vi "Beampointing_Multi_TRA.vi"() -> ()   [LabVIEW 2013]
uses:
  GUI_Template/GUI_master/tcp_new_data_event.ctl
  GUI_Template/GUI_master/tcp new data cluster.ctl
  Ctrs/beam detection.ctl
  GUI_Beampointing_single_TRA/Ctrs/move.ctl
  <vilib>/Utility/file.llb/Read From Spreadsheet File (string).vi
  <userlib>/_OpenG.lib/array/array.llb/Filter 1D Array with Scalar (String)__ogtk.vi
  <vilib>/Utility/file.llb/Write To Spreadsheet File (string).vi
  <vilib>/Analysis/NI_AALBase.lvlib
panel:
  out "size(s) 3":i32[](array[numeric])
  out "size(s) 2":i32[](array[numeric])
  out "size(s)":i32[](array[numeric])
  out "Numeric 2":i32
  out "x-y*floor(x/y)":dbl
  out "config path":string
  out "motor refs 7":refnum<vi>[](array[refnum])
  out "Moving Y":string
  out "Moving X":string
  out "particles":T1(array[cluster])
  out "motor refs 6":refnum<vi>[](array[refnum])
  out "millisecond timer value":u32
  out "motor refs 5":refnum<vi>[](array[refnum])
  out "appended path":path
  out "motor refs 4":refnum<vi>[](array[refnum])
  in  "active Axis ref 3":cluster{"Ref X":refnum<vi>, "Ref Y":refnum<vi>}
  out "motor refs 3":refnum<vi>[](array[refnum])
  in  "active man refs":cluster{"Ref X":refnum<vi>, "Ref Y":refnum<vi>}
  out "motor refs 2":refnum<vi>[](array[refnum])
  in  "Numeric":dbl
  out "Current State":string
  in  "output cluster 2":T5 {"detection para"."smal para"."Measurement Parameter" items=["Center of Mass X", "Center of Mass Y", "First Pixel X", "First Pixel Y", "Bounding Rect Left", "Bounding Rect Top", "Bounding Rect Right", "Bounding Rect Bottom", "Max Feret Diameter Start X", "Max Feret Diameter Start Y", "Max Feret Diameter End X", "Max Feret Diameter End Y", "Max Horiz. Segment Length Left", "Max Horiz. Segment Length Right", "Max Horiz. Segment Length Row", "-", "Bounding Rect Width", "Bounding Rect Height", "Bounding Rect Diagonal", "Perimeter", "Convex Hull Perimeter", "Holes' Perimeter", "Max Feret Diameter", "Equivalent Ellipse Major Axis", "Equivalent Ellipse Minor Axis", "Equivalent Ellipse Minor Axis (Feret)", "Equivalent Rect Long Side", "Equivalent Rect Short Side", "Equivalent Rect Diagonal", "Equivalent Rect Short Side (Feret)", "Average Horiz. Segment Length", "Average Vert. Segment Length", "Hydraulic Radius", "Waddel Disk Diameter", "-", "Area", "Holes' Area", "Particle & Holes' Area", "Convex Hull Area", "Image Area", "-", "Number of Holes", "Number of Horiz. Segments", "Number of Vert. Segments", "-", "Orientation", "Max Feret Diameter Orientation", "-", "% Area/Image Area", "% Area/(Particle & Holes' Area)", "Ratio of Equivalent Ellipse Axes", "Ratio of Equivalent Rect Sides", "-", "Elongation Factor", "Compactness Factor", "Heywood Circularity Factor", "Type Factor", "-", "Sum X", "Sum Y", "Sum XX", "Sum XY", "Sum YY", "Sum XXX", "Sum XXY", "Sum XYY", "Sum YYY", "-", "Moment of Inertia XX", "Moment of Inertia XY", "Moment of Inertia YY", "Moment of Inertia XXX", "Moment of Inertia XXY", "Moment of Inertia XYY", "Moment of Inertia YYY", "Norm. Moment of Inertia XX", "Norm. Moment of Inertia XY", "Norm. Moment of Inertia YY", "Norm. Moment of Inertia XXX", "Norm. Moment of Inertia XXY", "Norm. Moment of Inertia XYY", "Norm. Moment of Inertia YYY", "Hu Moment 1", "Hu Moment 2", "Hu Moment 3", "Hu Moment 4", "Hu Moment 5", "Hu Moment 6", "Hu Moment 7"]; "detection para"."smal para"."Range Lower Value" format="%.2f"; "detection para"."smal para"."Range Upper Value" format="%.2f"; "detection para"."detection method" items=["clustering", "entropy", "metric", "moments", "inter-class variance"]; "detection para"."Filter" items=["No Filter", "Median Filter", "Low Pass Filter"]}
  out "CCDs":string[](array[string])
  in  "GUIdevice 12":string
  in  "GUIdevice 11":string
  in  "GUIdevice 10":string
  in  "GUIdevice 9":string
  out "error out 2":errorcluster
  in  "active cams":string[](array[string])
  in  "Motor Y":dbl[][](array[numeric])
  in  "Motor X":dbl[][](array[numeric])
  out "Names":string[](array[string])
  in  "Offset X stats":dbl[][](array[numeric])
  in  "Offset Y stats":dbl[][](array[numeric])
  out "Box":T6(array[cluster])
  in  "Tab Control 2":enum32{"Config ", "Main", "History"}(tab)=enum."Main"
  in  "associated motors":T7 {"Motor CCD 12" items=["M20", "SIM", "M22", ""]; "Motor CCD 11" items=["M20", "SIM", "M22", ""]; "Motor CCD 10" items=["M20", "SIM", "M22", ""]; "Motor CCD 9" items=["M20", "SIM", "M22", ""]; "Motor CCD 8" items=["M20", "SIM", "M22", ""]; "Motor CCD 7" items=["M20", "SIM", "M22", ""]; "Motor CCD 6" items=["M20", "SIM", "M22", ""]; "Motor CCD 5" items=["M20", "SIM", "M22", ""]; "Motor CCD 4" items=["M20", "SIM", "M22", ""]; "Motor CCD 3" items=["M20", "SIM", "M22", ""]; "Motor CCD 2" items=["M20", "SIM", "M22", ""]; "Motor CCD 1" items=["M20", "SIM", "M22", ""]}
  out "Cameras":T8
  out "Status":cluster{i32, i32, "Centroid X":dbl[][]}(graph)
  in  "Exposure:12":dbl=0.095 min=0.0001 max=1.0 format="%#_6f"
  in  "Triggerdelay::12":dbl=0.003 min=0.0 max=0.09 format="%#_6f"
  in  "Exposure::11":dbl=0.095 min=0.0001 max=1.0 format="%#_6f"
  in  "Triggerdelay::11":dbl=0.003 min=0.0 max=0.09 format="%#_6f"
  in  "Exposure::10":dbl=0.095 min=0.0001 max=1.0 format="%#_6f"
  in  "Triggerdelay::10":dbl=0.003 min=0.0 max=0.09 format="%#_6f"
  in  "Exposure::9":dbl=0.095 min=0.0001 max=1.0 format="%#_6f"
  in  "Triggerdelay::9":dbl=0.003 min=0.0 max=0.09 format="%#_6f"
  in  "Trigger::9":bool
  in  "Trigger::10":bool caption="Trigger:10"
  in  "Trigger::11":bool
  in  "Trigger::12":bool
  in  "Target.Y::9":dbl=45.0 caption="T9y" min=0.0 max=2000.0 format="%#_6f"
  in  "Target.X::9":dbl=47.0 caption="Tx9" min=0.0 max=2000.0 format="%#_6f"
  in  "Target.Y::10":dbl=45.0 caption="T10y" min=0.0 max=2000.0 format="%#_6f"
  in  "Target.X::10":dbl=47.0 caption="T10x" min=0.0 max=2000.0 format="%#_6f"
  in  "Target.Y::11":dbl=45.0 caption="T11y" min=0.0 max=2000.0 format="%#_6f"
  in  "Target.X::11":dbl=47.0 caption="T11x" min=0.0 max=2000.0 format="%#_6f"
  in  "Target.Y::12":dbl=45.0 caption="T12y" min=0.0 max=2000.0 format="%#_6f"
  in  "Target.X::12":dbl=47.0 caption="T12x" min=0.0 max=2000.0 format="%#_6f"
  in  "Exposure::8":dbl=0.095 min=0.0001 max=1.0 format="%#_6f"
  in  "Triggerdelay::8":dbl=0.003 min=0.0 max=0.09 format="%#_6f"
  in  "Trigger::8":bool
  in  "Target.Y::8":dbl=45.0 caption="T8y" min=0.0 max=2000.0 format="%#_6f"
  in  "Target.X::8":dbl=47.0 caption="T8x" min=0.0 max=2000.0 format="%#_6f"
  in  "Target.Y::7":dbl=45.0 caption="T7x" min=0.0 max=2000.0 format="%#_6f"
  in  "Target.X::7":dbl=47.0 caption="T7y" min=0.0 max=2000.0 format="%#_6f"
  in  "Target.Y::6":dbl=45.0 caption="T6y" min=0.0 max=5000.0 format="%#_6f"
  in  "Target.X::6":dbl=47.0 caption="T6x" min=0.0 max=5000.0 format="%#_6f"
  in  "Target.Y::5":dbl=45.0 caption="T5y" min=0.0 max=5000.0 format="%#_6f"
  in  "Target.X::5":dbl=47.0 caption="T5x" min=0.0 max=5000.0 format="%#_6f"
  in  "Target.Y::4":dbl=45.0 caption="T4y" min=0.0 max=5000.0 format="%#_6f"
  in  "Target.X::4":dbl=47.0 caption="T4x" min=0.0 max=5000.0 format="%#_6f"
  in  "Target.Y::3":dbl=163.0 caption="T3y" min=0.0 max=5000.0 format="%#_6f"
  in  "Target.X::3":dbl=152.0 caption="T3x" min=0.0 max=5000.0 format="%#_6f"
  in  "Target.Y::2":dbl=74.0 caption="T2y" min=0.0 max=5000.0 format="%#_6f"
  in  "Target.X::2":dbl=75.0 caption="T2x" min=0.0 max=5000.0 format="%#_6f"
  in  "Target.Y::1":dbl=61.0 caption="T1y" min=0.0 max=5000.0 format="%#_6f"
  in  "Target.X::1":dbl=77.0 caption="T1x" min=0.0 max=5000.0 format="%#_6f"
  in  "Exposure::7":dbl=0.095 min=0.0001 max=1.0 format="%#_6f"
  in  "Triggerdelay::7":dbl=0.003 min=0.0 max=0.09 format="%#_6f"
  in  "Trigger::7":bool
  in  "Exposure::6":dbl=0.095 min=0.0001 max=1.0 format="%#_6f"
  in  "Triggerdelay::6":dbl=0.003 min=0.0 max=0.09 format="%#_6f"
  in  "Trigger::6":bool
  in  "Exposure::5":dbl=0.095 min=0.0001 max=1.0 format="%#_6f"
  in  "Triggerdelay::5":dbl=0.003 min=0.0 max=0.09 format="%#_6f"
  in  "Trigger::5":bool
  in  "Exposure::4":dbl=0.095 min=0.0001 max=1.0 format="%#_6f"
  in  "Triggerdelay::4":dbl=0.003 min=0.0 max=0.09 format="%#_6f"
  in  "Trigger::4":bool
  in  "Exposure::3":dbl=0.095 min=0.0001 max=1.0 format="%#_6f"
  in  "Triggerdelay::3":dbl=0.003 min=0.0 max=0.09 format="%#_6f"
  in  "Trigger::3":bool
  in  "Exposure::2":dbl=0.095 min=0.0001 max=1.0 format="%#_6f"
  in  "Triggerdelay::2":dbl=0.003 min=0.0 max=0.09 format="%#_6f"
  in  "Trigger::2":bool
  out "image::1":T9(plugin-control) caption="RegenCam"
  out "image::2":T9(plugin-control) caption="BoosterCam"
  out "image::3":T9(plugin-control) caption="PreampCam"
  out "image::4":T9(plugin-control) caption="Amp1Cam"
  out "image::5":T9(plugin-control) caption="Amp2Cam"
  out "image::6":T9(plugin-control) caption="Amp3Cam"
  out "image::7":T9(plugin-control)
  out "image::8":T9(plugin-control)
  in  "Exposure::1":dbl=0.095 min=0.0001 max=1.0 format="%#_6f"
  in  "Triggerdelay::1":dbl=0.003 min=0.0 max=0.09 format="%#_6f"
  in  "Trigger::1":bool
  in  "UDP error message":string
  out "required Y":bool[](array[boolean])
  out "required X":bool[](array[boolean])
  out "detected":bool[](array[boolean])
  out "name array":string[](array[string])
  out "image::9":T9(plugin-control)
  out "image::10":T9(plugin-control)
  out "image::11":T9(plugin-control)
  out "image::12":T9(plugin-control)
  out "speedmode X":bool[](array[boolean])
  out "speedmode Y":bool[](array[boolean])
  out "CCD 9":cluster{timestamp[], dbl[]}[](graph)
  out "CCD 10":cluster{timestamp[], dbl[]}[](graph)
  out "CCD 11":cluster{timestamp[], dbl[]}[](graph)
  out "CCD 12":cluster{timestamp[], dbl[]}[](graph)
  out "CCD 5":cluster{timestamp[], dbl[]}[](graph)
  out "CCD 6":cluster{timestamp[], dbl[]}[](graph)
  out "CCD 7":cluster{timestamp[], dbl[]}[](graph)
  out "CCD 8":cluster{timestamp[], dbl[]}[](graph)
  out "CCD 2":cluster{timestamp[], dbl[]}[](graph)
  out "CCD 1":cluster{timestamp[], dbl[]}[](graph)
  out "CCD 3":cluster{timestamp[], dbl[]}[](graph)
  out "CCD 4":cluster{timestamp[], dbl[]}[](graph)
  in  "History Size":i32=500
  out "History Index":i32
  in  "Feedback Global":bool
  in  "detection para":T3[](array[typedef])=[{"Filter"=1, "Filter Para"={"X Size"=5, "Y Size"=5, "% Tolerance"=1}, "detection method"=4, "smal para"=[{"Measurement Parameter"=35, "Range Lower Value"=0.0, "Range Upper Value"=0.0, "Range"=TRUE, "Measurement Type"=FALSE}], "Remove small Objects"=TRUE, "Restrict to round Objects"=FALSE}, {"Filter"=1, "Filter Para"={"X Size"=5, "Y Size"=5, "% Tolerance"=1}, "detection method"=4, "smal para"=[{"Measurement Parameter"=35, "Range Lower Value"=0.0, "Range Upper Value"=500.0, "Range"=FALSE, "Measurement Type"=FALSE}], "Remove small Objects"=TRUE, "Restrict to round Objects"=FALSE}, {"Filter"=1, "Filter Para"={"X Size"=5, "Y Size"=5, "% Tolerance"=1}, "detection method"=4, "smal para"=[{"Measurement Parameter"=35, "Range Lower Value"=0.0, "Range Upper Value"=500.0, "Range"=TRUE, "Measurement Type"=FALSE}], "Remove small Objects"=TRUE, "Restrict to round Objects"=FALSE}, {"Filter"=1, "Filter Para"={"X Size"=5, "Y Size"=5, "% Tolerance"=1}, "detection method"=4, "smal para"=[{"Measurement Parameter"=35, "Range Lower Value"=0.0, "Range Upper Value"=500.0, "Range"=TRUE, "Measurement Type"=FALSE}], "Remove small Objects"=TRUE, "Restrict to round Objects"=FALSE}, {"Filter"=1, "Filter Para"={"X Size"=5, "Y Size"=5, "% Tolerance"=1}, "detection method"=4, "smal para"=[{"Measurement Parameter"=35, "Range Lower Value"=0.0, "Range Upper Value"=500.0, "Range"=TRUE, "Measurement Type"=FALSE}], "Remove small Objects"=TRUE, "Restrict to round Objects"=FALSE}, {"Filter"=1, "Filter Para"={"X Size"=5, "Y Size"=5, "% Tolerance"=1}, "detection method"=4, "smal para"=[{"Measurement Parameter"=35, "Range Lower Value"=0.0, "Range Upper Value"=500.0, "Range"=TRUE, "Measurement Type"=FALSE}], "Remove small Objects"=TRUE, "Restrict to round Objects"=FALSE}, {"Filter"=1, "Filter Para"={"X Size"=5, "Y Size"=5, "% Tolerance"=1}, "detection method"=4, "smal para"=[{"Measurement Parameter"=35, "Range Lower Value"=0.0, "Range Upper Value"=500.0, "Range"=TRUE, "Measurement Type"=FALSE}], "Remove small Objects"=TRUE, "Restrict to round Objects"=FALSE}, {"Filter"=1, "Filter Para"={"X Size"=5, "Y Size"=5, "% Tolerance"=1}, "detection method"=3, "smal para"=[{"Measurement Parameter"=35, "Range Lower Value"=0.0, "Range Upper Value"=0.0, "Range"=FALSE, "Measurement Type"=FALSE}], "Remove small Objects"=TRUE, "Restrict to round Objects"=FALSE}, {"Filter"=1, "Filter Para"={"X Size"=5, "Y Size"=5, "% Tolerance"=1}, "detection method"=4, "smal para"=[{"Measurement Parameter"=35, "Range Lower Value"=0.0, "Range Upper Value"=0.0, "Range"=FALSE, "Measurement Type"=FALSE}], "Remove small Objects"=TRUE, "Restrict to round Objects"=FALSE}, {"Filter"=1, "Filter Para"={"X Size"=5, "Y Size"=5, "% Tolerance"=1}, "detection method"=4, "smal para"=[{"Measurement Parameter"=35, "Range Lower Value"=0.0, "Range Upper Value"=500.0, "Range"=TRUE, "Measurement Type"=FALSE}], "Remove small Objects"=TRUE, "Restrict to round Objects"=FALSE}, {"Filter"=1, "Filter Para"={"X Size"=5, "Y Size"=5, "% Tolerance"=1}, "detection method"=4, "smal para"=[{"Measurement Parameter"=35, "Range Lower Value"=0.0, "Range Upper Value"=500.0, "Range"=TRUE, "Measurement Type"=FALSE}], "Remove small Objects"=TRUE, "Restrict to round Objects"=FALSE}, {"Filter"=1, "Filter Para"={"X Size"=5, "Y Size"=5, "% Tolerance"=1}, "detection method"=4, "smal para"=[{"Measurement Parameter"=35, "Range Lower Value"=0.0, "Range Upper Value"=500.0, "Range"=TRUE, "Measurement Type"=FALSE}], "Remove small Objects"=TRUE, "Restrict to round Objects"=FALSE}] {"smal para"."Measurement Parameter" items=["Center of Mass X", "Center of Mass Y", "First Pixel X", "First Pixel Y", "Bounding Rect Left", "Bounding Rect Top", "Bounding Rect Right", "Bounding Rect Bottom", "Max Feret Diameter Start X", "Max Feret Diameter Start Y", "Max Feret Diameter End X", "Max Feret Diameter End Y", "Max Horiz. Segment Length Left", "Max Horiz. Segment Length Right", "Max Horiz. Segment Length Row", "-", "Bounding Rect Width", "Bounding Rect Height", "Bounding Rect Diagonal", "Perimeter", "Convex Hull Perimeter", "Holes' Perimeter", "Max Feret Diameter", "Equivalent Ellipse Major Axis", "Equivalent Ellipse Minor Axis", "Equivalent Ellipse Minor Axis (Feret)", "Equivalent Rect Long Side", "Equivalent Rect Short Side", "Equivalent Rect Diagonal", "Equivalent Rect Short Side (Feret)", "Average Horiz. Segment Length", "Average Vert. Segment Length", "Hydraulic Radius", "Waddel Disk Diameter", "-", "Area", "Holes' Area", "Particle & Holes' Area", "Convex Hull Area", "Image Area", "-", "Number of Holes", "Number of Horiz. Segments", "Number of Vert. Segments", "-", "Orientation", "Max Feret Diameter Orientation", "-", "% Area/Image Area", "% Area/(Particle & Holes' Area)", "Ratio of Equivalent Ellipse Axes", "Ratio of Equivalent Rect Sides", "-", "Elongation Factor", "Compactness Factor", "Heywood Circularity Factor", "Type Factor", "-", "Sum X", "Sum Y", "Sum XX", "Sum XY", "Sum YY", "Sum XXX", "Sum XXY", "Sum XYY", "Sum YYY", "-", "Moment of Inertia XX", "Moment of Inertia XY", "Moment of Inertia YY", "Moment of Inertia XXX", "Moment of Inertia XXY", "Moment of Inertia XYY", "Moment of Inertia YYY", "Norm. Moment of Inertia XX", "Norm. Moment of Inertia XY", "Norm. Moment of Inertia YY", "Norm. Moment of Inertia XXX", "Norm. Moment of Inertia XXY", "Norm. Moment of Inertia XYY", "Norm. Moment of Inertia YYY", "Hu Moment 1", "Hu Moment 2", "Hu Moment 3", "Hu Moment 4", "Hu Moment 5", "Hu Moment 6", "Hu Moment 7"]; "smal para"."Range Lower Value" format="%.2f"; "smal para"."Range Upper Value" format="%.2f"; "detection method" items=["clustering", "entropy", "metric", "moments", "inter-class variance"]; "Filter" items=["No Filter", "Median Filter", "Low Pass Filter"]}
  in  "GUIdevice 8":string
  in  "Tab Control":T10(tab)=enum."Detection"
  in  "new tdms":bool
  in  "Save Stats":bool
  in  "Save Config":bool
  in  "Load Config":bool
  in  "update speed [ms]":i32=200
  in  "img to avg":i32=10
  in  "Reset History":bool
  in  "save path":path=path "W:/BP_DATA"
  in  "autodetect":bool
  in  "Detection Rate":dbl=0.9 min=0.001 max=1.0
  in  "Center":bool
  in  "Align":bool
  in  "Speedmode @":dbl=3.0 min=1.0 max=20.0
  in  "device ini":bool
  in  "beam detection para":T3={"Filter"=1, "Filter Para"={"X Size"=5, "Y Size"=5, "% Tolerance"=1}, "detection method"=4, "smal para"=[{"Measurement Parameter"=35, "Range Lower Value"=0.0, "Range Upper Value"=500.0, "Range"=FALSE, "Measurement Type"=FALSE}], "Remove small Objects"=TRUE, "Restrict to round Objects"=FALSE} {"smal para"."Measurement Parameter" items=["Center of Mass X", "Center of Mass Y", "First Pixel X", "First Pixel Y", "Bounding Rect Left", "Bounding Rect Top", "Bounding Rect Right", "Bounding Rect Bottom", "Max Feret Diameter Start X", "Max Feret Diameter Start Y", "Max Feret Diameter End X", "Max Feret Diameter End Y", "Max Horiz. Segment Length Left", "Max Horiz. Segment Length Right", "Max Horiz. Segment Length Row", "-", "Bounding Rect Width", "Bounding Rect Height", "Bounding Rect Diagonal", "Perimeter", "Convex Hull Perimeter", "Holes' Perimeter", "Max Feret Diameter", "Equivalent Ellipse Major Axis", "Equivalent Ellipse Minor Axis", "Equivalent Ellipse Minor Axis (Feret)", "Equivalent Rect Long Side", "Equivalent Rect Short Side", "Equivalent Rect Diagonal", "Equivalent Rect Short Side (Feret)", "Average Horiz. Segment Length", "Average Vert. Segment Length", "Hydraulic Radius", "Waddel Disk Diameter", "-", "Area", "Holes' Area", "Particle & Holes' Area", "Convex Hull Area", "Image Area", "-", "Number of Holes", "Number of Horiz. Segments", "Number of Vert. Segments", "-", "Orientation", "Max Feret Diameter Orientation", "-", "% Area/Image Area", "% Area/(Particle & Holes' Area)", "Ratio of Equivalent Ellipse Axes", "Ratio of Equivalent Rect Sides", "-", "Elongation Factor", "Compactness Factor", "Heywood Circularity Factor", "Type Factor", "-", "Sum X", "Sum Y", "Sum XX", "Sum XY", "Sum YY", "Sum XXX", "Sum XXY", "Sum XYY", "Sum YYY", "-", "Moment of Inertia XX", "Moment of Inertia XY", "Moment of Inertia YY", "Moment of Inertia XXX", "Moment of Inertia XXY", "Moment of Inertia XYY", "Moment of Inertia YYY", "Norm. Moment of Inertia XX", "Norm. Moment of Inertia XY", "Norm. Moment of Inertia YY", "Norm. Moment of Inertia XXX", "Norm. Moment of Inertia XXY", "Norm. Moment of Inertia XYY", "Norm. Moment of Inertia YYY", "Hu Moment 1", "Hu Moment 2", "Hu Moment 3", "Hu Moment 4", "Hu Moment 5", "Hu Moment 6", "Hu Moment 7"]; "smal para"."Range Lower Value" format="%.2f"; "smal para"."Range Upper Value" format="%.2f"; "detection method" items=["clustering", "entropy", "metric", "moments", "inter-class variance"]; "Filter" items=["No Filter", "Median Filter", "Low Pass Filter"]}
  in  "move config":T2={"Tolerance [%]"=0.1, "Stepsize"=0.0001, "Invert Axis"=TRUE, "Invert Direction X"=FALSE, "Invert Direction Y"=TRUE, "enable feedback"=FALSE, "Set Centriod Target"=FALSE}
  in  "Position 2":dbl=0.001 caption="Stepsize" min=0.0 max=999999.0 format="%_6f"
  in  "Position 1":dbl=0.001 caption="Stepsize" min=0.0 max=999999.0 format="%_6f"
  in  "Right":bool caption="RelativeMove.Axis 1.CCW::1"
  in  "Left":bool caption="RelativeMove.Axis 1.CW::1"
  in  "Down":bool caption="RelativeMove.Axis. 2.CCW::1"
  in  "Up":bool caption="RelativeMove.Axis 2.CW::1"
  in  "StepSize":dbl=0.001 caption="Stepsize" min=0.0 max=999999.0 format="%_1p"
  in  "active axis refs 2":T11(array[cluster])
  in  "active Axis ref":cluster{"Ref X":refnum<vi>, "Ref Y":refnum<vi>}
  in  "CCDs":u16(ring) items=["RegenCam", "BoosterCam", "PreampCam", "Amp1Cam", "Amp2Cam", "Amp3Cam", "", "", "", "", "", ""]
  out "motor refs":refnum<vi>[](array[refnum])
  in  "Position.Axis 4::99":dbl=77.0 caption="Motor Axis 1" min=0.0 max=6.0 format="%#_6f"
  in  "Position.Axis 5::99":dbl=77.0 caption="Motor Axis 1" min=0.0 max=6.0 format="%#_6f"
  in  "Position.Axis 6::99":dbl=77.0 caption="Motor Axis 1" min=0.0 max=6.0 format="%#_6f"
  in  "Position.Axis 3::99":dbl=77.0 caption="Motor Axis 1" min=0.0 max=6.0 format="%#_6f"
  in  "Position.Axis 2::99":dbl=77.0 caption="Motor Axis 1" min=0.0 max=6.0 format="%#_6f"
  in  "Position.Axis 1::99":dbl=77.0 caption="Motor Axis 1" min=0.0 max=6.0 format="%#_6f"
  in  "GUIdevice 99":string="TREX TRA1"
  in  "move properties":T2[](array[typedef])=[{"Tolerance [%]"=0.1, "Stepsize"=0.0001, "Invert Axis"=TRUE, "Invert Direction X"=FALSE, "Invert Direction Y"=TRUE, "enable feedback"=FALSE, "Set Centriod Target"=FALSE}, {"Tolerance [%]"=0.1, "Stepsize"=0.0001, "Invert Axis"=TRUE, "Invert Direction X"=FALSE, "Invert Direction Y"=TRUE, "enable feedback"=FALSE, "Set Centriod Target"=FALSE}, {"Tolerance [%]"=0.1, "Stepsize"=0.0001, "Invert Axis"=TRUE, "Invert Direction X"=FALSE, "Invert Direction Y"=TRUE, "enable feedback"=FALSE, "Set Centriod Target"=FALSE}, {"Tolerance [%]"=0.1, "Stepsize"=0.0001, "Invert Axis"=TRUE, "Invert Direction X"=FALSE, "Invert Direction Y"=TRUE, "enable feedback"=FALSE, "Set Centriod Target"=FALSE}, {"Tolerance [%]"=0.1, "Stepsize"=0.0001, "Invert Axis"=TRUE, "Invert Direction X"=FALSE, "Invert Direction Y"=TRUE, "enable feedback"=FALSE, "Set Centriod Target"=FALSE}, {"Tolerance [%]"=0.1, "Stepsize"=0.0001, "Invert Axis"=TRUE, "Invert Direction X"=FALSE, "Invert Direction Y"=TRUE, "enable feedback"=FALSE, "Set Centriod Target"=FALSE}, {"Tolerance [%]"=0.1, "Stepsize"=0.0001, "Invert Axis"=TRUE, "Invert Direction X"=FALSE, "Invert Direction Y"=TRUE, "enable feedback"=FALSE, "Set Centriod Target"=FALSE}, {"Tolerance [%]"=0.1, "Stepsize"=0.0001, "Invert Axis"=TRUE, "Invert Direction X"=FALSE, "Invert Direction Y"=TRUE, "enable feedback"=FALSE, "Set Centriod Target"=FALSE}, {"Tolerance [%]"=0.1, "Stepsize"=0.0001, "Invert Axis"=TRUE, "Invert Direction X"=FALSE, "Invert Direction Y"=TRUE, "enable feedback"=FALSE, "Set Centriod Target"=FALSE}, {"Tolerance [%]"=0.1, "Stepsize"=0.0001, "Invert Axis"=TRUE, "Invert Direction X"=FALSE, "Invert Direction Y"=TRUE, "enable feedback"=FALSE, "Set Centriod Target"=FALSE}, {"Tolerance [%]"=0.1, "Stepsize"=0.0001, "Invert Axis"=TRUE, "Invert Direction X"=FALSE, "Invert Direction Y"=TRUE, "enable feedback"=FALSE, "Set Centriod Target"=FALSE}, {"Tolerance [%]"=0.1, "Stepsize"=0.0001, "Invert Axis"=TRUE, "Invert Direction X"=FALSE, "Invert Direction Y"=TRUE, "enable feedback"=FALSE, "Set Centriod Target"=FALSE}, {"Tolerance [%]"=0.1, "Stepsize"=0.0001, "Invert Axis"=TRUE, "Invert Direction X"=FALSE, "Invert Direction Y"=TRUE, "enable feedback"=FALSE, "Set Centriod Target"=FALSE}]
  in  "Time":timestamp[][](array[timestamp])
  in  "Mean Size":dbl[][](array[numeric])
  in  "Size":dbl[][](array[numeric])
  in  "active CCDs":i32(listbox)
  in  "Offset Y":dbl[][](array[numeric])
  in  "Offset X":dbl[][](array[numeric])
  in  "Mean Centroid X":dbl[][](array[numeric])
  in  "Mean Centroid Y":dbl[][](array[numeric])
  in  "Centroid Y":dbl[][](array[numeric])
  in  "Centroid X":dbl[][](array[numeric])
  in  "GUIdevice 7":string
  in  "GUIdevice 6":string
  in  "GUIdevice 5":string
  in  "GUIdevice 4":string
  in  "GUIdevice 3":string="TargetCam10Hz_Diode"
  in  "GUIdevice 2":string="StagingM1Far"
  in  "insert tag":bool=TRUE
  in  "stop":bool
  in  "GUIdevice 1":string="StagingM1Near"
  out "tcp data event":T12
  out "error IO 2":errorcluster
  # "x [Tolerance]"
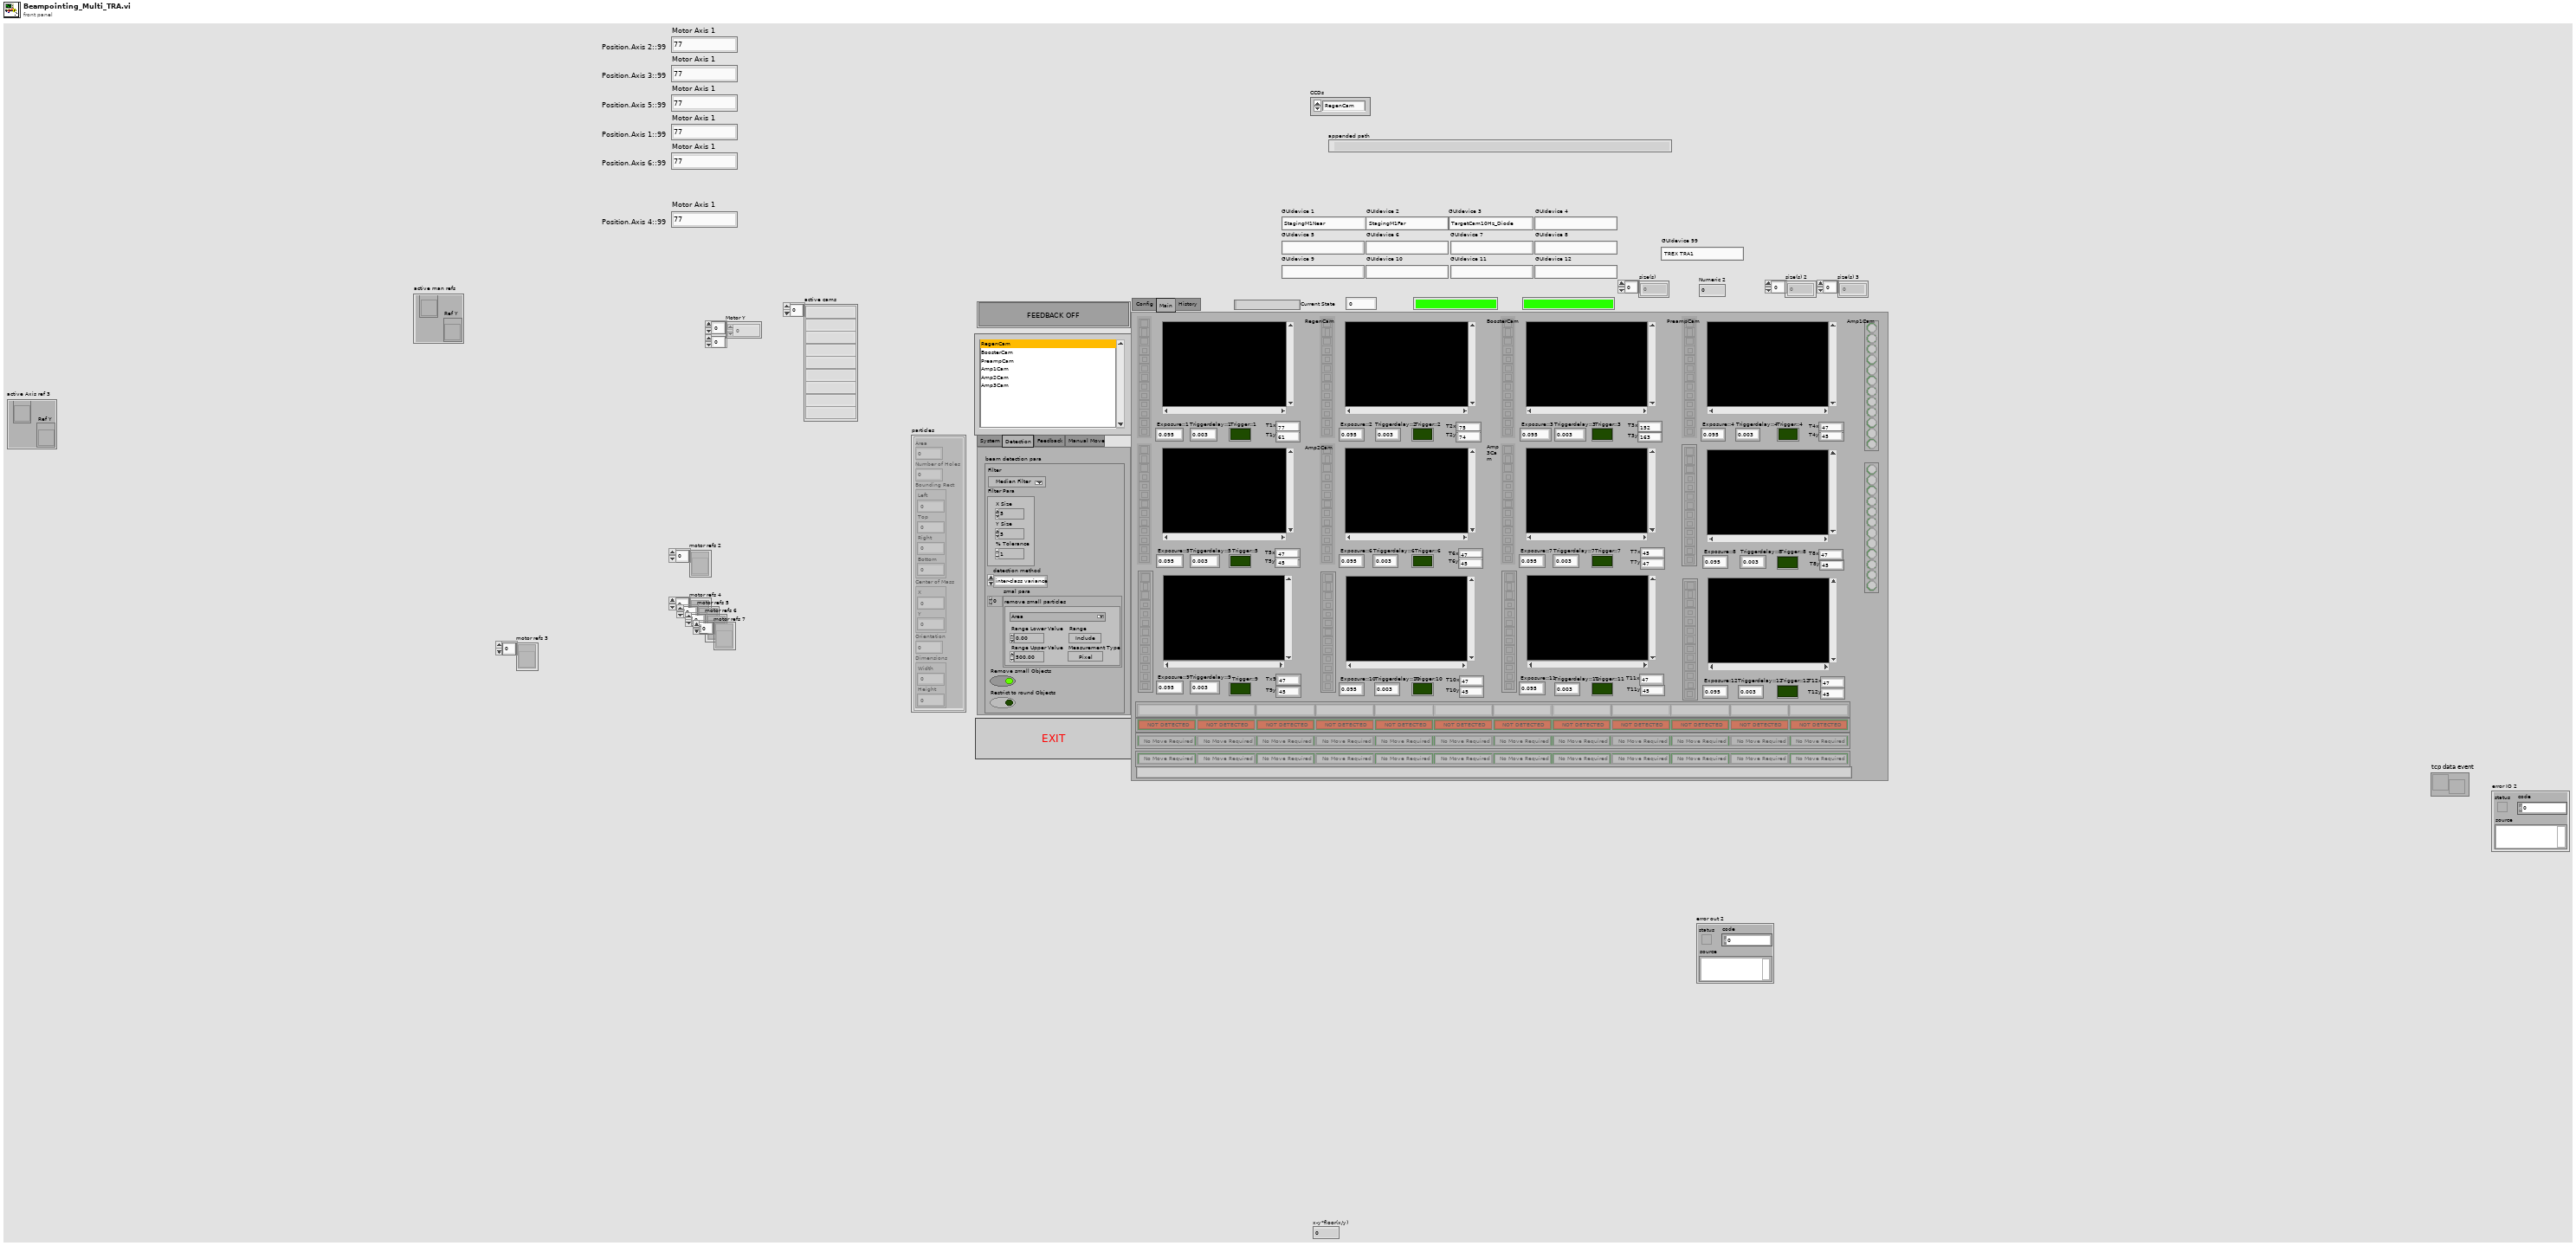
[diagram p1: front panel]
types:
  T1 = cluster{"Area":dbl, "Number of Holes":dbl, "Bounding Rect":cluster{"Left":dbl, "Top":dbl, "Right":dbl, "Bottom":dbl}, "Center of Mass":cluster{"X":dbl, "Y":dbl}, "Orientation":dbl, "Dimensions":cluster{"Width":dbl, "Height":dbl}}[]
  T2 = typedef "move.ctl" = cluster{"Tolerance [%]":dbl, "Stepsize":dbl, "Invert Axis":bool, "Invert Direction X":bool, "Invert Direction Y":bool, "enable feedback":bool, "Set Centriod Target":bool}
  T3 = typedef "beam detection.ctl" = cluster{"Filter":u16, "Filter Para":cluster{"X Size":i32, "Y Size":i32, "% Tolerance":i32}, "detection method":i32, "smal para":cluster{"Measurement Parameter":T4, "Range Lower Value":dbl, "Range Upper Value":dbl, "Range":bool, "Measurement Type":bool}[], "Remove small Objects":bool, "Restrict to round Objects":bool}
  T4 = typedef "Particle Parameters" = i32
  T5 = cluster{"CCDs":string[], "move properties":T2[], "detection para":T3[], "thresholds":cluster{"Lower value":sgl, "Upper value":sgl}[], "Value":cluster{"Motor CCD 1":u16, "Motor CCD 2":u16, "Motor CCD 3":u16, "Motor CCD 4":u16, "Motor CCD 5":u16, "Motor CCD 6":u16, "Motor CCD 7":u16, "Motor CCD 8":u16, "Motor CCD 9":u16, "Motor CCD 10":u16, "Motor CCD 11":u16, "Motor CCD 12":u16}}
  T6 = cluster{"Left":dbl, "Top":dbl, "Right":dbl, "Bottom":dbl}[]
  T7 = cluster{"Motor CCD 1":u16, "Motor CCD 2":u16, "Motor CCD 3":u16, "Motor CCD 4":u16, "Motor CCD 5":u16, "Motor CCD 6":u16, "Motor CCD 7":u16, "Motor CCD 8":u16, "Motor CCD 9":u16, "Motor CCD 10":u16, "Motor CCD 11":u16, "Motor CCD 12":u16}
  T8 = cluster{"[0]":string, "[1]":string, "[2]":string, "[3]":string, "[4]":string, "[5]":string, "[6]":string, "[7]":string, "[8]":string, "[8] 2":string, "[8] 3":string, "[8] 4":string}
  T9 = typedef "IMAQ Image.ctl" = refnum<image>
  T10 = enum32{"System", "Detection", "Feedback", "Manual Move"}
  T11 = cluster{"Ref X":refnum<vi>, "Ref Y":refnum<vi>}[]
  T12 = typedef "tcp_new_data_event.ctl" = refnum<user-event>
  T13 = typedef "tcp new data cluster.ctl" = cluster{"EventEnum":enum16{"new data", "connection status update"}, "Device name":string}
  T14 = cluster{"Left":i32, "Top":i32, "Right":i32, "Bottom":i32}
  T15 = enum32{"invalid app kind", "Development System", "Run Time System", "Student Edition", "Embedded LabVIEW", "Evaluation", "Custom"}
  T16 = enum16{"open", "open or create", "create or replace", "create", "open (read-only)"}
  T17 = enum32{"Invalid", "Standard", "Closed", "Hidden", "Minimized", "Maximized"}
  T18 = enum16{"open", "replace", "create", "open or create", "replace or create", "replace or create with confirmation"}
  T19 = enum8{"Enabled", "Disabled", "Disabled and Grayed Out"}
  T20 = typedef "Image Type" = u32
  T21 = cluster{"[0]":string, "[1]":string, "[2]":string, "[3]":string, "[4]":string, "[5]":string, "[6]":string, "[7]":string, "[8]":string, "[9]":string, "[10]":string, "[11]":string}
  T22 = cluster{"Target.X::1":refnum<vi>, "Target.Y::1":refnum<vi>}
  T23 = cluster{"Target.X::2":refnum<vi>, "Target.Y::2":refnum<vi>}
  T24 = cluster{"Target.X::3":refnum<vi>, "Target.Y::3":refnum<vi>}
  T25 = cluster{"Target.X::4":refnum<vi>, "Target.Y::4":refnum<vi>}
  T26 = cluster{"Target.X::5":refnum<vi>, "Target.Y::5":refnum<vi>}
  T27 = cluster{"Target.X::6":refnum<vi>, "Target.Y::6":refnum<vi>}
  T28 = cluster{"Target.X::7":refnum<vi>, "Target.Y::7":refnum<vi>}
  T29 = cluster{"Target.X::8":refnum<vi>, "Target.Y::8":refnum<vi>}
  T30 = cluster{"Target.X::12":refnum<vi>, "Target.Y::12":refnum<vi>}
  T31 = cluster{"Target.X::9":refnum<vi>, "Target.Y::9":refnum<vi>}
  T32 = cluster{"Target.X::10":refnum<vi>, "Target.Y::10":refnum<vi>}
  T33 = cluster{"Target.X::11":refnum<vi>, "Target.Y::11":refnum<vi>}
  T34 = cluster{"Target.X::12":refnum<vi>, "Target.Y::12":refnum<vi>}[]
  T35 = cluster{"Left":dbl, "Top":dbl, "Right":dbl, "Bottom":dbl}
  T36 = cluster{"Core":cluster{"Current VI Reference":refnum<vi>, "Close Panel on Exit?":bool}, "detection para":T3[], "thresholds":cluster{"Lower value":sgl, "Upper value":sgl}[], "Centroid X":dbl[][], "Centroid Y":dbl[][], "img to avg":i32, "Mean Centroid X":dbl[][], "Mean Centroid Y":dbl[][], "Offset X":dbl[][], "Offset Y":dbl[][], "Offset X stats ":dbl[][], "Offset Y stats ":dbl[][], "Size":dbl[][], "Mean Size":dbl[][], "Time":timestamp[][], "move properties":T2[], "active axis refs 2":cluster{"Ref X":refnum<vi>, "Ref Y":refnum<vi>}[], "active ccd":i32, "Feedback global":bool, "Motor X":dbl[][], "Motor Y":dbl[][], "active cams":string[], "Data Value Reference out":refnum<k34>, "active man refs":cluster{"Ref X":refnum<vi>, "Ref Y":refnum<vi>}, "speedmode X":bool[], "speedmode Y":bool[]}
  T37 = cluster{"Current VI Reference":refnum<vi>, "Close Panel on Exit?":bool}
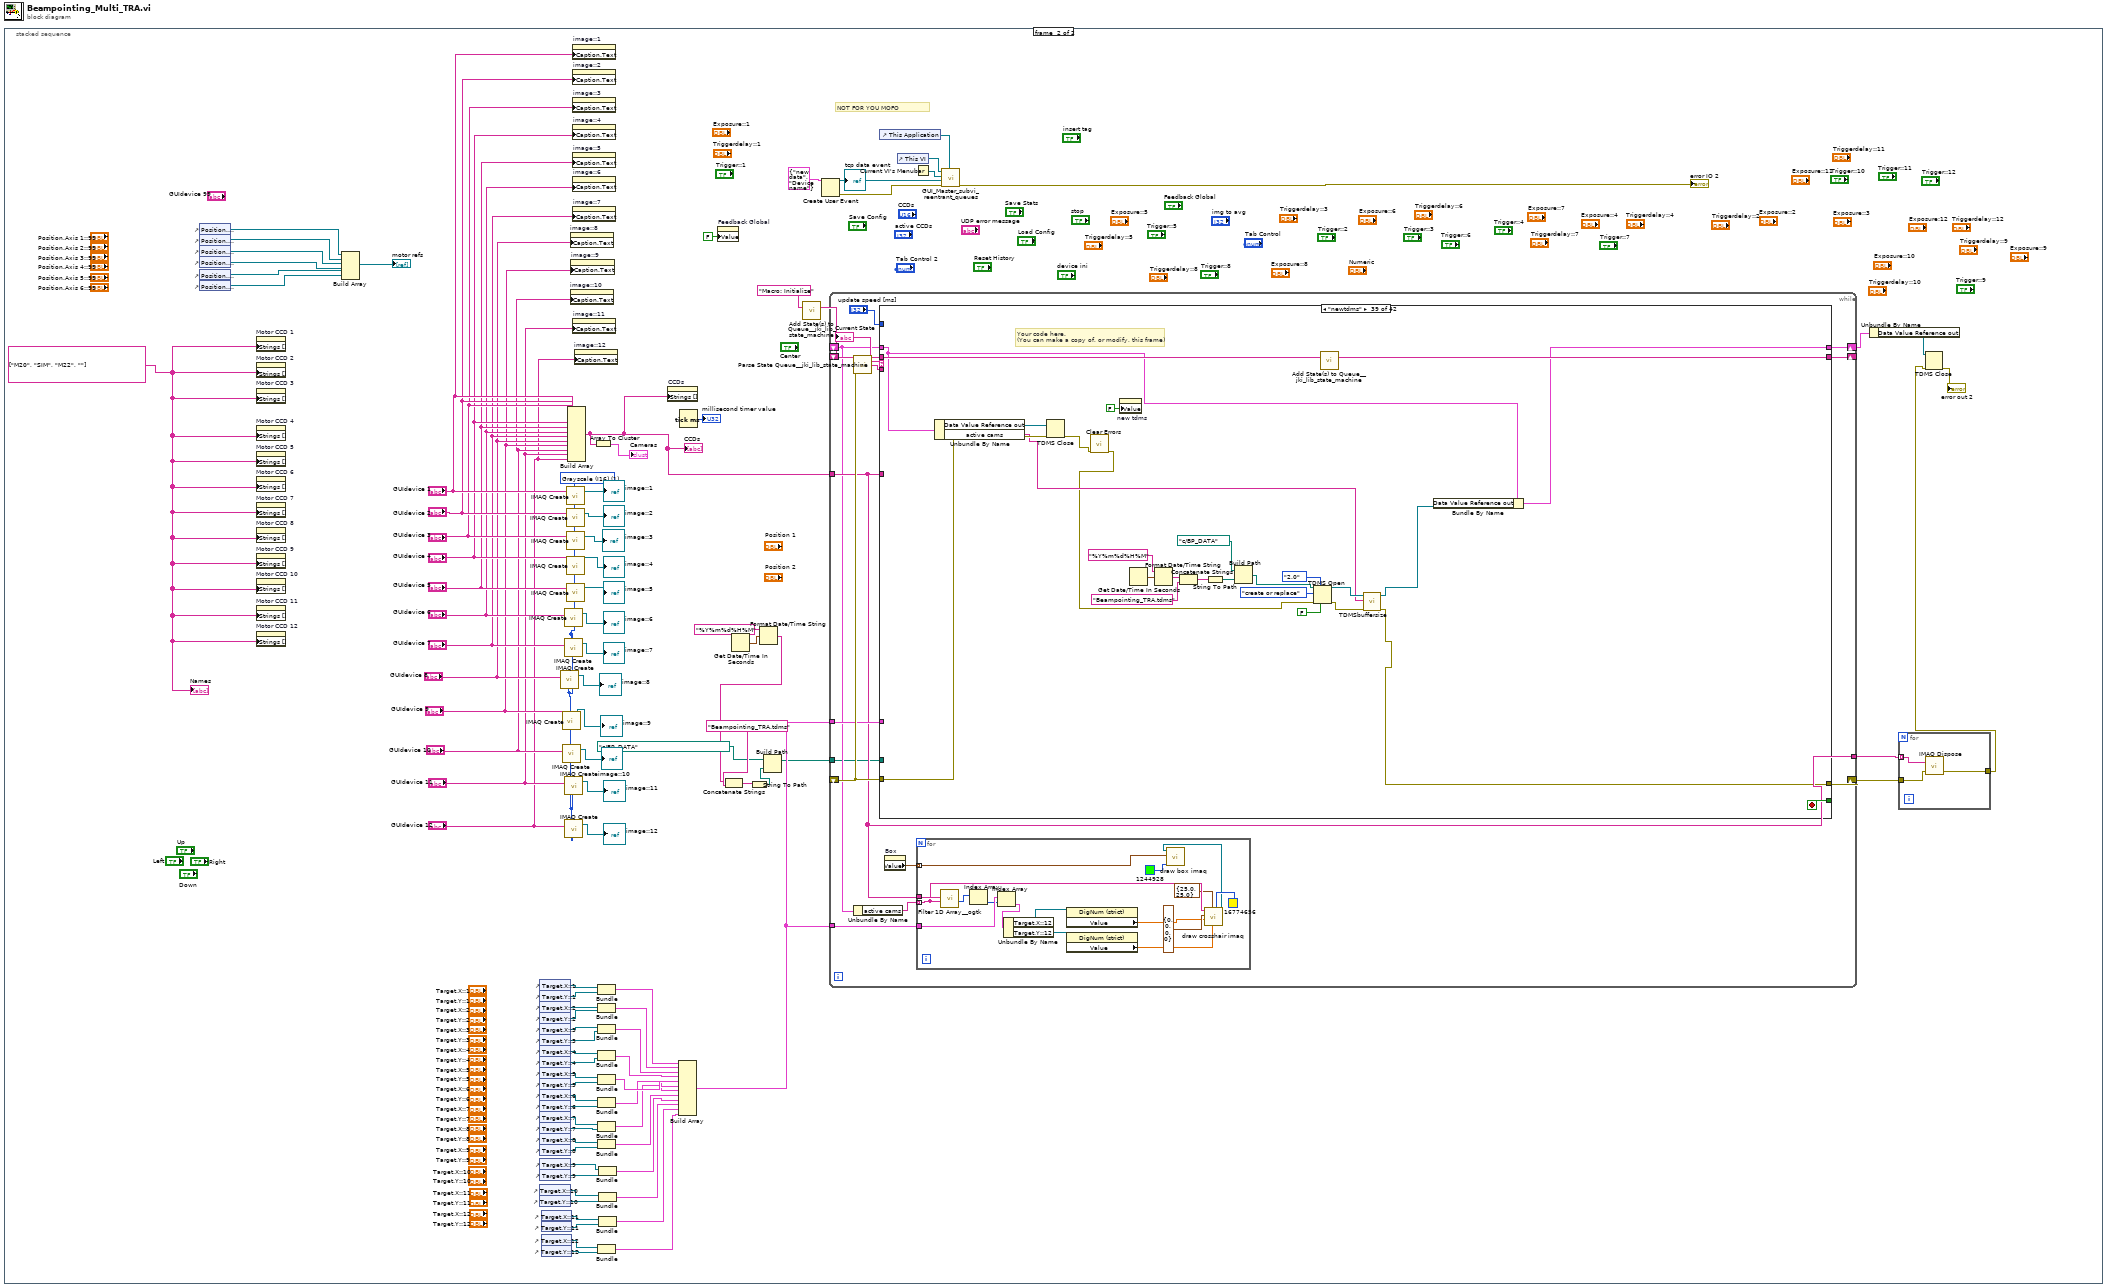
[diagram p0: block diagram]
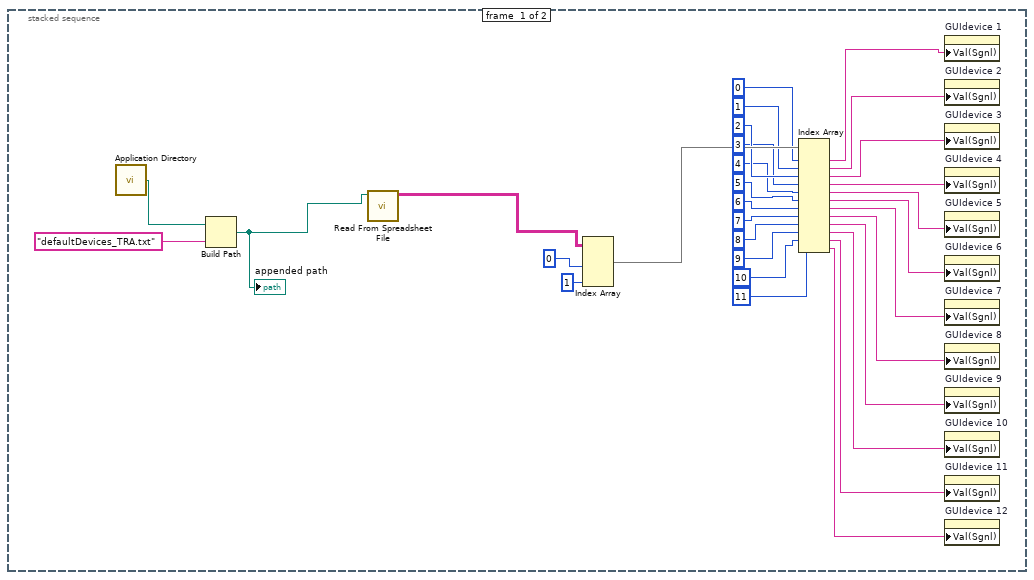
[diagram p2: hidden frame]
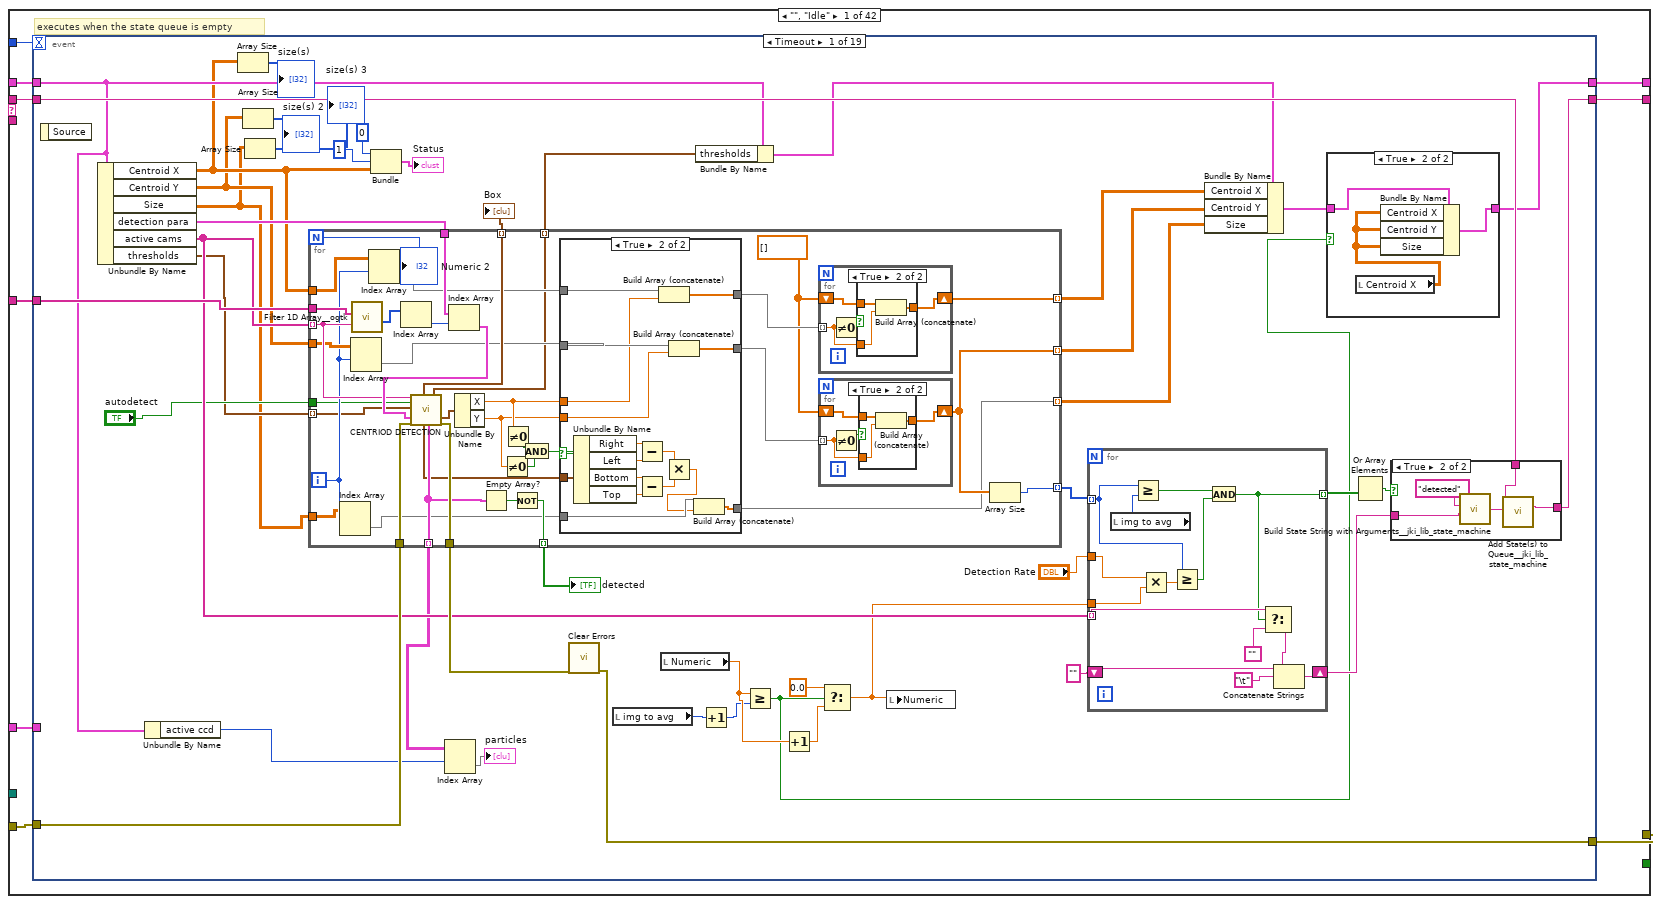
[diagram p3: hidden frame]
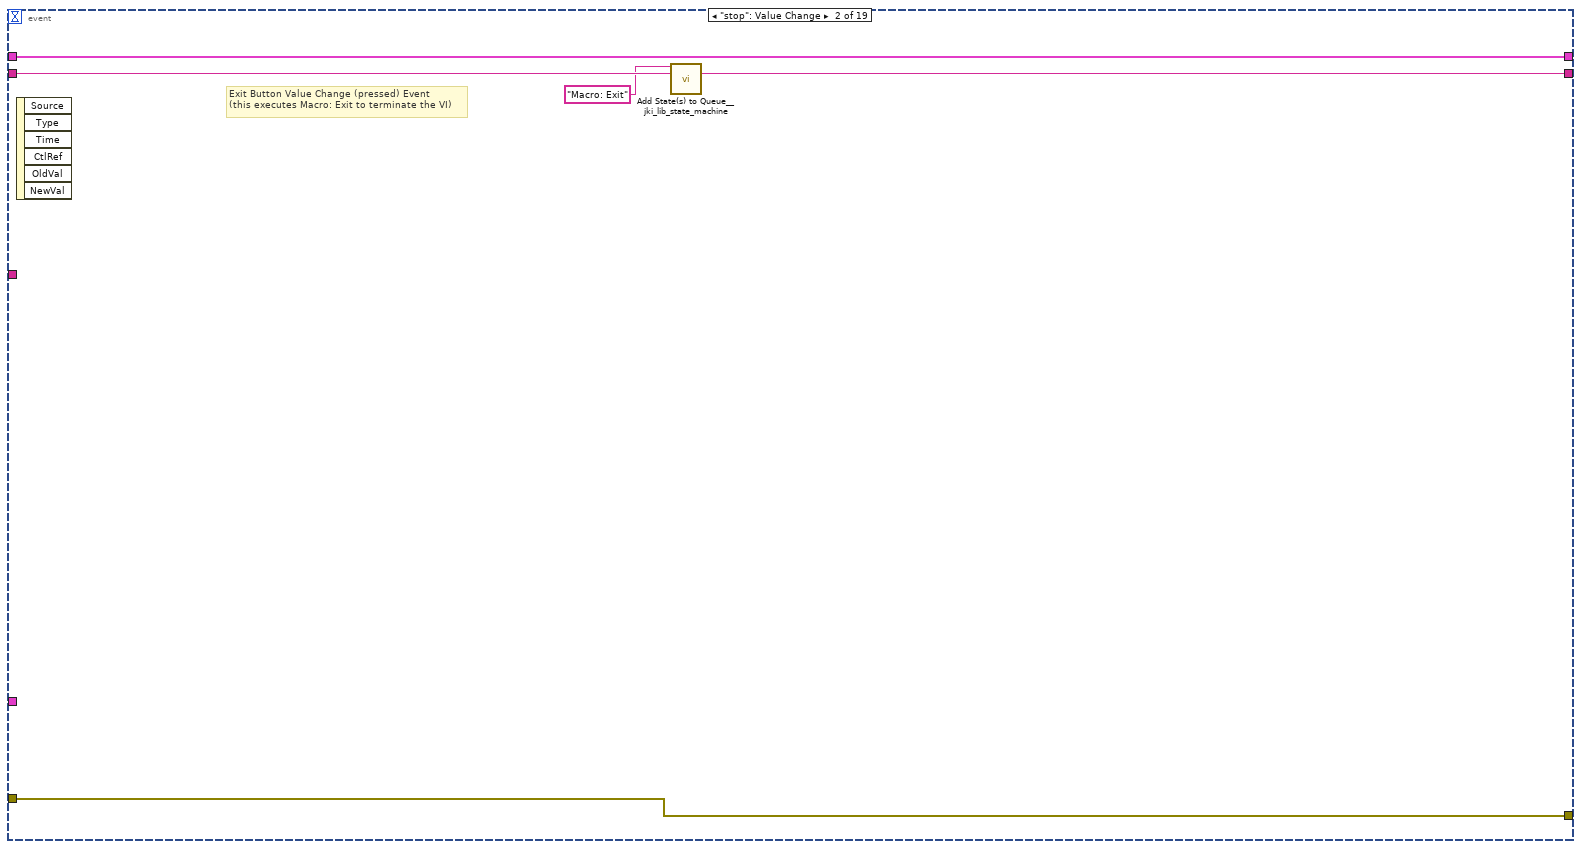
[diagram p9: hidden frame]
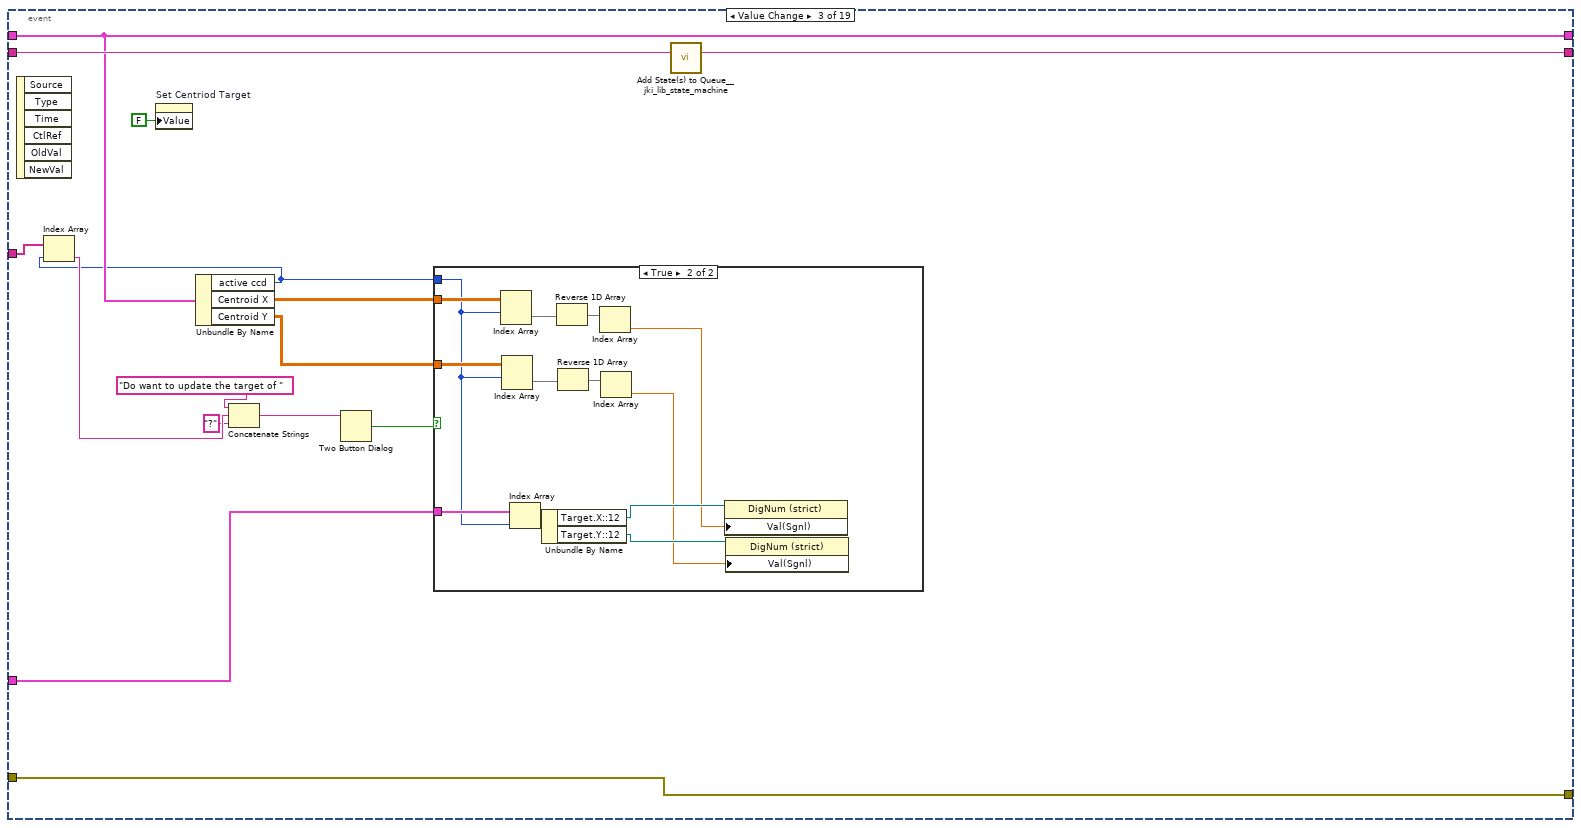
[diagram p10: hidden frame]
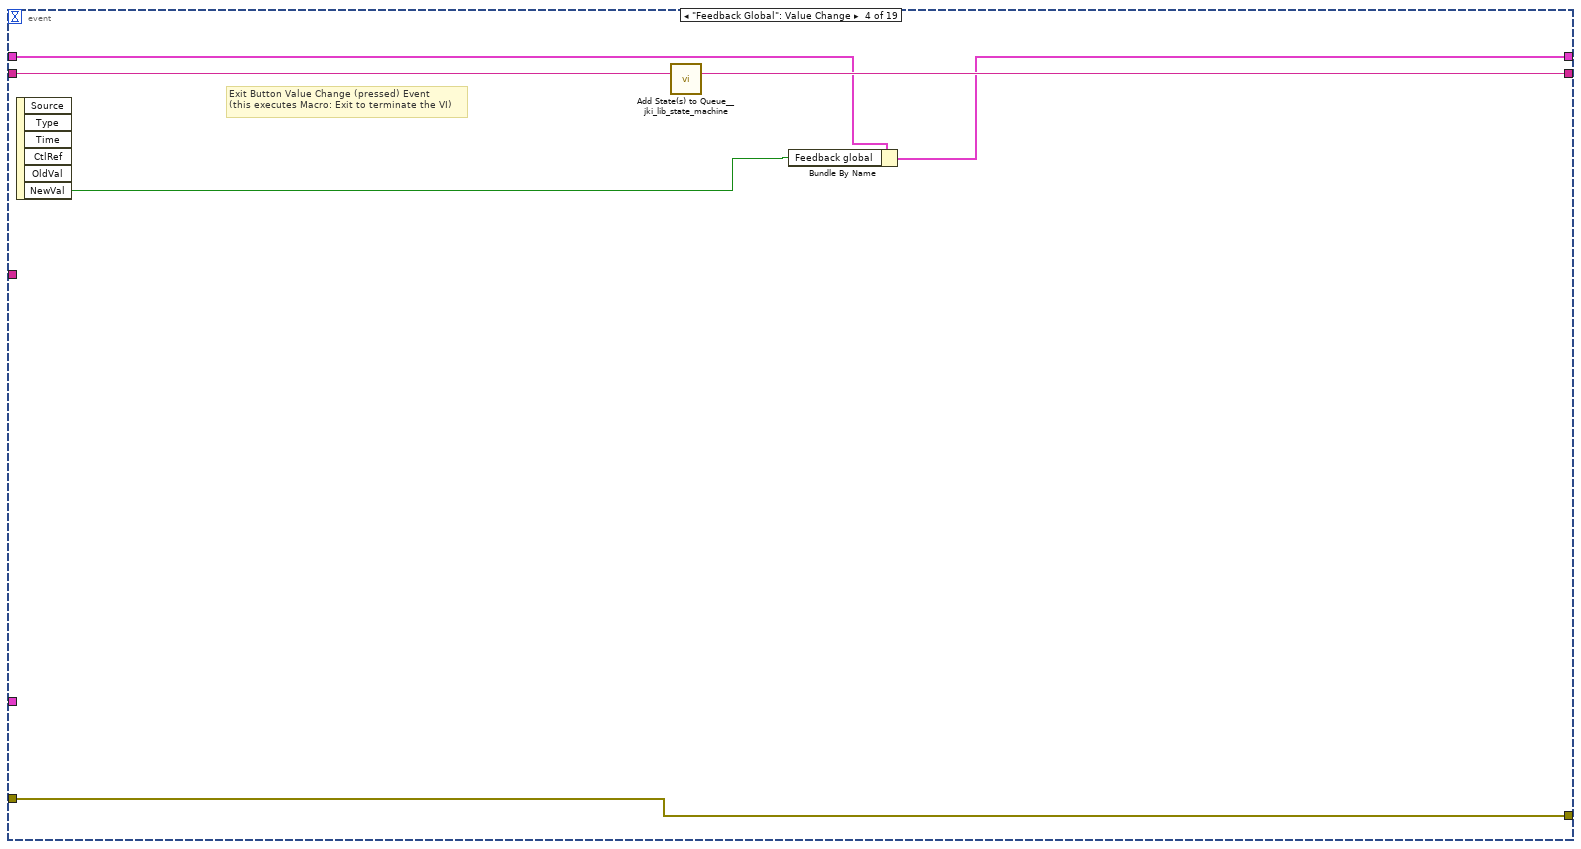
[diagram p12: hidden frame]
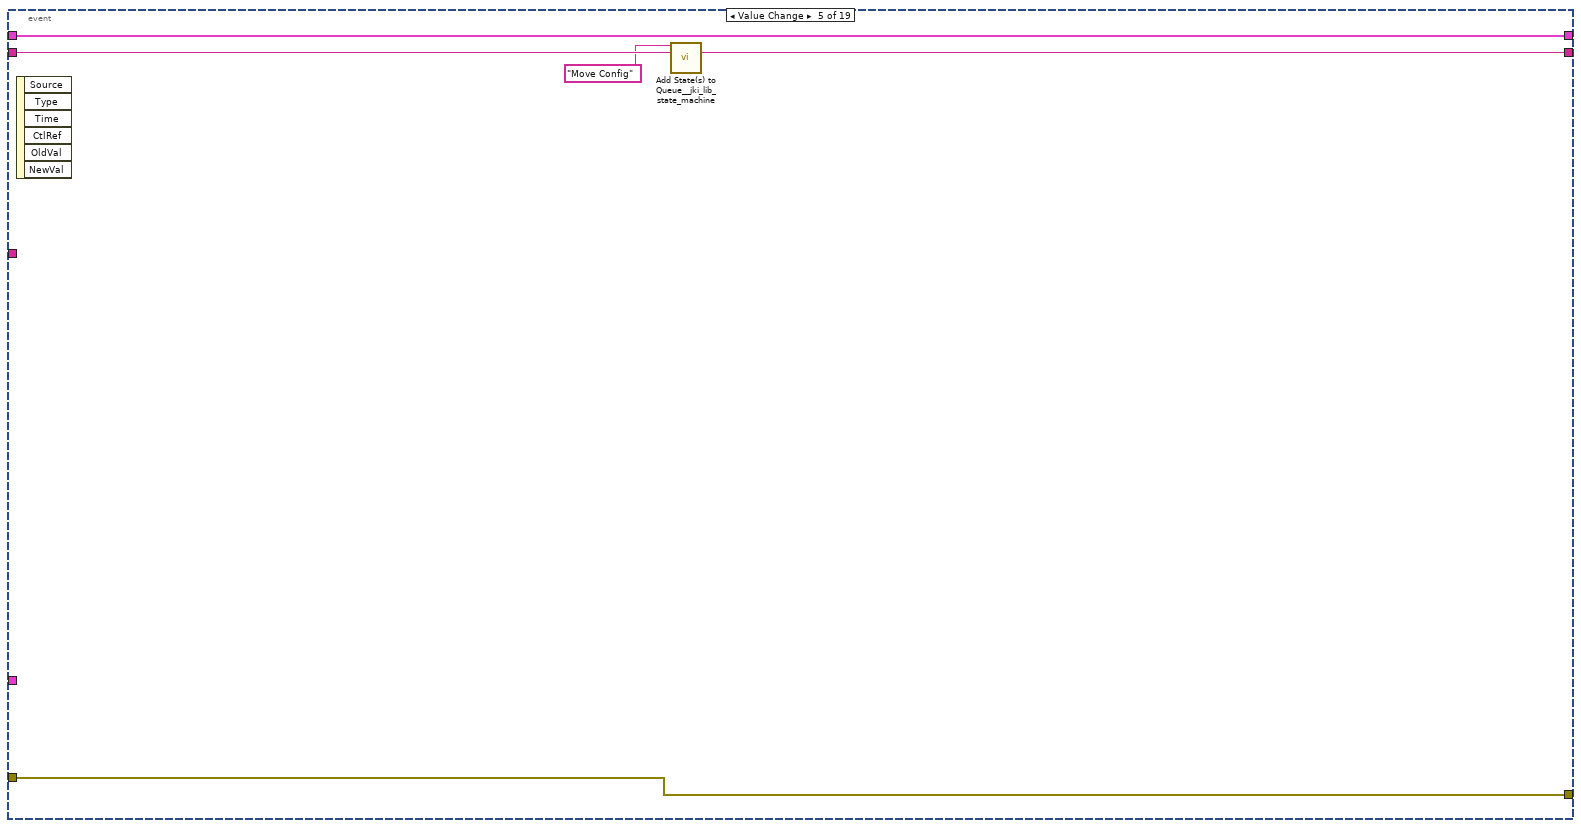
[diagram p13: hidden frame]
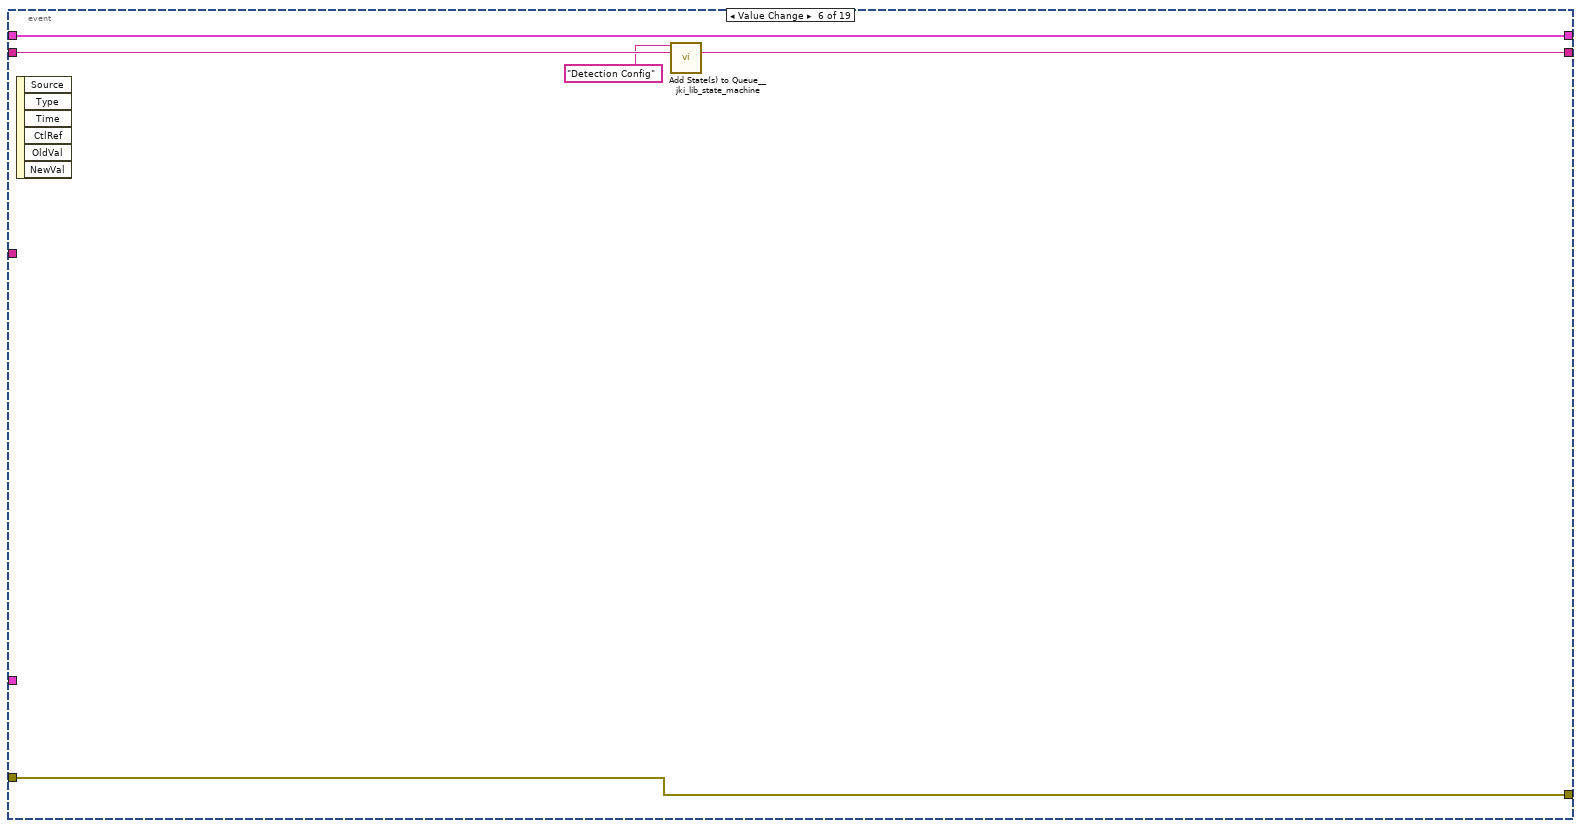
[diagram p14: hidden frame]
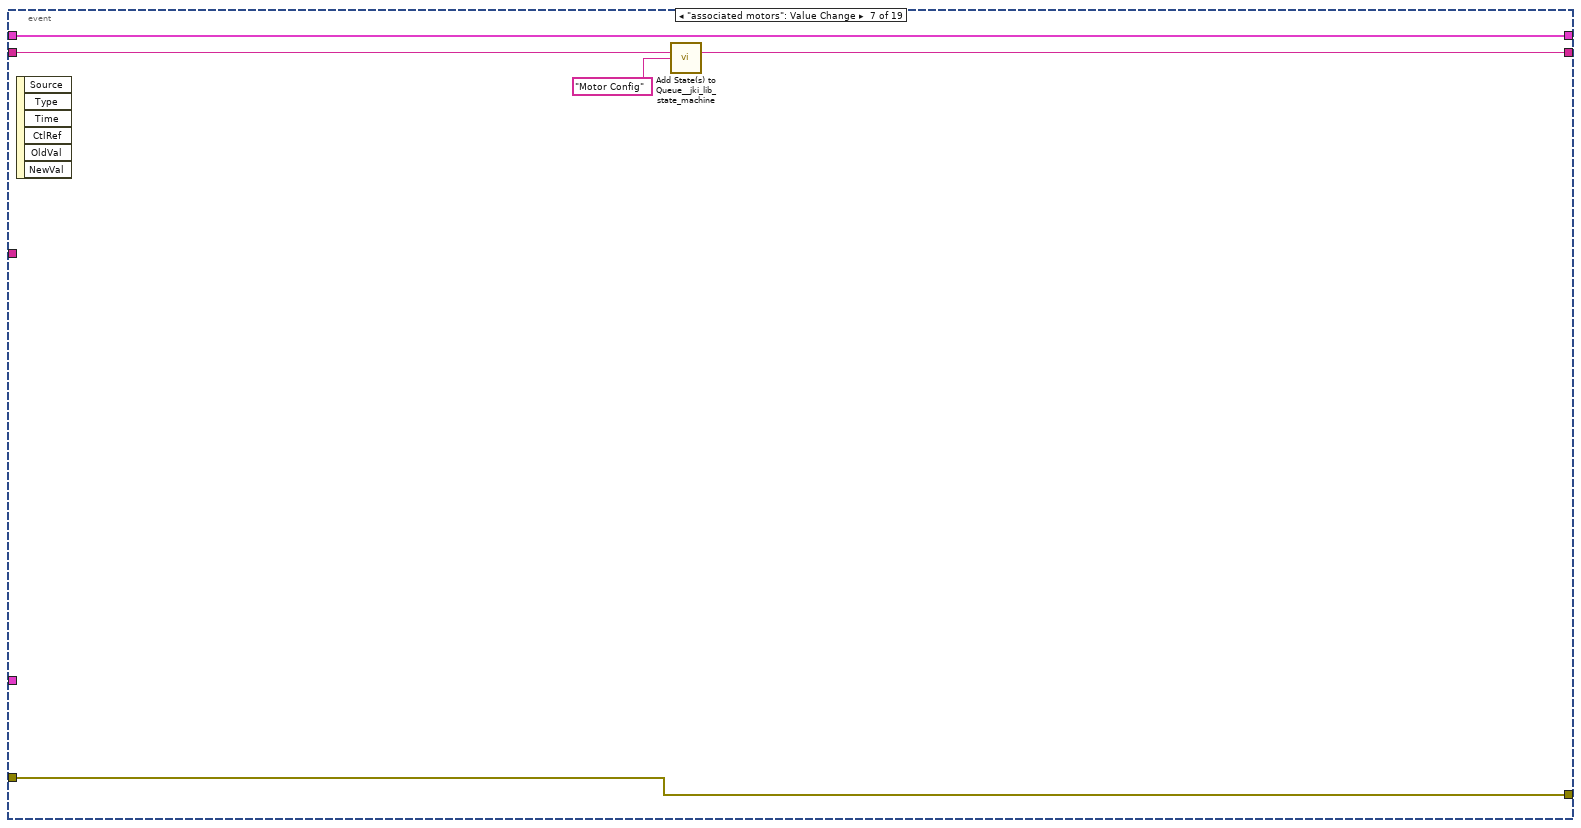
[diagram p15: hidden frame]
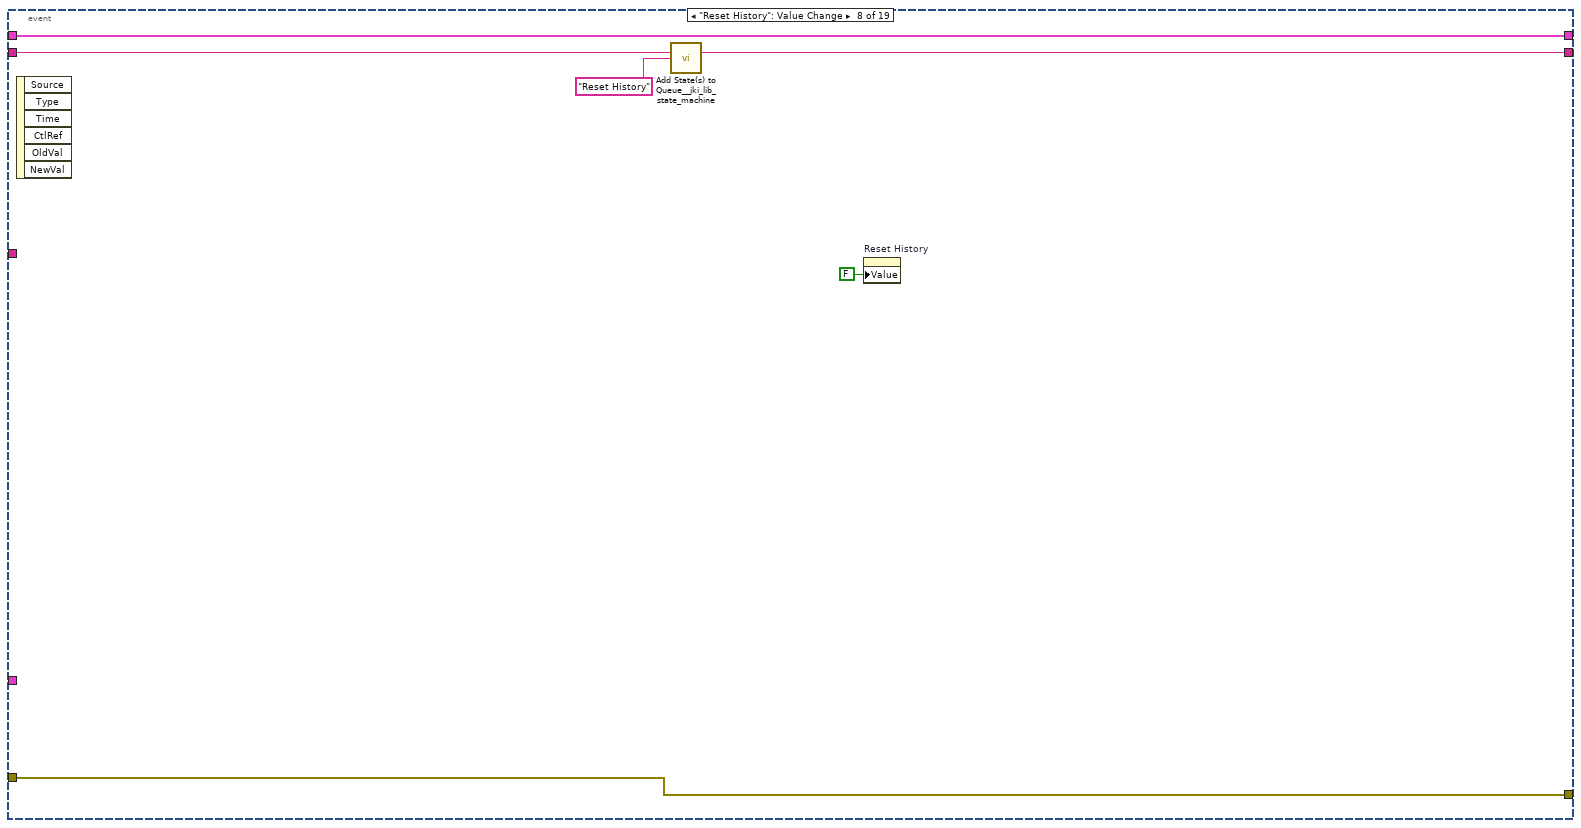
[diagram p16: hidden frame]
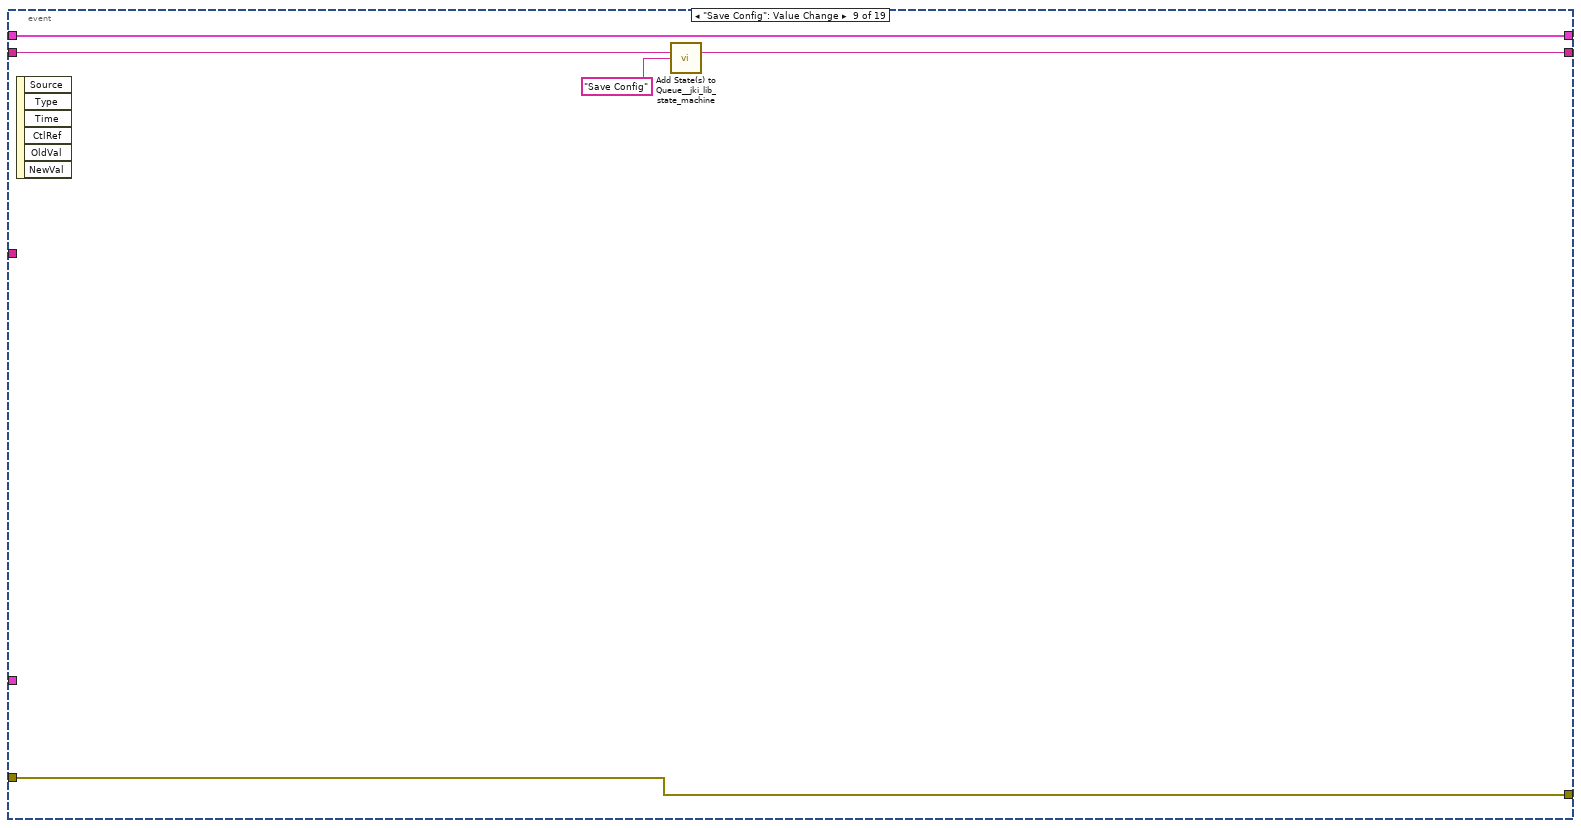
[diagram p17: hidden frame]
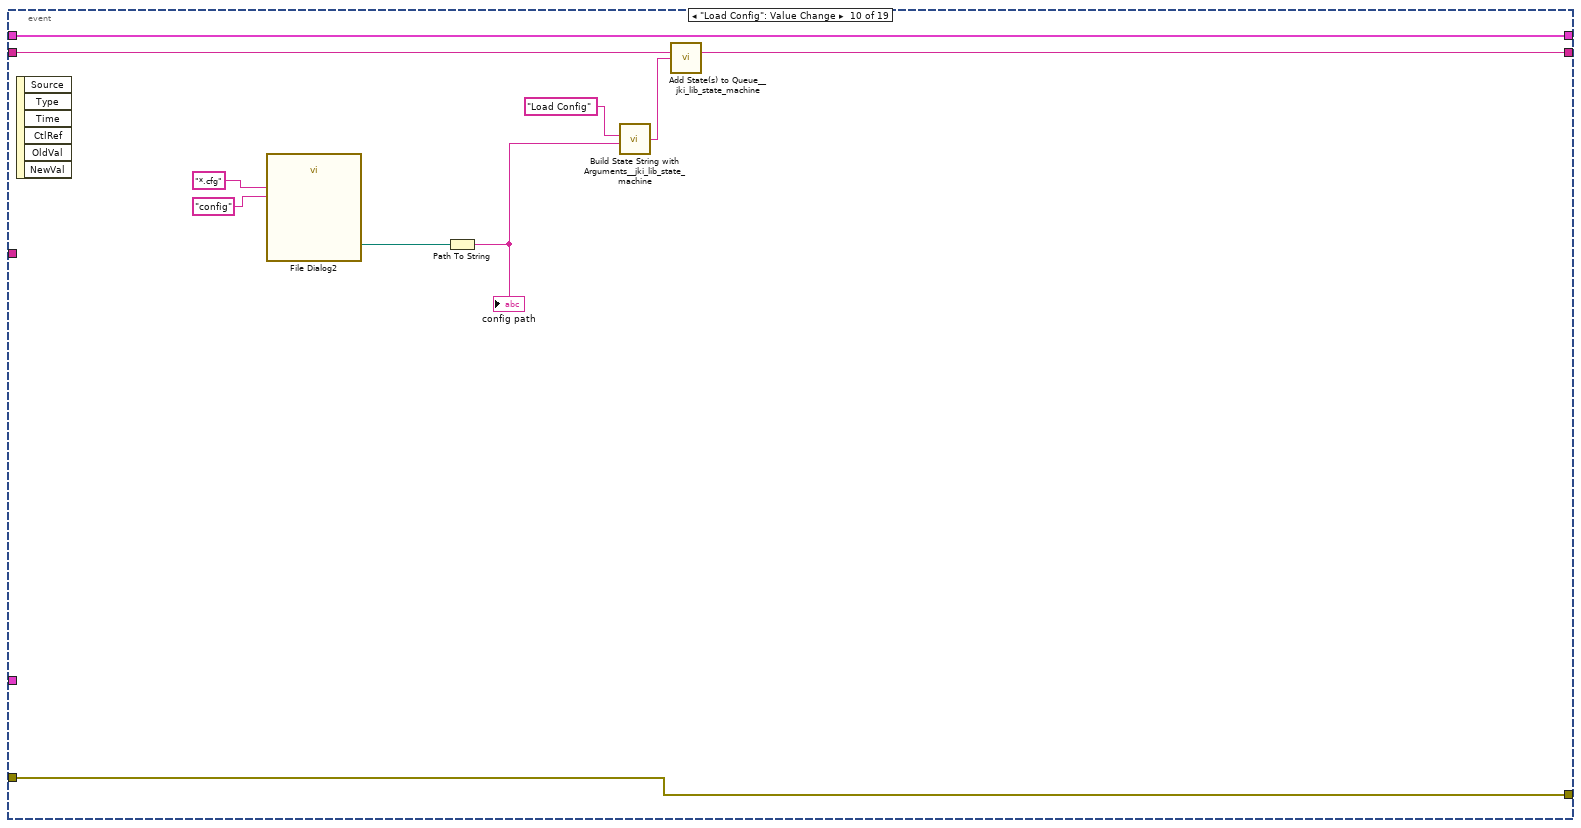
[diagram p18: hidden frame]
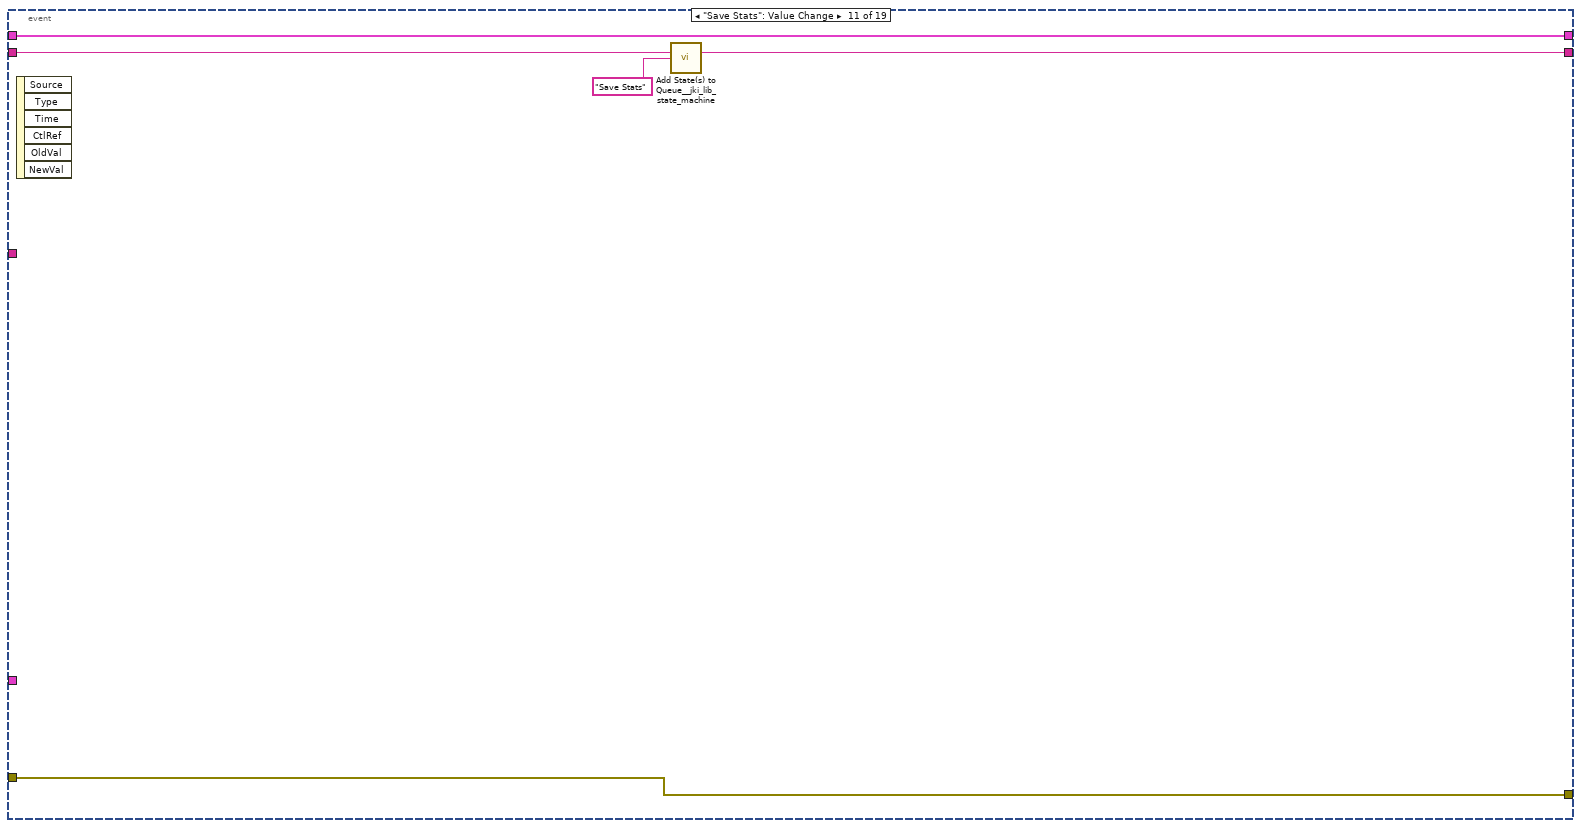
[diagram p19: hidden frame]
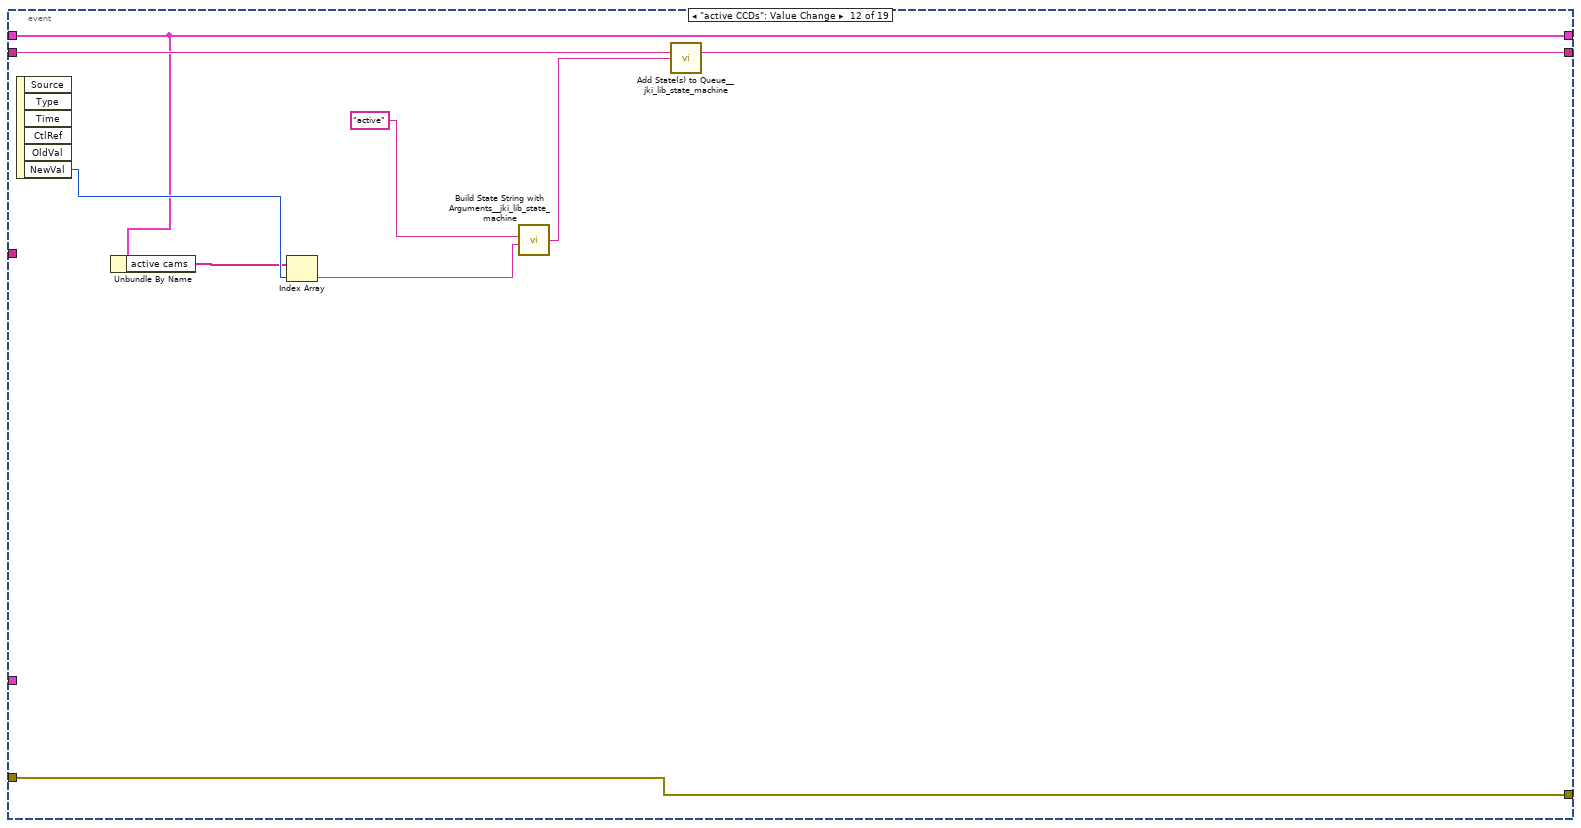
[diagram p20: hidden frame]
diagram:
  n1 = stacked-sequence {
    frame #0 {
      n2 = call <vilib>:"Application Directory.vi"() -> ("Application Directory"=w31:path)
      n3 = Build Path(base path=w31, name or relative path="defaultDevices_TRA.txt") -> (appended path=w29:path)
      "appended path" <- w29
      n4 = call-poly <vilib>:"Read From Spreadsheet File.vi"("file path (dialog if empty)"=w29) -> ("all rows"=w28:string[][])  [unwired: 6 in, 4 out]
      n5 = Index Array(array=w28, index (col) #1=0 ("disabled index (col)"), index (col) #2=1 ("index (col)")) -> (element #1=w25:string[])  [unwired: 2 in, 1 out]
      n6 = Index Array(array=w25, index #1=0 ("index"), index #2=1 ("index"), index #3=2 ("index"), index #4=3 ("index"), index #5=4 ("index"), index #6=5 ("index"), index #7=6 ("index"), index #8=7 ("index"), index #9=8 ("index"), index #10=9 ("index"), index #11=10 ("index"), index #12=11 ("index")) -> (element #1=w12:string, element #2=w11:string, element #3=w10:string, element #4=w9:string, element #5=w8:string, element #6=w7:string, element #7=w6:string, element #8=w5:string, element #9=w4:string, element #10=w3:string, element #11=w2:string, element #12=w1:string)
      n7 = property on="GUIdevice 1" class="Str"("Val(Sgnl)"=w12) -> ()  [unwired: 2 in, 2 out]
      n8 = property on="GUIdevice 2" class="Str"("Val(Sgnl)"=w11) -> ()  [unwired: 2 in, 2 out]
      n9 = property on="GUIdevice 3" class="Str"("Val(Sgnl)"=w10) -> ()  [unwired: 2 in, 2 out]
      n10 = property on="GUIdevice 4" class="Str"("Val(Sgnl)"=w9) -> ()  [unwired: 2 in, 2 out]
      n11 = property on="GUIdevice 5" class="Str"("Val(Sgnl)"=w8) -> ()  [unwired: 2 in, 2 out]
      n12 = property on="GUIdevice 6" class="Str"("Val(Sgnl)"=w7) -> ()  [unwired: 2 in, 2 out]
      n13 = property on="GUIdevice 7" class="Str"("Val(Sgnl)"=w6) -> ()  [unwired: 2 in, 2 out]
      n14 = property on="GUIdevice 8" class="Str"("Val(Sgnl)"=w5) -> ()  [unwired: 2 in, 2 out]
      n15 = property on="GUIdevice 9" class="Str"("Val(Sgnl)"=w4) -> ()  [unwired: 2 in, 2 out]
      n16 = property on="GUIdevice 10" class="Str"("Val(Sgnl)"=w3) -> ()  [unwired: 2 in, 2 out]
      n17 = property on="GUIdevice 11" class="Str"("Val(Sgnl)"=w2) -> ()  [unwired: 2 in, 2 out]
      n18 = property on="GUIdevice 12" class="Str"("Val(Sgnl)"=w1) -> ()  [unwired: 2 in, 2 out]
    }
    frame #1 {
      w34 = string[] ["M20", "SIM", "M22", ""] ("elements")
      w38 = T20 1 items=["Grayscale (U8)", "Grayscale (I16)", "Grayscale (SGL)", "Complex (CSG)", "RGB (U32)", "HSL (U32)", "RGB (U64)", "Grayscale (U16)"] ("Image Type")
      # "NOT FOR YOU MOFO"
      n19 = control-ref of="Position.Axis 1::99"() -> (w112:refnum<vi>)
      n20 = control-ref of="Position.Axis 2::99"() -> (w111:refnum<vi>)
      n21 = control-ref of="Position.Axis 3::99"() -> (w110:refnum<vi>)
      n22 = control-ref of="Position.Axis 4::99"() -> (w109:refnum<vi>)
      n23 = control-ref of="Position.Axis 5::99"() -> (w108:refnum<vi>)
      n24 = control-ref of="Position.Axis 6::99"() -> (w107:refnum<vi>)
      n25 = property on="Motor CCD 1" class="Ring (strict)"("Strings []"=w34) -> ()  [unwired: 2 in, 2 out]
      n26 = property on="Motor CCD 2" class="Ring (strict)"("Strings []"=w34) -> ()  [unwired: 2 in, 2 out]
      n27 = property on="Motor CCD 3" class="Ring (strict)"("Strings []"=w34) -> ()  [unwired: 2 in, 2 out]
      n28 = property on="Motor CCD 4" class="Ring (strict)"("Strings []"=w34) -> ()  [unwired: 2 in, 2 out]
      n29 = property on="Motor CCD 5" class="Ring (strict)"("Strings []"=w34) -> ()  [unwired: 2 in, 2 out]
      n30 = property on="Motor CCD 6" class="Ring (strict)"("Strings []"=w34) -> ()  [unwired: 2 in, 2 out]
      n31 = property on="Motor CCD 7" class="Ring (strict)"("Strings []"=w34) -> ()  [unwired: 2 in, 2 out]
      n32 = property on="Motor CCD 8" class="Ring (strict)"("Strings []"=w34) -> ()  [unwired: 2 in, 2 out]
      n33 = property on="Motor CCD 9" class="Ring (strict)"("Strings []"=w34) -> ()  [unwired: 2 in, 2 out]
      n34 = property on="Motor CCD 10" class="Ring (strict)"("Strings []"=w34) -> ()  [unwired: 2 in, 2 out]
      n35 = property on="Motor CCD 11" class="Ring (strict)"("Strings []"=w34) -> ()  [unwired: 2 in, 2 out]
      n36 = property on="Motor CCD 12" class="Ring (strict)"("Strings []"=w34) -> ()  [unwired: 2 in, 2 out]
      n37 = Build Array(w112, w111, w110, w109, w108, w107) -> (→"motor refs":refnum<vi>[])
      n38 = control-ref of="Target.X::1"() -> (w93:refnum<vi>)
      n39 = control-ref of="Target.Y::1"() -> (w92:refnum<vi>)
      n40 = control-ref of="Target.X::2"() -> (w91:refnum<vi>)
      n41 = control-ref of="Target.Y::2"() -> (w90:refnum<vi>)
      n42 = control-ref of="Target.X::3"() -> (w89:refnum<vi>)
      n43 = control-ref of="Target.Y::3"() -> (w88:refnum<vi>)
      n44 = control-ref of="Target.X::4"() -> (w87:refnum<vi>)
      n45 = control-ref of="Target.Y::4"() -> (w86:refnum<vi>)
      n46 = control-ref of="Target.X::5"() -> (w85:refnum<vi>)
      n47 = control-ref of="Target.Y::5"() -> (w84:refnum<vi>)
      n48 = control-ref of="Target.X::6"() -> (w83:refnum<vi>)
      n49 = control-ref of="Target.Y::6"() -> (w82:refnum<vi>)
      n50 = control-ref of="Target.X::7"() -> (w81:refnum<vi>)
      n51 = control-ref of="Target.Y::7"() -> (w80:refnum<vi>)
      n52 = control-ref of="Target.X::8"() -> (w79:refnum<vi>)
      n53 = control-ref of="Target.Y::8"() -> (w78:refnum<vi>)
      n54 = control-ref of="Target.X::9"() -> (w55:refnum<vi>)
      n55 = control-ref of="Target.Y::9"() -> (w54:refnum<vi>)
      n56 = control-ref of="Target.X::10"() -> (w53:refnum<vi>)
      n57 = control-ref of="Target.Y::10"() -> (w52:refnum<vi>)
      n58 = control-ref of="Target.X::11"() -> (w51:refnum<vi>)
      n59 = control-ref of="Target.Y::11"() -> (w50:refnum<vi>)
      n60 = control-ref of="Target.X::12"() -> (w49:refnum<vi>)
      n61 = control-ref of="Target.Y::12"() -> (w48:refnum<vi>)
      n62 = call "IMAQ Create"("Image Name"="GUIdevice 8", "Image Type"=w38) -> ("New Image"=→"image::8":T9)  [unwired: 3 in, 1 out]
      n63 = call "IMAQ Create"("Image Name"="GUIdevice 9", "Image Type"=w38) -> ("New Image"=→"image::9":T9)  [unwired: 3 in, 1 out]
      n64 = call "IMAQ Create"("Image Name"="GUIdevice 10", "Image Type"=w38) -> ("New Image"=→"image::10":T9)  [unwired: 3 in, 1 out]
      n65 = call "IMAQ Create"("Image Name"="GUIdevice 6", "Image Type"=w38) -> ("New Image"=→"image::6":T9)  [unwired: 3 in, 1 out]
      n66 = call "IMAQ Create"("Image Name"="GUIdevice 7", "Image Type"=w38) -> ("New Image"=→"image::7":T9)  [unwired: 3 in, 1 out]
      n67 = call "IMAQ Create"("Image Name"="GUIdevice 11", "Image Type"=w38) -> ("New Image"=→"image::11":T9)  [unwired: 3 in, 1 out]
      n68 = call "IMAQ Create"("Image Name"="GUIdevice 12", "Image Type"=w38) -> ("New Image"=→"image::12":T9)  [unwired: 3 in, 1 out]
      n69 = call "IMAQ Create"("Image Name"="GUIdevice 2") -> ("New Image"=→"image::2":T9)  [unwired: 4 in, 1 out]
      n70 = call "IMAQ Create"("Image Name"="GUIdevice 4", "Image Type"=w38) -> ("New Image"=→"image::4":T9)  [unwired: 3 in, 1 out]
      n71 = call "IMAQ Create"("Image Name"="GUIdevice 1", "Image Type"=w38) -> ("New Image"=→"image::1":T9)  [unwired: 3 in, 1 out]
      n72 = call "IMAQ Create"("Image Name"="GUIdevice 3", "Image Type"=w38) -> ("New Image"=→"image::3":T9)  [unwired: 3 in, 1 out]
      n73 = call "IMAQ Create"("Image Name"="GUIdevice 5", "Image Type"=w38) -> ("New Image"=→"image::5":T9)  [unwired: 3 in, 1 out]
      n74 = Build Array("GUIdevice 1", "GUIdevice 2", "GUIdevice 3", "GUIdevice 4", "GUIdevice 5", "GUIdevice 6", "GUIdevice 7", "GUIdevice 8", "GUIdevice 9", "GUIdevice 10", "GUIdevice 11", "GUIdevice 12") -> (w67:string[])
      "CCDs" <- w67
      n75 = property on="image::8" class="ImageControl"("Caption.Text"="GUIdevice 8") -> ()  [unwired: 2 in, 2 out]
      n76 = property on="image::10" class="ImageControl"("Caption.Text"="GUIdevice 10") -> ()  [unwired: 2 in, 2 out]
      n77 = property on="image::9" class="ImageControl"("Caption.Text"="GUIdevice 9") -> ()  [unwired: 2 in, 2 out]
      n78 = property on="image::1" class="ImageControl"("Caption.Text"="GUIdevice 1") -> ()  [unwired: 2 in, 2 out]
      n79 = property on="image::2" class="ImageControl"("Caption.Text"="GUIdevice 2") -> ()  [unwired: 2 in, 2 out]
      n80 = property on="image::3" class="ImageControl"("Caption.Text"="GUIdevice 3") -> ()  [unwired: 2 in, 2 out]
      n81 = property on="image::4" class="ImageControl"("Caption.Text"="GUIdevice 4") -> ()  [unwired: 2 in, 2 out]
      n82 = property on="image::5" class="ImageControl"("Caption.Text"="GUIdevice 5") -> ()  [unwired: 2 in, 2 out]
      n83 = property on="image::6" class="ImageControl"("Caption.Text"="GUIdevice 6") -> ()  [unwired: 2 in, 2 out]
      n84 = property on="image::7" class="ImageControl"("Caption.Text"="GUIdevice 7") -> ()  [unwired: 2 in, 2 out]
      n85 = property on="image::11" class="ImageControl"("Caption.Text"="GUIdevice 11") -> ()  [unwired: 2 in, 2 out]
      n86 = property on="image::12" class="ImageControl"("Caption.Text"="GUIdevice 12") -> ()  [unwired: 2 in, 2 out]
      n87 = Array To Cluster(array=w67) -> (cluster=→"Cameras":T21)
      n88 = Bundle("Target.X::1"=w93, "Target.Y::1"=w92) -> (w77:T22)  [unwired: 1 in]
      n89 = Bundle("Target.X::2"=w91, "Target.Y::2"=w90) -> (w76:T23)  [unwired: 1 in]
      n90 = Bundle("Target.X::3"=w89, "Target.Y::3"=w88) -> (w75:T24)  [unwired: 1 in]
      n91 = Bundle("Target.X::4"=w87, "Target.Y::4"=w86) -> (w68:T25)  [unwired: 1 in]
      n92 = Bundle("Target.X::5"=w85, "Target.Y::5"=w84) -> (w74:T26)  [unwired: 1 in]
      n93 = Bundle("Target.X::6"=w83, "Target.Y::6"=w82) -> (w73:T27)  [unwired: 1 in]
      n94 = Bundle("Target.X::7"=w81, "Target.Y::7"=w80) -> (w72:T28)  [unwired: 1 in]
      n95 = Bundle("Target.X::8"=w79, "Target.Y::8"=w78) -> (w71:T29)  [unwired: 1 in]
      n96 = Bundle("Target.X::12"=w49, "Target.Y::12"=w48) -> (w44:T30)  [unwired: 1 in]
      n97 = Bundle("Target.X::9"=w55, "Target.Y::9"=w54) -> (w47:T31)  [unwired: 1 in]
      n98 = Bundle("Target.X::10"=w53, "Target.Y::10"=w52) -> (w46:T32)  [unwired: 1 in]
      n99 = Bundle("Target.X::11"=w51, "Target.Y::11"=w50) -> (w45:T33)  [unwired: 1 in]
      n100 = property on="CCDs" class="Ring (strict)"("Strings []"=w67) -> ()  [unwired: 2 in, 2 out]
      n101 = Build Array(w77, w76, w75, w68, w74, w73, w72, w71, w47, w46, w45, w44) -> (w70:T34)
      n102 = Tick Count (ms)() -> (millisecond timer value=→"millisecond timer value":u32)
      n103 = property on="Feedback Global" class="Bool (strict)"("Value"=FALSE ("Feedback Global")) -> ()  [unwired: 2 in, 2 out]
      n104 = Get Date/Time In Seconds() -> (seconds since 1Jan1904=w57:timestamp)
      n105 = Format Date/Time String(time format string (%c)="%Y%m%d%H%M", seconds (now)=w57) -> (date/time string=w56:string)  [unwired: 1 in]
      n106 = Concatenate Strings(w56, "Beampointing_TRA.tdms" ("string")) -> (w60:string)
      n107 = String To Path(string=w60) -> (path=w59:path)
      n108 = Build Path(base path=path "c:/BP_DATA", name or relative path=w59) -> (appended path=w62:path)
      n109 = call <vilib>:"Add State(s) to Queue__jki_lib_state_machine.vi"("State(s) in (\"\")"="Macro: Initialize") -> ("States Out"=w114:string)  [unwired: 14 in]
      n110 = Create User Event(user event datatype=T13 {"EventEnum"=enum."new data", "Device name"="Device name"} ("New Event")) -> (user event=w122:refnum<user-event>, error out=w124:errorcluster)  [unwired: 1 in]
      "tcp data event" <- w122
      n111 = while "JKI - String-Based Queued State Machine (Basic) v1.0" {
        shift-right: [w141] -> w66
        shift-left: _ -> [w134]
        shift-right: [w144] -> w94
        shift-left: _ -> [w140]
        shift-right: [w143] -> _
        shift-left: w114 -> [w145]
        tunnel: w70 -> [w138]
        tunnel: w67 -> [w136]
        tunnel: [w136] -> w95
        tunnel: w70 -> [w137]
        tunnel: w62 -> [w132]
        stop <- w142 stop-if-true
        n112 = Unbundle By Name(w134) -> ("active cams"=w133:string[])
        n113 = call <vilib>:"Parse State Queue__jki_lib_state_machine.vi"("State Queue"=w145, "Error In (no error)"=w140) -> ("Remaining States"=w147:string, "Current State"=w148:string, "Arguments"=w146:string)  [unwired: 11 in]
        "Current State" <- w148
        n114 = case shown="\"newtdms\"" w148 {
          selector: w148 -> [_ _ w461 _ _ _ _ _ _ _ _ _ _ _ _ _ _ _ _ _ _ _ _ _ _ _ _ _ _ _ _ _ _ _ _ _ _ _ _ _ _ _]
          tunnel: w147 -> [w173 w460 w465 w483 w489 w494 w498 w539 w545 w549 w553 w559 w570 w594 w603 w613 w617 w641 w741 w793 w823 w832 w854 w875 w879 w895 w1039 w1170 w1250 w1314 w1385 w1461 w1485 w1500 w1583 w1635 w1645 w1680 w1721 w1741 w1752 w1775]
          tunnel: w146 -> [_ _ _ _ _ _ _ _ _ _ _ w554 w565 _ _ _ _ w634 w693 _ w808 _ _ _ _ w896 _ w1145 w1236 w1300 w1360 w1455 _ _ _ _ _ _ _ _ w1756 _]
          tunnel: w134 -> [w171 w457 w463 w473 w486 w492 w495 _ w540 w546 w551 w557 w564 w591 w600 w605 w614 w631 w731 w791 w804 w828 w846 w868 w876 w884 w1020 w1163 w1246 w1310 w1378 w1457 w1482 w1497 w1563 w1632 w1642 w1653 w1707 w1738 w1755 w1766]
          tunnel: [w170 w458 w467 w481 errorcluster {"status"=FALSE, "code"=0, "source"=""} ("error out") w491 w496 w501 w542 w547 w550 w555 w567 w592 w601 w611 w615 w635 w696 w782 w812 w830 w852 w873 w877 w929 w1052 w1168 w1248 w1312 w1383 w1450 w1483 w1498 w1576 w1633 w1643 w1678 w1699 w1739 w1750 w1773] -> w144
          tunnel: w140 -> [w169 w458 w466 w481 w485 w491 w496 w502 w543 w547 w550 w556 w568 w592 w601 w611 w615 w636 w694 w783 w811 w830 w852 w873 w877 w929 w1052 w1168 w1248 w1312 w1383 w1451 w1483 w1498 w1577 w1633 w1643 w1678 w1701 w1739 w1750 w1773]
          tunnel: [w172 w459 w464 w482 w488 w493 w497 w538 w544 w548 w552 w558 w569 w593 w602 w612 w616 w625 w740 w792 w822 w831 w853 w874 w878 w900 w1053 w1169 w1249 w1313 w1384 w1460 w1484 w1499 w1582 w1634 w1644 w1679 w1720 w1740 w1751 w1774] -> w143
          tunnel: [_ _ _ _ _ TRUE _ _ _ _ _ _ _ _ _ _ _ _ _ _ _ _ _ _ _ _ _ _ _ _ _ _ _ _ _ _ _ _ _ _ _ _] -> w142
          tunnel: [w166 w457 w463 w472 w486 w492 w495 w508 w540 w546 w551 w557 w564 w591 w600 w605 w614 w638 w730 w791 w817 w827 w845 w867 w876 w922 w1019 w1163 w1246 w1310 w1378 w1459 w1482 w1497 w1563 w1631 w1642 w1653 w1706 w1738 w1754 w1765] -> w141
          tunnel: "update speed [ms]" -> [w168 _ _ _ _ _ _ _ _ _ _ _ _ _ _ _ _ _ _ _ _ _ _ _ _ _ _ _ _ _ _ _ _ _ _ _ _ _ _ _ _ _]
          tunnel: w138 -> [w165 _ _ _ _ _ _ _ _ _ _ _ _ _ _ _ _ _ _ _ _ _ _ _ _ w920 _ _ _ _ _ _ _ _ _ _ _ _ _ w1723 _ _]
          tunnel: w136 -> [w167 _ _ _ _ _ _ _ _ _ _ _ _ _ _ _ _ w640 w729 _ w818 _ _ _ _ w888 _ w1167 _ _ w1382 w1456 _ w1486 _ _ _ w1652 _ _ _ _]
          tunnel: w132 -> [_ _ _ _ _ _ _ w500 _ _ _ _ _ _ _ _ _ w637 _ _ _ _ _ _ _ _ _ _ _ _ _ _ _ _ _ _ _ _ _ _ _ _]
          frame "", "Idle" {
            # "executes when the state queue is empty"
            n115 = event shown="[0] Timeout" {
              selector: _ -> [_ _ _ _ _ _ _ _ _ _ _ _ _ _ _ _ _ _ _]
              dyn-events: _ -> [_ _ _ _ _ _ _ _ _ _ _ _ _ _ _ _ _ _ _]
              timeout: w168 -> [_ _ _ _ _ _ _ _ _ _ _ _ _ _ _ _ _ _ _]
              tunnel: w173 -> [w211 w318 w333 w352 w357 w362 w367 w373 w378 w388 w393 w402 w414 w426 w431 w436 w442 w446 w456]
              tunnel: [w188 w317 w332 w351 w356 w361 w366 w372 w377 w387 w392 w401 w413 w425 w430 w435 w441 w444 w455] -> w172
              tunnel: w171 -> [w181 w315 w329 w348 w354 w359 w364 w370 w375 w385 w390 w395 w412 w424 w429 w434 w440 w447 w453]
              tunnel: [w207 w316 w331 w350 w355 w360 w365 w371 w376 w386 w391 w400 w407 w419 w428 w433 w439 w443 w454] -> w170
              tunnel: w169 -> [w208 w316 w331 w350 w355 w360 w365 w371 w376 w386 w391 w400 w408 w420 w428 w433 w439 w443 w454]
              tunnel: [w186 w315 w329 w347 w354 w359 w364 w370 w375 w385 w390 w395 w412 w424 w429 w434 w440 w447 w453] -> w166
              tunnel: w167 -> [w206 _ w325 _ _ _ _ _ _ _ _ _ _ _ _ _ _ _ _]
              tunnel: w165 -> [_ _ w327 _ _ _ _ _ _ _ _ _ _ _ _ _ _ _ _]
              event Timeout {
                n116 = event-data() -> ()  [unwired: 1 in, 1 out]
                n117 = Unbundle By Name(w181) -> ("Centroid X"=w179:dbl[][], "Centroid Y"=w178:dbl[][], "Size"=w177:dbl[][], "detection para"=w205:T3[], "active cams"=w200:string[], "thresholds"=w196:cluster{"Lower value":sgl, "Upper value":sgl}[])
                n118 = Unbundle By Name(w181) -> ("active ccd"=w180:i32)
                n119 = Array Size(array=w179) -> (size(s)=→"size(s)":i32[])
                n120 = Array Size(array=w178) -> (size(s)=→"size(s) 2":i32[])
                n121 = Array Size(array=w177) -> (size(s)=→"size(s) 3":i32[])
                n122 = for {
                  N -> [w243]
                  tunnel: w200 -> [w256] mode=indexing
                  tunnel: [w270] -> w217 mode=indexing
                  tunnel: [w267] -> w218 mode=indexing
                  tunnel: [w273] -> w216 mode=indexing
                  tunnel: w179 -> [w253]
                  tunnel: w178 -> [w251]
                  tunnel: w177 -> [w248]
                  tunnel: [w266] -> w210 mode=indexing
                  tunnel: [w265] -> w209
                  tunnel: w208 -> [w264]
                  tunnel: w206 -> [w263]
                  tunnel: w205 -> [w261]
                  tunnel: [w259] -> w184 mode=indexing
                  tunnel: [w258] -> w182 mode=indexing
                  tunnel: [w255] -> w201 mode=indexing
                  tunnel: [w246] -> w198 mode=indexing
                  tunnel: "autodetect" -> [w245]
                  tunnel: w196 -> [w244] mode=indexing
                  i -> [w249]
                  w269 = dbl[] [] ("Array 4")
                  n123 = Index Array(array=w248, index (row)=w249) -> (element=w247:dbl[])  [unwired: 1 in]
                  n124 = Index Array(array=w251, index (row)=w249) -> (element=w250:dbl[])  [unwired: 1 in]
                  n125 = call-poly <userlib>:"Filter 1D Array__ogtk.vi"("items to filter"=w256, "array"=w263) -> ("filtered item indices"=w262:i32[])  [unwired: 4 in, 1 out]
                  n126 = Index Array(array=w253, index (row)=w249) -> (element=w252:dbl[])  [unwired: 1 in]
                  n127 = Index Array(array=w262) -> (element=w254:i32)  [unwired: 1 in]
                  n128 = Index Array(array=w261, index=w254) -> (element=w257:T3)
                  n129 = call "CENTRIOD DETECTION.vi"("Refnum in"=w256, "auto threshold"=w245, "Threshold Range In"=w244, "beam detection para"=w257, "error in (no error)"=w264) -> ("Bounding Rect"=w255:T35, "Particle Reports (Pixels)"=w258:T1, "Threshold Range Out"=w246:cluster{"Lower value":sgl, "Upper value":sgl}, "Centriod"=w278:cluster{"X":dbl, "Y":dbl}, "error out"=w265:errorcluster)  [unwired: 7 in, 3 out]
                  n130 = Unbundle By Name(w278) -> ("X"=w275:dbl, "Y"=w274:dbl)
                  n131 = Empty Array?(array=w258) -> (empty?=w260:bool)
                  n132 = Not Equal To 0?(x=w274) -> (x != 0?=w276:bool)
                  n133 = Not Equal To 0?(x=w275) -> (x != 0?=w277:bool)
                  n134 = Not(x=w260) -> (.not. x?=w259:bool)
                  n135 = And(x=w277, y=w276) -> (x .and. y?=w272:bool)
                  n136 = case shown="True" w272 {
                    tunnel: w275 -> [_ w311]
                    tunnel: w274 -> [_ w310]
                    tunnel: w252 -> [w297 w313]
                    tunnel: w250 -> [w296 w312]
                    tunnel: [w297 w309] -> w271
                    tunnel: [w296 w308] -> w268
                    tunnel: w255 -> [_ w307]
                    tunnel: w247 -> [w295 w300]
                    tunnel: [w295 w298] -> w266
                    frame False {
                    }
                    frame True {
                      n137 = Unbundle By Name(w307) -> ("Right"=w306:dbl, "Left"=w305:dbl, "Bottom"=w304:dbl, "Top"=w303:dbl)
                      n138 = Subtract(x=w306, y=w305) -> (x-y=w301:dbl)
                      n139 = Subtract(x=w304, y=w303) -> (x-y=w302:dbl)
                      n140 = Build Array (concatenate)(w313, w311) -> (w309:dbl[])
                      n141 = Multiply(x=w301, y=w302) -> (x*y=w299:dbl)
                      n142 = Build Array (concatenate)(w312, w310) -> (w308:dbl[])
                      n143 = Build Array (concatenate)(w300, w299) -> (w298:dbl[])
                    }
                  }
                  n144 = for {
                    tunnel: w271 -> [w288] mode=indexing
                    shift-right: [w287] -> w270
                    shift-left: w269 -> [w289]
                    n145 = Not Equal To 0?(x=w288) -> (x != 0?=w290:bool)
                    n146 = case shown="True" w290 {
                      tunnel: w289 -> [w291 w294]
                      tunnel: w288 -> [_ w293]
                      tunnel: [w291 w292] -> w287
                      frame False {
                      }
                      frame True {
                        n147 = Build Array (concatenate)(w294, w293) -> (w292:dbl[])
                      }
                    }
                  }
                  n148 = for {
                    tunnel: w268 -> [w280] mode=indexing
                    shift-right: [w279] -> w267
                    shift-left: w269 -> [w281]
                    n149 = Not Equal To 0?(x=w280) -> (x != 0?=w282:bool)
                    n150 = case shown="True" w282 {
                      tunnel: w281 -> [w283 w286]
                      tunnel: w280 -> [_ w285]
                      tunnel: [w283 w284] -> w279
                      frame False {
                      }
                      frame True {
                        n151 = Build Array (concatenate)(w286, w285) -> (w284:dbl[])
                      }
                    }
                  }
                  n152 = Array Size(array=w267) -> (size(s)=w273:i32)
                  "Numeric 2" <- w243
                }
                "detected" <- w184
                "Box" <- w201
                n153 = Bundle(0, 1, "Centroid X"=w179) -> (→"Status":cluster{i32, i32, "Centroid X":dbl[][]})  [unwired: 1 in]
                n154 = Index Array(array=w182, index (row)=w180) -> (element=→"particles":T1)  [unwired: 1 in]
                n155 = call <vilib>:"Clear Errors.vi"("error in (no error)"=w209) -> ("error out"=w207:errorcluster)  [unwired: 6 in]
                n156 = local read "img to avg"() -> (w190:i32)
                n157 = local read "Numeric"() -> (w193:dbl)
                n158 = Bundle By Name(cluster=w181, "thresholds"=w198) -> (w197:T36)
                n159 = Increment(x=w190) -> (x+1=w189:i32)
                n160 = Greater Or Equal?(x=w193, y=w189) -> (x >= y?=w185:bool)
                n161 = Increment(x=w193) -> (x+1=w192:dbl)
                n162 = Select(t=0.0, s=w185, f=w192) -> (s? t:f=w191:dbl)
                n163 = local write "Numeric"(w191) -> ()
                n164 = for {
                  tunnel: w216 -> [w235] mode=indexing
                  tunnel: w200 -> [w242] mode=indexing
                  shift-right: [w237] -> w212
                  shift-left: "" ("GUIdevice 7") -> [w240]
                  tunnel: [w230] -> w214 mode=indexing
                  tunnel: "Detection Rate" -> [w234]
                  tunnel: w191 -> [w232]
                  n165 = local read "img to avg"() -> (w236:i32)
                  n166 = Greater Or Equal?(x=w235, y=w236) -> (x >= y?=w231:bool)
                  n167 = Multiply(x=w234, y=w232) -> (x*y=w233:dbl)
                  n168 = Greater Or Equal?(x=w235, y=w233) -> (x >= y?=w229:bool)
                  n169 = And(x=w231, y=w229) -> (x .and. y?=w230:bool)
                  n170 = Select(t=w242, s=w230, f="") -> (s? t:f=w238:string)
                  n171 = Concatenate Strings(w240, "\t", w238) -> (w237:string)
                }
                n172 = Bundle By Name(cluster=w197, "Centroid X"=w217, "Centroid Y"=w218, "Size"=w210) -> (w187:T36)
                n173 = case shown="True" w185 {
                  tunnel: w187 -> [w219 w222]
                  tunnel: [w219 w221] -> w186
                  frame False {
                  }
                  frame True {
                    n174 = local read "Centroid X"() -> (w220:dbl[][])
                    n175 = Bundle By Name(cluster=w222, "Centroid X"=w220, "Centroid Y"=w220, "Size"=w220) -> (w221:T36)
                  }
                }
                n176 = Or Array Elements(Boolean array=w214) -> (logical OR=w213:bool)
                n177 = case shown="True" w213 {
                  tunnel: w212 -> [_ w227]
                  tunnel: w211 -> [w223 w225]
                  tunnel: [w223 w224] -> w188
                  frame False {
                  }
                  frame True {
                    n178 = call <vilib>:"Build State String with Arguments__jki_lib_state_machine.vi"("Arguments (\"\")"=w227, "State"="detected") -> ("State with Arguments"=w226:string)  [unwired: 4 in]
                    n179 = call <vilib>:"Add State(s) to Queue__jki_lib_state_machine.vi"("State(s) in (\"\")"=w225, "State(s) at Back (\"\")"=w226) -> ("States Out"=w224:string)  [unwired: 13 in]
                  }
                }
              }
              event "stop": Value Change {
                # "Exit Button Value Change (pressed) Event\n(this executes Macro: Exit to terminate the VI)"
                n180 = event-data() -> ()  [unwired: 1 in, 6 out]
                n181 = call <vilib>:"Add State(s) to Queue__jki_lib_state_machine.vi"("State(s) in Front (\"\")"="Macro: Exit", "State(s) in (\"\")"=w318) -> ("States Out"=w317:string)  [unwired: 13 in]
              }
              event Value Change {
                n182 = event-data() -> ()  [unwired: 1 in, 6 out]
                n183 = property on="Set Centriod Target" class="Bool (strict)"("Value"=FALSE) -> ()  [unwired: 2 in, 2 out]
                n184 = Unbundle By Name(w329) -> ("active ccd"=w321:i32, "Centroid X"=w320:dbl[][], "Centroid Y"=w319:dbl[][])
                n185 = Index Array(array=w325, index=w321) -> (element=w324:string)
                n186 = Concatenate Strings("Do want to update the target of " ("message"), w324, "?" ("string")) -> (w322:string)
                n187 = Two Button Dialog(message=w322) -> (T button?=w328:bool)  [unwired: 2 in]
                n188 = case shown="True" w328 {
                  tunnel: w327 -> [_ w340]
                  tunnel: w321 -> [_ w339]
                  tunnel: w320 -> [_ w346]
                  tunnel: w319 -> [_ w341]
                  frame False {
                  }
                  frame True {
                    n189 = Index Array(array=w346, index (row)=w339) -> (element=w345:dbl[])  [unwired: 1 in]
                    n190 = Index Array(array=w341, index (row)=w339) -> (element=w342:dbl[])  [unwired: 1 in]
                    n191 = Index Array(array=w340, index=w339) -> (element=w338:T30)
                    n192 = Unbundle By Name(w338) -> ("Target.X::12"=w337:refnum<vi>, "Target.Y::12"=w335:refnum<vi>)
                    n193 = Reverse 1D Array(array=w345) -> (reversed array=w344:dbl[])
                    n194 = Reverse 1D Array(array=w342) -> (reversed array=w343:dbl[])
                    n195 = Index Array(array=w344) -> (element=w336:dbl)  [unwired: 1 in]
                    n196 = Index Array(array=w343) -> (element=w334:dbl)  [unwired: 1 in]
                    n197 = property class="DigNum (strict)"(reference=w337, "Val(Sgnl)"=w336) -> ()  [unwired: 1 in, 2 out]
                    n198 = property class="DigNum (strict)"(reference=w335, "Val(Sgnl)"=w334) -> ()  [unwired: 1 in, 2 out]
                  }
                }
                n199 = call <vilib>:"Add State(s) to Queue__jki_lib_state_machine.vi"("State(s) in (\"\")"=w333) -> ("States Out"=w332:string)  [unwired: 14 in]
              }
              event "Feedback Global": Value Change {
                # "Exit Button Value Change (pressed) Event\n(this executes Macro: Exit to terminate the VI)"
                n200 = event-data() -> ("NewVal"=w349:bool)  [unwired: 1 in, 5 out]
                n201 = call <vilib>:"Add State(s) to Queue__jki_lib_state_machine.vi"("State(s) in (\"\")"=w352) -> ("States Out"=w351:string)  [unwired: 14 in]
                n202 = Bundle By Name(cluster=w348, "Feedback global"=w349) -> (w347:T36)
              }
              event Value Change {
                n203 = event-data() -> ()  [unwired: 1 in, 6 out]
                n204 = call <vilib>:"Add State(s) to Queue__jki_lib_state_machine.vi"("State(s) in Front (\"\")"="Move Config", "State(s) in (\"\")"=w357) -> ("States Out"=w356:string)  [unwired: 13 in]
              }
              event Value Change {
                n205 = event-data() -> ()  [unwired: 1 in, 6 out]
                n206 = call <vilib>:"Add State(s) to Queue__jki_lib_state_machine.vi"("State(s) in Front (\"\")"="Detection Config", "State(s) in (\"\")"=w362) -> ("States Out"=w361:string)  [unwired: 13 in]
              }
              event "associated motors": Value Change {
                n207 = event-data() -> ()  [unwired: 1 in, 6 out]
                n208 = call <vilib>:"Add State(s) to Queue__jki_lib_state_machine.vi"("State(s) in (\"\")"=w367, "State(s) at Back (\"\")"="Motor Config" ("State(s) at Back (\"\")")) -> ("States Out"=w366:string)  [unwired: 13 in]
              }
              event "Reset History": Value Change {
                n209 = event-data() -> ()  [unwired: 1 in, 6 out]
                n210 = call <vilib>:"Add State(s) to Queue__jki_lib_state_machine.vi"("State(s) in (\"\")"=w373, "State(s) at Back (\"\")"="Reset History" ("State(s) at Back (\"\")")) -> ("States Out"=w372:string)  [unwired: 13 in]
                n211 = property on="Reset History" class="Bool (strict)"("Value"=FALSE ("Reset History")) -> ()  [unwired: 2 in, 2 out]
              }
              event "Save Config": Value Change {
                n212 = event-data() -> ()  [unwired: 1 in, 6 out]
                n213 = call <vilib>:"Add State(s) to Queue__jki_lib_state_machine.vi"("State(s) in (\"\")"=w378, "State(s) at Back (\"\")"="Save Config" ("State(s) at Back (\"\")")) -> ("States Out"=w377:string)  [unwired: 13 in]
              }
              event "Load Config": Value Change {
                n214 = event-data() -> ()  [unwired: 1 in, 6 out]
                n215 = call "File Dialog2"("pattern (all files)"="*.cfg", "pattern label"="config") -> ("selected path"=w382:path)  [unwired: 10 in, 3 out]
                n216 = Path To String(path=w382) -> (string=w380:string)
                "config path" <- w380
                n217 = call <vilib>:"Build State String with Arguments__jki_lib_state_machine.vi"("Arguments (\"\")"=w380, "State"="Load Config" ("State(s) at Back (\"\")")) -> ("State with Arguments"=w379:string)  [unwired: 4 in]
                n218 = call <vilib>:"Add State(s) to Queue__jki_lib_state_machine.vi"("State(s) in (\"\")"=w388, "State(s) at Back (\"\")"=w379) -> ("States Out"=w387:string)  [unwired: 13 in]
              }
              event "Save Stats": Value Change {
                n219 = event-data() -> ()  [unwired: 1 in, 6 out]
                n220 = call <vilib>:"Add State(s) to Queue__jki_lib_state_machine.vi"("State(s) in (\"\")"=w393, "State(s) at Back (\"\")"="Save Stats" ("State(s) at Back (\"\")")) -> ("States Out"=w392:string)  [unwired: 13 in]
              }
              event "active CCDs": Value Change {
                n221 = event-data() -> ("NewVal"=w399:i32)  [unwired: 1 in, 5 out]
                n222 = Unbundle By Name(w395) -> ("active cams"=w394:string[])
                n223 = Index Array(array=w394, index=w399) -> (element=w397:string)
                n224 = call <vilib>:"Build State String with Arguments__jki_lib_state_machine.vi"("Arguments (\"\")"=w397, "State"="active" ("State(s) at Back (\"\")")) -> ("State with Arguments"=w396:string)  [unwired: 4 in]
                n225 = call <vilib>:"Add State(s) to Queue__jki_lib_state_machine.vi"("State(s) in (\"\")"=w402, "State(s) at Back (\"\")"=w396) -> ("States Out"=w401:string)  [unwired: 13 in]
              }
              event "Left", "Right": Value Change {
                n226 = event-data() -> ("CtlRef"=w411:refnum<vi>)  [unwired: 1 in, 5 out]
                n227 = property class="Bool (strict)"(reference=w411, error in=w408) -> (reference out=w410:refnum<vi>, error out=w409:errorcluster, "Label.Text"=w405:string)
                n228 = property class="Bool (strict)"(reference=w410, error in=w409, "Value"=FALSE) -> (error out=w407:errorcluster)  [unwired: 1 out]
                n229 = call <vilib>:"Build State String with Arguments__jki_lib_state_machine.vi"("Arguments (\"\")"=w405, "State"="ManMove X") -> ("State with Arguments"=w404:string)  [unwired: 4 in]
                n230 = call <vilib>:"Add State(s) to Queue__jki_lib_state_machine.vi"("State(s) in (\"\")"=w414, "State(s) at Back (\"\")"=w404) -> ("States Out"=w413:string)  [unwired: 13 in]
              }
              event "Up", "Down": Value Change {
                n231 = event-data() -> ("CtlRef"=w423:refnum<vi>)  [unwired: 1 in, 5 out]
                n232 = property class="Bool (strict)"(reference=w423, error in=w420) -> (reference out=w422:refnum<vi>, error out=w421:errorcluster, "Label.Text"=w417:string)
                n233 = property class="Bool (strict)"(reference=w422, error in=w421, "Value"=FALSE) -> (error out=w419:errorcluster)  [unwired: 1 out]
                n234 = call <vilib>:"Build State String with Arguments__jki_lib_state_machine.vi"("Arguments (\"\")"=w417, "State"="ManMove Y") -> ("State with Arguments"=w416:string)  [unwired: 4 in]
                n235 = call <vilib>:"Add State(s) to Queue__jki_lib_state_machine.vi"("State(s) in (\"\")"=w426, "State(s) at Back (\"\")"=w416) -> ("States Out"=w425:string)  [unwired: 13 in]
              }
              event "Center": Value Change {
                n236 = event-data() -> ()  [unwired: 1 in, 6 out]
                n237 = call <vilib>:"Add State(s) to Queue__jki_lib_state_machine.vi"("State(s) in (\"\")"=w431, "State(s) at Back (\"\")"="Center" ("State(s) at Back (\"\")")) -> ("States Out"=w430:string)  [unwired: 13 in]
              }
              event "new tdms": Value Change {
                n238 = event-data() -> ()  [unwired: 1 in, 6 out]
                n239 = call <vilib>:"Add State(s) to Queue__jki_lib_state_machine.vi"("State(s) in (\"\")"=w436, "State(s) at Back (\"\")"="newtdms" ("State(s) at Back (\"\")")) -> ("States Out"=w435:string)  [unwired: 13 in]
              }
              event "device ini": Value Change {
                n240 = event-data() -> ()  [unwired: 1 in, 6 out]
                n241 = property on="device ini" class="Bool (strict)"("Value"=FALSE ("test")) -> ()  [unwired: 2 in, 2 out]
                n242 = call <vilib>:"Add State(s) to Queue__jki_lib_state_machine.vi"("State(s) in (\"\")"=w442, "State(s) at Back (\"\")"="Device Ini" ("State(s) at Back (\"\")")) -> ("States Out"=w441:string)  [unwired: 13 in]
              }
              event "img to avg": Value Change {
                n243 = event-data() -> ("NewVal"=w448:i32)  [unwired: 1 in, 5 out]
                n244 = Number To Decimal String(number=w448) -> (decimal integer string=w450:string)  [unwired: 1 in]
                n245 = call <vilib>:"Build State String with Arguments__jki_lib_state_machine.vi"("Arguments (\"\")"=w450, "State"="ImgToAvg" ("State(s) at Back (\"\")")) -> ("State with Arguments"=w445:string)  [unwired: 4 in]
                n246 = call <vilib>:"Add State(s) to Queue__jki_lib_state_machine.vi"("State(s) in (\"\")"=w446, "State(s) at Back (\"\")"=w445) -> ("States Out"=w444:string)  [unwired: 13 in]
              }
              event Panel Close? {
                # "Discard the event because we'll close the front panel ourselves in Macro: Exit"
                # "Close Panel button (pressed) Event\n(this executes Macro: Exit to terminate the VI)"
                n247 = event-data() -> ()  [unwired: 1 in, 1 out]
                n248 = call <vilib>:"Add State(s) to Queue__jki_lib_state_machine.vi"("State(s) in Front (\"\")"="Macro: Exit", "State(s) in (\"\")"=w456) -> ("States Out"=w455:string)  [unwired: 13 in]
                n249 = event-data("Discard?"=TRUE) -> ()  [unwired: 1 in, 1 out]
              }
            }
          }
          frame "---------- Core ----------" {
            # "Do not put any code in this frame.\n(it is a separator no-op)"
            n250 = call <vilib>:"Add State(s) to Queue__jki_lib_state_machine.vi"("State(s) in (\"\")"=w460) -> ("States Out"=w459:string)  [unwired: 14 in]
          }
          frame Default {
            w470 = 42 items=["No error", "Argument error", "Memory is full", "Out of zone", "End of file", "File already open", "Generic file I/O error", "File not found", "File permission error", "Disk is full", "Duplicate path", "Too many files open", "System feature not enabled", "Resource file not found", "Cannot add resource", "Resource not found", "Image not found", "Image memory error", "Pen does not exist", "Config type invalid", "Config token not found", "Config parse error", "Config memory error", "Bad external code format", "Bad external code offset", "External code not present", "Null window", "Destroy window error", "Null menu", "Print aborted", "Bad print record", "Print driver error", "Windows error during printing", "Memory error during printing", "Print dialog error", "Generic print error", "Invalid device refnum", "Device not found", "Device parameter error", "Device unit error", "Cannot open device", "Device call aborted", "Generic error", "Cancelled by user", "Object ID too low", "Object ID too high", "Object not in heap", "Unknown heap", "Unknown object (invalid DefProc)", "Unknown object (DefProc not in table)", "Message out of range", "Invalid (null) method", "Unknown message", "Manager call not supported", "Bad address", "Network operation in progress", "Network operation timed out", "Connection is busy", "Network attribute not supported", "Network error", "Address in use", "System out of memory", "Connection aborted", "Connection refused", "Not connected", "Already connected", "Connection closed", "Initialization error (interapplication manager)", "Bad occurrence", "Wait on unbound occurrence handler", "Occurrence queue overflow", "Datalog type conflict", "Unused", "Unrecognized type (interapplication manager)", "Memory corrupt", "Failed to make temporary DLL", "Old CIN version", "Drag socket not found", "Failed to load drop-object", "Failed to register OLE object", "Failed to release OLE object", "Format specifier type mismatch", "Unknown format specifier", "Too few format specifiers", "Too many format specifiers", "Scan failed", "Newer CIN version", "Error converting to variant", "Runtime menu error", "Password tampered", "Variant attribute not found", "Incompatible variant data type", "Event data is not available", "Event Store is not present", "Occurrence is not found", "Event Queue is not created", "Event info is not available", "Refnum passed is NULL", "Error retrieving Class GUID", "Error retrieving CoClass GUID", "Error retrieving TypeLib GUID.", "Bad built application magic bytes.", "Specific driver is different from the specific driver associated with the Logical Name.", "There is no session opened to the class driver.", "Max Error", "MAX - Error with config objects", "MAX - Error loading configuration", "MAX - Group not supported"]
            # "Current State"
            # "Do not delete, rename, or modify this frame.\n(this is used to capture unhandled states and typos)"
            # "Handle mistyped state name (developer tool)"
            n251 = Format Into String(format string="Software Exception: Unhandled State \"%s\"." ("message"), error in=w466, w461) -> (resulting string=w469:string, error out=w468:errorcluster)  [unwired: 1 in]
            n252 = call <vilib>:"Error Cluster From Error Code.vi"("show call chain? (False)"=TRUE, "error in (no error)"=w468, "error message (\"\")"=w469, "error code (0)"=w470) -> ("error out"=w467:errorcluster)  [unwired: 5 in]
            n253 = call <vilib>:"Add State(s) to Queue__jki_lib_state_machine.vi"("State(s) in (\"\")"=w465) -> ("States Out"=w464:string)  [unwired: 14 in]
          }
          frame "Initialize Core Data" {
            # "Do not delete, rename, or modify this frame.\n(this is used to determine panel behavior on exit)"
            # "originally closed?"
            # "exe?"
            # "If panel starts closed or is an EXE, then close it when we exit"
            n254 = property class="VI"() -> ("Front Panel.Open"=w480:bool)  [unwired: 2 in, 2 out]
            n255 = property class="App"() -> ("App.Kind"=w479:T15)  [unwired: 2 in, 2 out]
            n256 = control-ref of="Current VI Reference"() -> (w474:refnum<vi>)
            n257 = Not(x=w480) -> (.not. x?=w477:bool)
            n258 = Equal?(x=w479, y=T15."Run Time System" ("Application:Kind")) -> (x = y?=w476:bool)
            n259 = Or(x=w477, y=w476) -> (x .or. y?=w475:bool)
            n260 = Bundle By Name(cluster=w473, "Core.Current VI Reference"=w474, "Core.Close Panel on Exit?"=w475) -> (w472:T36)
            n261 = call <vilib>:"Add State(s) to Queue__jki_lib_state_machine.vi"("State(s) in (\"\")"=w483) -> ("States Out"=w482:string)  [unwired: 14 in]
          }
          frame "Error Handler" {
            # "Unhandled Error -- Display it"
            # "Handle any errors here.\nYou can also output any states to clean-up after errors occur"
            # "Clear error"
            n262 = call <vilib>:"General Error Handler.vi"("error in (no error)"=w485) -> ()  [unwired: 10 in, 5 out]
            n263 = call <vilib>:"Add State(s) to Queue__jki_lib_state_machine.vi"("State(s) in Front (\"\")"="/* Post Error States", "State(s) in (\"\")"=w489) -> ("States Out"=w488:string)  [unwired: 13 in]
          }
          frame "Exit" {
            # "Do not put any code in this frame.\n(No errors that occur here will be handled.)"
            n264 = call <vilib>:"Add State(s) to Queue__jki_lib_state_machine.vi"("State(s) in (\"\")"=w494) -> ("States Out"=w493:string)  [unwired: 14 in]
          }
          frame "---------- Data ----------" {
            # "Do not put any code in this frame.\n(It is a separator no-op. You can make a copy of this frame to create a new Data frame)"
            n265 = call <vilib>:"Add State(s) to Queue__jki_lib_state_machine.vi"("State(s) in (\"\")"=w498) -> ("States Out"=w497:string)  [unwired: 14 in]
          }
          frame "Data: Initialize" {
            w514 = bool[] [FALSE, FALSE, FALSE, FALSE, FALSE, FALSE, FALSE, FALSE, FALSE, FALSE, FALSE, TRUE]  # speedmode Y
            w515 = bool[] [FALSE, FALSE, FALSE, FALSE, FALSE, FALSE, FALSE, FALSE, FALSE, FALSE, FALSE, TRUE]  # speedmode X
            w517 = cluster{"Lower value":sgl, "Upper value":sgl}[] [{"Lower value"=93.0, "Upper value"=255.0}, {"Lower value"=105.0, "Upper value"=255.0}, {"Lower value"=0.0, "Upper value"=255.0}, {"Lower value"=127.0, "Upper value"=255.0}, {"Lower value"=0.0, "Upper value"=255.0}, {"Lower value"=0.0, "Upper value"=255.0}, {"Lower value"=0.0, "Upper value"=255.0}, {"Lower value"=0.0, "Upper value"=255.0}, {"Lower value"=0.0, "Upper value"=255.0}, {"Lower value"=0.0, "Upper value"=255.0}, {"Lower value"=0.0, "Upper value"=255.0}, {"Lower value"=0.0, "Upper value"=255.0}]  # thresholds
            w524 = FALSE  # Feedback global
            w526 = 0  # active ccd
            w510 = 2  # img to avg
            w537 = T37 {"Current VI Reference"=refnum, "Close Panel on Exit?"=FALSE}  # Core
            # "Initialize the shift-register data, here.\n(data names are defined by what you wire into the bundle function)"
            n266 = TDMS Open(6:FALSE ("disable buffering (T)"), 7:enum16{"1.0", "2.0"}."2.0" ("file format version (2.0)"), 8:w502, 10:T16."create or replace" ("operation"), 11:w500) -> (0:w506:errorcluster, 3:w507:refnum<k34>)  [unwired: 2 in]
            n267 = call "TDMSbuffersize.vi"("error in (no error)"=w506, "Data Value Reference in"=w507) -> ("error out"=w501:errorcluster, "Data Value Reference out"=w499:refnum<k34>)  [unwired: 8 in]
            n268 = call <vilib>:"Add State(s) to Queue__jki_lib_state_machine.vi"("State(s) in (\"\")"=w539) -> ("States Out"=w538:string)  [unwired: 14 in]
            n269 = Bundle("Core"=w537, "detection para"="detection para", "thresholds"=w517, "Centroid X"="Centroid X", "Centroid Y"="Centroid Y", "img to avg"=w510, "Mean Centroid X"="Mean Centroid X", "Mean Centroid Y"="Mean Centroid Y", "Offset X"="Offset X", "Offset Y"="Offset Y", "Offset X stats"="Offset X stats", "Offset Y stats"="Offset Y stats", "Size"="Size", "Mean Size"="Mean Size", "Time"="Time", "move properties"="move properties", "active axis refs 2"="active axis refs 2", "active ccd"=w526, "Feedback global"=w524, "Motor X"="Motor X", "Motor Y"="Motor Y", "active cams"="active cams", "Data Value Reference out"=w499, "active man refs"="active man refs", "speedmode X"=w515, "speedmode Y"=w514) -> (w509:T36)  [unwired: 1 in]
            n270 = Initialize Array(0.0 ("element"), 12 ("dimension size"), w510) -> (w513:dbl[][])
            n271 = Bundle By Name(cluster=w509, "Centroid X"=w513, "Centroid Y"=w513, "Size"=w513) -> (w508:T36)
          }
          frame "Data: Cleanup" {
            # "Cleanup any data and references, here.\n(this is called automatically, by the Macro: Exit)"
            n272 = Unbundle By Name(w540) -> ("Core.Current VI Reference"=w541:refnum<vi>)
            n273 = Close Reference(reference=w541, error in (no error)=w543) -> (error out=w542:errorcluster)
            n274 = call <vilib>:"Add State(s) to Queue__jki_lib_state_machine.vi"("State(s) in (\"\")"=w545) -> ("States Out"=w544:string)  [unwired: 14 in]
          }
          frame "---------- UI ----------" {
            # "Do not put any code in this frame.\n(It is a separator no-op. You can make a copy of this frame to create a new UI frame)"
            n275 = call <vilib>:"Add State(s) to Queue__jki_lib_state_machine.vi"("State(s) in (\"\")"=w549) -> ("States Out"=w548:string)  [unwired: 14 in]
          }
          frame "UI: Initialize" {
            # "Initialize the User Interface, here.\n(this is called automatically, by the Macro: Init)"
            n276 = call <vilib>:"Add State(s) to Queue__jki_lib_state_machine.vi"("State(s) in (\"\")"=w553) -> ("States Out"=w552:string)  [unwired: 14 in]
          }
          frame "UI: Cursor Set" {
            # "Argument"
            # "Set and Unset Cursor Busy.\n(Usage: \"UI: Cursor Set >> Busy|Idle\")"
            n277 = case shown="\"Idle\", Default" w554 {
              tunnel: w556 -> [w561 w563]
              tunnel: [w560 w562] -> w555
              frame "Idle", Default {
                n278 = call <vilib>:"Unset Busy.vi"("error in (no error)"=w561) -> ("error out"=w560:errorcluster)  [unwired: 10 in]
              }
              frame "Busy" {
                n279 = call <vilib>:"Set Busy.vi"("error in (no error)"=w563) -> ("error out"=w562:errorcluster)  [unwired: 9 in, 1 out]
              }
            }
            n280 = call <vilib>:"Add State(s) to Queue__jki_lib_state_machine.vi"("State(s) in (\"\")"=w559) -> ("States Out"=w558:string)  [unwired: 14 in]
          }
          frame "UI: Front Panel State" {
            # "Argument"
            # "Set Front Panel Open or Closed\n(Usage: \"UI: Front Panel State >> Open|Close\")"
            n281 = Unbundle By Name(w564) -> ("Core.Current VI Reference"=w566:refnum<vi>)
            n282 = case shown="\"Open\", Default" w565 {
              tunnel: w568 -> [w574 w585]
              tunnel: [w575 w586] -> w567
              tunnel: w566 -> [_ _]
              frame "Open", Default {
                n283 = property class="VI"(error in=w574) -> (reference out=w572:refnum<vi>, error out=w573:errorcluster, "Front Panel.Open"=w571:bool)  [unwired: 1 in]
                n284 = case shown="False" w571 {
                  tunnel: [w578 w581] -> w575
                  tunnel: w573 -> [w577 w581]
                  tunnel: w572 -> [w576 _]
                  frame False {
                    n285 = invoke class="VI" method="FP.Open"(reference=w576, error in=w577, "Activate"=TRUE, "State"=T17."Standard") -> (error out=w578:errorcluster)  [unwired: 1 in, 4 out]
                  }
                  frame True {
                  }
                }
              }
              frame "Close" {
                n286 = property class="VI"(error in=w585) -> (reference out=w583:refnum<vi>, error out=w584:errorcluster, "Front Panel.Open"=w582:bool)  [unwired: 1 in]
                n287 = case shown="True" w582 {
                  tunnel: [w587 w590] -> w586
                  tunnel: w584 -> [w587 w589]
                  tunnel: w583 -> [_ w588]
                  frame False {
                  }
                  frame True {
                    n288 = invoke class="VI" method="FP.Close"(reference=w588, error in=w589) -> (error out=w590:errorcluster)  [unwired: 1 in, 2 out]
                  }
                }
              }
            }
            n289 = call <vilib>:"Add State(s) to Queue__jki_lib_state_machine.vi"("State(s) in (\"\")"=w570) -> ("States Out"=w569:string)  [unwired: 14 in]
          }
          frame "---------- Macro ----------" {
            # "Do not put any code in this frame.\n(It is a separator no-op. You can make a copy of this frame to create a new Macro frame)"
            n290 = call <vilib>:"Add State(s) to Queue__jki_lib_state_machine.vi"("State(s) in (\"\")"=w594) -> ("States Out"=w593:string)  [unwired: 14 in]
          }
          frame "Macro: Initialize" {
            # "Initialization Macro\n(This is called once, when the VI starts)"
            n291 = property on="img to avg" class="DigNum (strict)"() -> ("Value"=w596:i32)  [unwired: 2 in, 2 out]
            n292 = Number To Decimal String(number=w596) -> (decimal integer string=w598:string)  [unwired: 1 in]
            n293 = call <vilib>:"Build State String with Arguments__jki_lib_state_machine.vi"("Arguments (\"\")"=w598, "State"="ImgToAvg") -> ("State with Arguments"=w595:string)  [unwired: 4 in]
            n294 = call <vilib>:"Add State(s) to Queue__jki_lib_state_machine.vi"("State(s) in Front (\"\")"="Data: Initialize\nInitialize Core Data\nUI: Initialize\nUI: Front Panel State >> Open\nDevice Ini >> 3000", "State(s) in (\"\")"=w603, "State(s) at Back (\"\")"=w595) -> ("States Out"=w602:string)  [unwired: 12 in]
          }
          frame "Macro: Exit" {
            # "Exit Macro\n(This is called once, when the VI exits)"
            n295 = Unbundle By Name(w605) -> ("Core.Close Panel on Exit?"=w604:bool)
            n296 = Select(t="UI: Front Panel State >> Close", s=w604, f="") -> (s? t:f=w608:string)
            n297 = call <vilib>:"Add State(s) to Queue__jki_lib_state_machine.vi"("State(s) in (\"\")"=w608, "State(s) at Back (\"\")"="Data: Cleanup\nExit") -> ("States Out"=w606:string)  [unwired: 13 in]
            n298 = call <vilib>:"Add State(s) to Queue__jki_lib_state_machine.vi"("State(s) in Front (\"\")"=w606, "State(s) in (\"\")"=w613) -> ("States Out"=w612:string)  [unwired: 13 in]
          }
          frame "---------- Ini and Configure ----------" {
            # "Template Separator\n(You can make a copy of, or modify, this frame)"
            n299 = call <vilib>:"Add State(s) to Queue__jki_lib_state_machine.vi"("State(s) in (\"\")"=w617) -> ("States Out"=w616:string)  [unwired: 14 in]
          }
          frame "Device Ini" {
            # "Your code here.\n(You can make a copy of, or modify, this frame)"
            n300 = Empty String/Path?(string/path=w634) -> (empty?=w633:bool)
            n301 = case shown="False" w633 {
              tunnel: w634 -> [w675 _]
              tunnel: [w674 0] -> w632
              frame False {
                n302 = Decimal String To Number(string=w675) -> (number=w674:i32)  [unwired: 2 in, 1 out]
              }
              frame True {
              }
            }
            n303 = flat-sequence {
              tunnel: w640 -> [w678]
              tunnel: [w678] -> w639
              tunnel: w632 -> [w677]
              tunnel: w639 -> [w681]
              tunnel: [w679] -> w623
              frame #0 {
                n304 = Wait (ms)(milliseconds to wait=w677) -> ()  [unwired: 1 out]
              }
              frame #1 {
                n305 = for {
                  tunnel: w681 -> [w683] mode=indexing
                  shift-right: [w684] -> w679
                  shift-left: string[] [] -> [w685]
                  n306 = call "send command.vi"("Device Name"=w683) -> ("status"=w686:bool)  [unwired: 4 in]
                  n307 = Wait (ms)(milliseconds to wait=u32 5) -> ()  [unwired: 1 out]
                  n308 = case shown="True" w686 {
                    tunnel: w685 -> [w687 w690]
                    tunnel: [w687 w689] -> w684
                    tunnel: w683 -> [_ w688]
                    frame False {
                    }
                    frame True {
                      n309 = Build Array (concatenate)(w690, w688) -> (w689:string[])
                    }
                  }
                }
              }
            }
            n310 = Unbundle By Name(w631) -> ("active cams"=w624:string[])
            n311 = call <vilib>:"Add State(s) to Queue__jki_lib_state_machine.vi"("State(s) in (\"\")"=w641) -> ("States Out"=w626:string)  [unwired: 14 in]
            n312 = Equal?(x=w624, y=w623) -> (x = y?=w630:bool[])
            n313 = Empty Array?(array=w624) -> (empty?=w629:bool)
            n314 = Not(x=w629) -> (.not. x?=w628:bool)
            n315 = Build Array (concatenate)(w630, w628) -> (w627:bool[])
            n316 = Array Size(array=w623) -> (size(s)=w622:i32)
            n317 = Array Size(array=w624) -> (size(s)=w621:i32)
            n318 = And Array Elements(Boolean array=w627) -> (logical AND=w619:bool)
            n319 = Equal?(x=w622, y=w621) -> (x = y?=w620:bool)
            n320 = And(x=w620, y=w619) -> (x .and. y?=w618:bool)
            n321 = case shown="False" w618 {
              tunnel: [w656 w673] -> w638
              tunnel: w637 -> [_ _]
              tunnel: w636 -> [w653 w672]
              tunnel: [w653 w672] -> w635
              tunnel: w631 -> [w649 w673]
              tunnel: w623 -> [w650 _]
              tunnel: w626 -> [w655 w671]
              tunnel: [w642 w671] -> w625
              frame False {
                n322 = property on="active CCDs" class="LstBox (strict)"("Item Names"=w650) -> ()  [unwired: 2 in, 2 out]
                n323 = Array Size(array=w650) -> (size(s)=w663:i32)
                n324 = Initialize Array(0.0 ("element"), w663, 0 ("dimension size")) -> (w658:dbl[][])
                n325 = Unbundle By Name(w649) -> ("img to avg"=w648:i32)
                n326 = Bundle By Name(cluster=w649, "active cams"=w650) -> (w657:T36)
                n327 = Initialize Array(0.0 ("element"), 12 ("dimension size"), w648) -> (w647:dbl[][])
                n328 = Bundle By Name(cluster=w657, "Offset X stats"=w658, "Offset Y stats"=w658, "Centroid X"=w647, "Centroid Y"=w647, "Mean Centroid X"=w658, "Mean Centroid Y"=w658, "Offset X"=w658, "Offset Y"=w658, "Size"=w647, "Mean Size"=w658, "Motor X"=w658, "Motor Y"=w658) -> (w656:T36)
                n329 = for {
                  N: 1 -> [_]
                  shift-right: [w665] -> w661
                  shift-left: timestamp[][] [] ("Time") -> [w667]
                  n330 = for {
                    N: 12 -> [_]
                    tunnel: w667 -> [w670] mode=indexing
                    tunnel: [w668] -> w665 mode=indexing
                    n331 = Get Date/Time In Seconds() -> (seconds since 1Jan1904=w669:timestamp)
                    n332 = Build Array (concatenate)(w670, w669) -> (w668:timestamp[])
                  }
                }
                n333 = property on="config path" class="Str"() -> ("Value"=w645:string)  [unwired: 2 in, 2 out]
                n334 = call <vilib>:"Add State(s) to Queue__jki_lib_state_machine.vi"("State(s) in Front (\"\")"="newtdms\nMove Config\nMotor Config\nDetection Config\nactive\nCenter" ("State(s) in Front (\"\")"), "State(s) in (\"\")"=w655) -> ("States Out"=w644:string)  [unwired: 13 in]
                n335 = call <vilib>:"Build State String with Arguments__jki_lib_state_machine.vi"("Arguments (\"\")"=w645, "State"="Load Config" ("State(s) in Front (\"\")")) -> ("State with Arguments"=w643:string)  [unwired: 4 in]
                n336 = call <vilib>:"Add State(s) to Queue__jki_lib_state_machine.vi"("State(s) in Front (\"\")"=w643, "State(s) in (\"\")"=w644) -> ("States Out"=w642:string)  [unwired: 13 in]
                n337 = property on="Time" class="Arr (strict)"("Value"=w661) -> ()  [unwired: 2 in, 2 out]
                "name array" <- w650
              }
              frame True {
              }
            }
          }
          frame "Load Config" {
            # "Your code here.\n(You can make a copy of, or modify, this frame)"
            n338 = Unbundle By Name(w731) -> ("detection para"=w737:T3[], "move properties"=w734:T2[], "thresholds"=w727:cluster{"Lower value":sgl, "Upper value":sgl}[])
            n339 = Empty String/Path?(string/path=w693) -> (empty?=w692:bool)
            n340 = case shown="True" w692 {
              tunnel: [w747 T5 {"CCDs"=[], "move properties"=[], "detection para"=[], "thresholds"=[], "Value"={"Motor CCD 1"=0, "Motor CCD 2"=0, "Motor CCD 3"=0, "Motor CCD 4"=0, "Motor CCD 5"=0, "Motor CCD 6"=0, "Motor CCD 7"=0, "Motor CCD 8"=0, "Motor CCD 9"=0, "Motor CCD 10"=0, "Motor CCD 11"=0, "Motor CCD 12"=0}} ("output cluster 2")] -> w739
              tunnel: [w745 w754] -> w697
              tunnel: w694 -> [w744 w754]
              tunnel: w693 -> [w743 _]
              frame False {
                n341 = String To Path(string=w743) -> (path=w742:path)
                n342 = Open/Create/Replace File(file path (use dialog)=w742, error in=w744, operation (0:open)=T18."open or create") -> (refnum out=w749:refnum<file>, error out=w750:errorcluster)  [unwired: 3 in, 1 out]
                n343 = Read from Binary File(5:"output cluster 2", 8:w750, 11:w749) -> (0:w751:errorcluster, 2:w747:T5, 3:w752:refnum<file>)  [unwired: 3 in, 1 out]
                n344 = Close File(refnum=w752, error in=w751) -> (error out=w745:errorcluster)  [unwired: 1 out]
              }
              frame True {
              }
            }
            n345 = property on="Load Config" class="Bool (strict)"("Value"=FALSE ("Load Config")) -> ()  [unwired: 2 in, 2 out]
            n346 = Unbundle By Name(w739) -> ("Value"=w724:T7, "CCDs"=w738:string[], "detection para"=w736:T3[], "move properties"=w735:T2[], "thresholds"=w728:cluster{"Lower value":sgl, "Upper value":sgl}[])
            n347 = Cluster To Array(cluster=w724) -> (array=w725:u16[])
            n348 = call <vilib>:"Add State(s) to Queue__jki_lib_state_machine.vi"("State(s) in (\"\")"=w741, "State(s) at Back (\"\")"="Motor Config" ("State(s) at Back (\"\")")) -> ("States Out"=w740:string)  [unwired: 13 in]
            n349 = for {
              tunnel: w738 -> [w770]
              tunnel: w736 -> [w772]
              tunnel: w735 -> [w771]
              shift-right: [w764] -> w733
              shift-left: w737 -> [w769]
              shift-right: [w762] -> w732
              shift-left: w734 -> [w768]
              tunnel: w729 -> [w767] mode=indexing
              tunnel: w728 -> [w763]
              shift-right: [w759] -> w726
              shift-left: w727 -> [w761]
              tunnel: w725 -> [w758]
              tunnel: [w755] -> w723 mode=indexing
              i -> [w756]
              n350 = call-poly <userlib>:"Filter 1D Array__ogtk.vi"("items to filter"=w767, "array"=w770) -> ("filtered item indices"=w773:i32[])  [unwired: 4 in, 1 out]
              n351 = Index Array(array=w773) -> (element=w757:i32)  [unwired: 1 in]
              n352 = Index Array(array=w758, index=w757) -> (element=w755:u16)
              n353 = Index Array(array=w772, index=w757) -> (element=w766:T3)
              n354 = Index Array(array=w771, index=w757) -> (element=w765:T2)
              n355 = Index Array(array=w763, index=w757) -> (element=w760:cluster{"Lower value":sgl, "Upper value":sgl})
              n356 = Replace Array Subset(array=w769, new element=w766, index=w756) -> (w764:T3[])
              n357 = Replace Array Subset(array=w768, new element=w765, index=w756) -> (w762:T2[])
              n358 = Replace Array Subset(array=w761, new element=w760, index=w756) -> (w759:cluster{"Lower value":sgl, "Upper value":sgl}[])
            }
            n359 = Index Array(array=w723, index #1=0 ("index (row)"), index #2=1 ("index (row)"), index #3=2 ("index (row)"), index #4=3 ("index (row)"), index #5=4 ("index (row)"), index #6=5 ("index (row)"), index #7=6 ("index (row)"), index #8=7 ("index (row)"), index #9=8 ("index (row)"), index #10=9 ("index (row)"), index #11=10 ("index (row)"), index #12=11 ("index (row)")) -> (element #1=w710:u16, element #2=w709:u16, element #3=w708:u16, element #4=w707:u16, element #5=w706:u16, element #6=w705:u16, element #7=w704:u16, element #8=w703:u16, element #9=w702:u16, element #10=w701:u16, element #11=w700:u16, element #12=w699:u16)
            n360 = Bundle By Name(cluster=w724, "Motor CCD 1"=w710, "Motor CCD 2"=w709, "Motor CCD 3"=w708, "Motor CCD 4"=w707, "Motor CCD 5"=w706, "Motor CCD 6"=w705, "Motor CCD 7"=w704, "Motor CCD 8"=w703, "Motor CCD 9"=w702, "Motor CCD 10"=w701, "Motor CCD 11"=w700, "Motor CCD 12"=w699) -> (w698:T7)
            n361 = Bundle By Name(cluster=w731, "detection para"=w733, "move properties"=w732, "thresholds"=w726) -> (w730:T36)
            n362 = property on="associated motors" class="Clust (strict)"(error in=w697, "Val(Sgnl)"=w698) -> (error out=w696:errorcluster)  [unwired: 1 in, 1 out]
          }
          frame "Save Config" {
            # "Your code here.\n(You can make a copy of, or modify, this frame)"
            n363 = Unbundle By Name(w791) -> ("move properties"=w777:T2[], "detection para"=w786:T3[], "thresholds"=w774:cluster{"Lower value":sgl, "Upper value":sgl}[])
            n364 = property on="associated motors" class="Clust (strict)"() -> ("Value"=w785:T7)  [unwired: 2 in, 2 out]
            n365 = property on="Save Config" class="Bool (strict)"("Value"=FALSE ("Save Config")) -> ()  [unwired: 2 in, 2 out]
            n366 = local read "CCDs"() -> (w775:string[])
            n367 = call "File Dialog"("pattern (all files)"="*.cfg", "pattern label"="config") -> ("selected path"=w779:path)  [unwired: 10 in, 3 out]
            n368 = Bundle("CCDs"=w775, "move properties"=w777, "detection para"=w786, "thresholds"=w774, "Value"=w785) -> (w778:T5)  [unwired: 1 in]
            n369 = Open/Create/Replace File(file path (use dialog)=w779, error in=w783, operation (0:open)=T18."replace or create with confirmation") -> (refnum out=w787:refnum<file>, error out=w788:errorcluster)  [unwired: 3 in, 1 out]
            n370 = Write to Binary File(file (use dialog)=w787, data=w778, error in=w788) -> (refnum out=w790:refnum<file>, error out=w789:errorcluster)  [unwired: 3 in, 1 out]
            n371 = Close File(refnum=w790, error in=w789) -> (error out=w782:errorcluster)  [unwired: 1 out]
            n372 = call <vilib>:"Add State(s) to Queue__jki_lib_state_machine.vi"("State(s) in (\"\")"=w793) -> ("States Out"=w792:string)  [unwired: 14 in]
          }
          frame "active" {
            # "Your code here.\n(You can make a copy of, or modify, this frame)"
            n373 = Empty String/Path?(string/path=w808) -> (empty?=w807:bool)
            n374 = Unbundle By Name(w804) -> ("move properties"=w820:T2[], "detection para"=w816:T3[])  [unwired: 1 out]
            n375 = Unbundle By Name(w804) -> ("active axis refs 2"=w803:T11)
            n376 = call-poly <userlib>:"Filter 1D Array__ogtk.vi"("items to filter"=w808, "array"=w818) -> ("filtered item indices"=w821:i32[])  [unwired: 4 in, 1 out]
            n377 = Index Array(array=w821) -> (element=w805:i32)  [unwired: 1 in]
            n378 = Select(t=0, s=w807, f=w805) -> (s? t:f=w801:i32)
            n379 = Index Array(array=w803, index=w801) -> (element=w802:cluster{"Ref X":refnum<vi>, "Ref Y":refnum<vi>})
            n380 = Unbundle By Name(w802) -> ("Ref X"=w800:refnum<vi>, "Ref Y"=w799:refnum<vi>)
            n381 = Index Array(array=w820, index=w801) -> (element=w819:T2)
            n382 = Index Array(array=w816, index=w801) -> (element=w815:T3)
            n383 = property on="move config" class="Clust (strict)"(error in=w811, "Value"=w819) -> (error out=w809:errorcluster)  [unwired: 1 in, 1 out]
            n384 = property on="beam detection para" class="Clust (strict)"(error in=w809, "Value"=w815) -> (error out=w810:errorcluster)  [unwired: 1 in, 1 out]
            n385 = call <vilib>:"Add State(s) to Queue__jki_lib_state_machine.vi"("State(s) in (\"\")"=w823) -> ("States Out"=w822:string)  [unwired: 14 in]
            n386 = property class="DigNum (strict)"(reference=w800, error in=w810) -> (error out=w796:errorcluster, "Value"=w798:dbl)  [unwired: 1 out]
            n387 = Bundle By Name(cluster="active Axis ref 3", "Ref X"=w800, "Ref Y"=w799) -> (w813:cluster{"Ref X":refnum<vi>, "Ref Y":refnum<vi>})
            n388 = Bundle By Name(cluster=w804, "active ccd"=w801, "active man refs"=w813) -> (w817:T36)
            n389 = property on="Position 1" class="DigNum (strict)"(error in=w796, "Value"=w798) -> (error out=w795:errorcluster)  [unwired: 1 in, 1 out]
            n390 = property class="DigNum (strict)"(reference=w799, error in=w795) -> (error out=w794:errorcluster, "Value"=w797:dbl)  [unwired: 1 out]
            n391 = property on="Position 2" class="DigNum (strict)"(error in=w794, "Value"=w797) -> (error out=w812:errorcluster)  [unwired: 1 in, 1 out]
          }
          frame "Detection Config" {
            # "Your code here.\n(You can make a copy of, or modify, this frame)"
            n392 = Unbundle By Name(w828) -> ("detection para"=w824:T3[], "active ccd"=w829:i32)
            n393 = Replace Array Subset(array=w824, new element="beam detection para", index=w829) -> (w825:T3[])
            n394 = Bundle By Name(cluster=w828, "detection para"=w825) -> (w827:T36)
            n395 = call <vilib>:"Add State(s) to Queue__jki_lib_state_machine.vi"("State(s) in (\"\")"=w832) -> ("States Out"=w831:string)  [unwired: 14 in]
          }
          frame "Motor Config" {
            # "Your code here.\n(You can make a copy of, or modify, this frame)"
            n396 = Unbundle By Name("associated motors") -> ("Motor CCD 1"=w849:u16, "Motor CCD 2"=w850:u16, "Motor CCD 3"=w851:u16, "Motor CCD 4"=w844:u16, "Motor CCD 5"=w843:u16, "Motor CCD 6"=w842:u16, "Motor CCD 7"=w841:u16, "Motor CCD 8"=w840:u16, "Motor CCD 9"=w839:u16, "Motor CCD 10"=w838:u16, "Motor CCD 11"=w837:u16, "Motor CCD 12"=w836:u16)
            n397 = Build Array(w849, w850, w851, w844, w843, w842, w841, w840, w839, w838, w837, w836) -> (w835:u16[])
            n398 = local read "motor refs"() -> (w847:refnum<vi>[])
            n399 = Increment(x=w835) -> (x+1=w834:u16[])
            n400 = for {
              tunnel: w834 -> [w866] mode=indexing
              tunnel: w847 -> [w861]
              tunnel: [w855] -> w833 mode=indexing
              n401 = Multiply(x=w866, y=u16 2) -> (x*y=w862:u16)
              n402 = Subtract(x=w862, y=u16 2) -> (x-y=w860:u16)
              n403 = Subtract(x=w862, y=u16 1) -> (x-y=w859:u16)
              n404 = Index Array(array=w861, index=w860) -> (element=w858:refnum<vi>)
              n405 = Index Array(array=w861, index=w859) -> (element=w857:refnum<vi>)
              n406 = Bundle By Name(cluster="active Axis ref", "Ref X"=w858, "Ref Y"=w857) -> (w855:cluster{"Ref X":refnum<vi>, "Ref Y":refnum<vi>})
            }
            n407 = call <vilib>:"Add State(s) to Queue__jki_lib_state_machine.vi"("State(s) in (\"\")"=w854) -> ("States Out"=w853:string)  [unwired: 14 in]
            n408 = Bundle By Name(cluster=w846, "active axis refs 2"=w833) -> (w845:T36)
          }
          frame "Move Config" {
            # "Your code here.\n(You can make a copy of, or modify, this frame)"
            n409 = Unbundle By Name(w868) -> ("move properties"=w872:T2[], "active ccd"=w871:i32)
            n410 = Replace Array Subset(array=w872, new element="move config", index=w871) -> (w869:T2[])
            n411 = Bundle By Name(cluster=w868, "move properties"=w869) -> (w867:T36)
            n412 = call <vilib>:"Add State(s) to Queue__jki_lib_state_machine.vi"("State(s) in (\"\")"=w875) -> ("States Out"=w874:string)  [unwired: 14 in]
          }
          frame "----------Centroid & Move----------" {
            # "Template Separator\n(You can make a copy of, or modify, this frame)"
            n413 = call <vilib>:"Add State(s) to Queue__jki_lib_state_machine.vi"("State(s) in (\"\")"=w879) -> ("States Out"=w878:string)  [unwired: 14 in]
          }
          frame "detected" {
            n414 = Unbundle By Name(w884) -> ("Offset X"=w919:dbl[][], "Offset Y"=w918:dbl[][], "Size"=w917:dbl[][], "Mean Size"=w916:dbl[][], "Time"=w913:timestamp[][], "Motor X"=w893:dbl[][], "active axis refs 2"=w892:T11, "Motor Y"=w891:dbl[][])
            n415 = Spreadsheet String To Array(format string="%s", spreadsheet string=w896, array type (2D Dbl)=string[] []) -> (array=w887:string[])  [unwired: 1 in]
            n416 = for {
              tunnel: w888 -> [w933] mode=indexing
              tunnel: w887 -> [w932]
              tunnel: [w930] -> w886 mode=indexing
              n417 = for {
                tunnel: w933 -> [w936]
                tunnel: [w935] -> w931 mode=indexing
                tunnel: w932 -> [w934] mode=indexing
                n418 = Equal?(x=w936, y=w934) -> (x = y?=w935:bool)
              }
              n419 = Or Array Elements(Boolean array=w931) -> (logical OR=w930:bool)
            }
            n420 = Unbundle By Name(w884) -> ("Mean Centroid X"=w924:dbl[][], "Mean Centroid Y"=w923:dbl[][], "Centroid X"=w926:dbl[][], "Centroid Y"=w925:dbl[][])
            n421 = call <vilib>:"Build State String with Arguments__jki_lib_state_machine.vi"("Arguments (\"\")"=w896, "State"="stats") -> ("State with Arguments"=w897:string)  [unwired: 4 in]
            n422 = call <vilib>:"Add State(s) to Queue__jki_lib_state_machine.vi"("State(s) in Front (\"\")"=w897, "State(s) in (\"\")"=w895) -> ("States Out"=w894:string)  [unwired: 13 in]
            n423 = for {
              tunnel: w926 -> [w986]
              tunnel: w925 -> [w985]
              tunnel: w924 -> [w984]
              tunnel: w923 -> [w983]
              tunnel: [w982] -> w910 mode=indexing
              tunnel: [w981] -> w921 mode=indexing
              tunnel: w920 -> [w980] mode=indexing
              tunnel: w919 -> [w979]
              tunnel: w918 -> [w978]
              tunnel: [w977] -> w885 mode=indexing
              tunnel: [w976] -> w911 mode=indexing
              tunnel: w917 -> [w975]
              tunnel: w916 -> [w974]
              tunnel: [w973] -> w915 mode=indexing
              tunnel: w913 -> [w972]
              tunnel: [w971] -> w912 mode=indexing
              tunnel: w893 -> [w963]
              tunnel: w892 -> [w962]
              tunnel: w891 -> [w961]
              tunnel: [w941] -> w890 mode=indexing
              tunnel: [w940] -> w889 mode=indexing
              tunnel: w886 -> [w939]
              i -> [w938]
              n424 = Unbundle By Name(w980) -> ("Target.X::12"=w945:refnum<vi>, "Target.Y::12"=w944:refnum<vi>)
              n425 = Index Array(array=w963, index (row)=w938) -> (element=w966:dbl[])  [unwired: 1 in]
              n426 = Index Array(array=w962, index=w938) -> (element=w965:cluster{"Ref X":refnum<vi>, "Ref Y":refnum<vi>})
              n427 = Index Array(array=w961, index (row)=w938) -> (element=w970:dbl[])  [unwired: 1 in]
              n428 = Index Array(array=w939, index=w938) -> (element=w937:bool)
              n429 = Index Array(array=w984, index (row)=w938) -> (element=w957:dbl[])  [unwired: 1 in]
              n430 = Index Array(array=w983, index (row)=w938) -> (element=w958:dbl[])  [unwired: 1 in]
              n431 = Index Array(array=w986, index (row)=w938) -> (element=w960:dbl[])  [unwired: 1 in]
              n432 = Index Array(array=w985, index (row)=w938) -> (element=w959:dbl[])  [unwired: 1 in]
              n433 = Index Array(array=w979, index (row)=w938) -> (element=w953:dbl[])  [unwired: 1 in]
              n434 = Index Array(array=w978, index (row)=w938) -> (element=w952:dbl[])  [unwired: 1 in]
              n435 = Index Array(array=w975, index (row)=w938) -> (element=w950:dbl[])  [unwired: 1 in]
              n436 = Index Array(array=w974, index (row)=w938) -> (element=w949:dbl[])  [unwired: 1 in]
              n437 = Index Array(array=w972, index (row)=w938) -> (element=w946:timestamp[])  [unwired: 1 in]
              n438 = Unbundle By Name(w965) -> ("Ref X"=w964:refnum<vi>, "Ref Y"=w968:refnum<vi>)
              n439 = property class="DigNum (strict)"(reference=w945) -> ("Value"=w943:dbl)  [unwired: 1 in, 2 out]
              n440 = property class="DigNum (strict)"(reference=w944) -> ("Value"=w942:dbl)  [unwired: 1 in, 2 out]
              n441 = call <vilib>:"Std Deviation and Variance.vi"("X"=w960) -> ("mean"=w956:dbl)  [unwired: 1 in, 2 out]
              n442 = call <vilib>:"Std Deviation and Variance.vi"("X"=w959) -> ("mean"=w955:dbl)  [unwired: 1 in, 2 out]
              n443 = call <vilib>:"Std Deviation and Variance.vi"("X"=w950) -> ("mean"=w948:dbl)  [unwired: 1 in, 2 out]
              n444 = Get Date/Time In Seconds() -> (seconds since 1Jan1904=w947:timestamp)
              n445 = property class="DigNum (strict)"(reference=w964) -> ("Value"=w967:dbl)  [unwired: 1 in, 2 out]
              n446 = property class="DigNum (strict)"(reference=w968) -> ("Value"=w969:dbl)  [unwired: 1 in, 2 out]
              n447 = Subtract(x=w943, y=w956) -> (x-y=w954:dbl)
              n448 = Subtract(x=w942, y=w955) -> (x-y=w951:dbl)
              n449 = case shown="True" w937 {
                tunnel: [w999 w1018] -> w982
                tunnel: [w987 w1017] -> w981
                tunnel: [w988 w1016] -> w977
                tunnel: [w989 w1015] -> w976
                tunnel: [w990 w1014] -> w973
                tunnel: [w991 w1013] -> w971
                tunnel: w958 -> [w997 w1012]
                tunnel: w957 -> [w998 w1011]
                tunnel: w956 -> [_ w1010]
                tunnel: w955 -> [_ w1009]
                tunnel: w954 -> [_ w1008]
                tunnel: w953 -> [w996 w1007]
                tunnel: w952 -> [w995 w1006]
                tunnel: w951 -> [_ w1005]
                tunnel: w949 -> [w994 w1004]
                tunnel: w948 -> [_ w1003]
                tunnel: w947 -> [w992 w1002]
                tunnel: w946 -> [w993 w1001]
                frame False {
                  w1000 = 0.0
                  n450 = Build Array (concatenate)(w998, w1000) -> (w999:dbl[])
                  n451 = Build Array (concatenate)(w997, w1000) -> (w987:dbl[])
                  n452 = Build Array (concatenate)(w996, w1000) -> (w988:dbl[])
                  n453 = Build Array (concatenate)(w995, w1000) -> (w989:dbl[])
                  n454 = Build Array (concatenate)(w994, w1000) -> (w990:dbl[])
                  n455 = Build Array (concatenate)(w993, w992) -> (w991:timestamp[])
                }
                frame True {
                  n456 = Build Array (concatenate)(w1011, w1010) -> (w1018:dbl[])
                  n457 = Build Array (concatenate)(w1012, w1009) -> (w1017:dbl[])
                  n458 = Build Array (concatenate)(w1007, w1008) -> (w1016:dbl[])
                  n459 = Build Array (concatenate)(w1006, w1005) -> (w1015:dbl[])
                  n460 = Build Array (concatenate)(w1004, w1003) -> (w1014:dbl[])
                  n461 = Build Array (concatenate)(w1001, w1002) -> (w1013:timestamp[])
                }
              }
              n462 = Build Array (concatenate)(w966, w967) -> (w941:dbl[])
              n463 = Build Array (concatenate)(w970, w969) -> (w940:dbl[])
            }
            n464 = local write "Numeric"(0.0 ("Numeric")) -> ()
            n465 = Array Size(array=w885) -> (size(s)=w909:i32[])
            n466 = Index Array(array=w909, index=1) -> (element=w907:i32)
            "History Index" <- w907
            n467 = call <vilib>:"Add State(s) to Queue__jki_lib_state_machine.vi"("State(s) in (\"\")"=w894, "State(s) at Back (\"\")"="Check Move\ntdms" ("State(s) at Back (\"\")")) -> ("States Out"=w901:string)  [unwired: 13 in]
            n468 = Unbundle By Name(w884) -> ("img to avg"=w881:i32)
            n469 = Initialize Array(0.0 ("element"), 12 ("dimension size"), w881) -> (w880:dbl[][])
            n470 = Greater?(x=w907, y="History Size") -> (0:w905:bool)
            n471 = Bundle By Name(cluster=w884, "Centroid X"=w880, "Centroid Y"=w880, "Mean Centroid X"=w910, "Mean Centroid Y"=w921, "Offset X"=w885, "Offset Y"=w911, "Mean Size"=w915, "Size"=w880, "Time"=w912, "Motor X"=w890, "Motor Y"=w889) -> (w922:T36)
            n472 = Select(t="history" ("State(s) at Back (\"\")"), s=w905, f="") -> (s? t:f=w902:string)
            n473 = call <vilib>:"Add State(s) to Queue__jki_lib_state_machine.vi"("State(s) in (\"\")"=w901, "State(s) at Back (\"\")"=w902) -> ("States Out"=w900:string)  [unwired: 13 in]
          }
          frame "Check Move" {
            (unwired) "Device Ini" ("State(s) in Front (\"\")")
            n474 = Unbundle By Name(w1020) -> ("move properties"=w1032:T2[], "Mean Size"=w1031:dbl[][], "move properties"=w1030:T2[], "Offset X"=w1029:dbl[][], "Offset Y"=w1028:dbl[][], "active cams"=w1027:string[])
            n475 = for {
              tunnel: w1030 -> [w1088] mode=indexing
              tunnel: w1029 -> [w1090] mode=indexing
              tunnel: w1028 -> [w1089] mode=indexing
              tunnel: w1031 -> [w1087] mode=indexing
              tunnel: [w1066] -> w1026 mode=indexing
              tunnel: [w1062] -> w1025 mode=indexing
              tunnel: w1027 -> [w1084] mode=indexing
              tunnel: [w1086] -> w1033 mode=indexing
              tunnel: [w1085] -> w1023 mode=indexing
              tunnel: w1032 -> [w1083] mode=indexing
              tunnel: [w1060] -> w1022 mode=indexing
              tunnel: [w1055] -> w1021 mode=indexing
              tunnel: "Speedmode @" -> [w1054]
              n476 = Unbundle By Name(w1083) -> ("enable feedback"=w1065:bool)
              n477 = Unbundle By Name(w1088) -> ("Tolerance [%]"=w1077:dbl)
              n478 = Reverse 1D Array(array=w1090) -> (reversed array=w1082:dbl[])
              n479 = Reverse 1D Array(array=w1089) -> (reversed array=w1081:dbl[])
              n480 = Reverse 1D Array(array=w1087) -> (reversed array=w1076:dbl[])
              n481 = Index Array(array=w1082) -> (element=w1080:dbl)  [unwired: 1 in]
              n482 = Index Array(array=w1081) -> (element=w1079:dbl)  [unwired: 1 in]
              n483 = Index Array(array=w1076) -> (element=w1075:dbl)  [unwired: 1 in]
              n484 = Absolute Value(x=w1080) -> (abs(x)=w1061:dbl)
              n485 = Absolute Value(x=w1079) -> (abs(x)=w1058:dbl)
              n486 = Square Root(x=w1075) -> (sqrt(x)=w1074:dbl)
              n487 = Divide(x=w1077, y=100.0) -> (x/y=w1073:dbl)
              n488 = Multiply(x=w1074, y=w1073) -> (x*y=w1057:dbl)
              n489 = Not Equal To 0?(x=w1058) -> (x != 0?=w1063:bool)
              n490 = Not Equal To 0?(x=w1061) -> (x != 0?=w1068:bool)
              n491 = Greater Or Equal?(x=w1061, y=w1057) -> (x >= y?=w1067:bool)
              n492 = Greater Or Equal?(x=w1058, y=w1057) -> (x >= y?=w1064:bool)
              n493 = Divide(x=w1061, y=w1057) -> (x/y=w1059:dbl)
              n494 = Divide(x=w1058, y=w1057) -> (x/y=w1056:dbl)
              n495 = Compound Arithmetic op=AND(w1065, w1068, w1067) -> (w1066:bool)
              n496 = Compound Arithmetic op=AND(w1065, w1064, w1063) -> (w1062:bool)
              n497 = Boolean To (0,1)(Boolean=w1062) -> (0, 1=w1069:i16)
              n498 = Greater?(x=w1059, y=w1054) -> (0:w1060:bool)
              n499 = Greater?(x=w1056, y=w1054) -> (0:w1055:bool)
              n500 = Multiply(x=w1069, y=w1058) -> (x*y=w1070:dbl)
              n501 = Boolean To (0,1)(Boolean=w1066) -> (0, 1=w1072:i16)
              n502 = Multiply(x=w1072, y=w1061) -> (x*y=w1071:dbl)
              n503 = Bundle(w1070, "GUIdevice 8"=w1084) -> (w1085:cluster{dbl, "GUIdevice 8":string})  [unwired: 1 in]
              n504 = Bundle(w1071, "GUIdevice 8"=w1084) -> (w1086:cluster{dbl, "GUIdevice 8":string})  [unwired: 1 in]
            }
            "required X" <- w1026
            "required Y" <- w1025
            "speedmode X" <- w1022
            "speedmode Y" <- w1021
            n505 = case shown="True" "Align" {
              tunnel: w1033 -> [w1096 w1101]
              tunnel: w1023 -> [w1095 w1098]
              tunnel: [w1094 w1100] -> w1036
              tunnel: [w1093 w1097] -> w1035
              frame False {
                n506 = Sort 1D Array(array=w1095) -> (sorted array=w1092:cluster{dbl, "GUIdevice 8":string}[])
                n507 = Sort 1D Array(array=w1096) -> (sorted array=w1091:cluster{dbl, "GUIdevice 8":string}[])
                n508 = Reverse 1D Array(array=w1092) -> (reversed array=w1093:cluster{dbl, "GUIdevice 8":string}[])
                n509 = Reverse 1D Array(array=w1091) -> (reversed array=w1094:cluster{dbl, "GUIdevice 8":string}[])
              }
              frame True {
                w1099 = cluster{dbl, "GUIdevice 8":string}[] [] ("Array")
                n510 = for {
                  shift-right: [w1111] -> w1100
                  shift-left: w1099 -> [w1113]
                  tunnel: w1101 -> [w1112] mode=indexing
                  n511 = Unbundle(w1112) -> (w1115:dbl)  [unwired: 1 out]
                  n512 = Not Equal To 0?(x=w1115) -> (x != 0?=w1114:bool)
                  n513 = case shown="True" w1114 {
                    tunnel: w1113 -> [w1116 w1119]
                    tunnel: w1112 -> [_ w1118]
                    tunnel: [w1116 w1117] -> w1111
                    frame False {
                    }
                    frame True {
                      n514 = Build Array (concatenate)(w1119, w1118) -> (w1117:cluster{dbl, "GUIdevice 8":string}[])
                    }
                  }
                }
                n515 = for {
                  shift-right: [w1102] -> w1097
                  shift-left: w1099 -> [w1104]
                  tunnel: w1098 -> [w1103] mode=indexing
                  n516 = Unbundle(w1103) -> (w1106:dbl)  [unwired: 1 out]
                  n517 = Not Equal To 0?(x=w1106) -> (x != 0?=w1105:bool)
                  n518 = case shown="True" w1105 {
                    tunnel: w1104 -> [w1107 w1110]
                    tunnel: w1103 -> [_ w1109]
                    tunnel: [w1107 w1108] -> w1102
                    frame False {
                    }
                    frame True {
                      n519 = Build Array (concatenate)(w1110, w1109) -> (w1108:cluster{dbl, "GUIdevice 8":string}[])
                    }
                  }
                }
              }
            }
            n520 = call <vilib>:"Add State(s) to Queue__jki_lib_state_machine.vi"("State(s) in (\"\")"=w1039) -> ("States Out"=w1038:string)  [unwired: 14 in]
            n521 = Bundle By Name(cluster=w1020, "speedmode X"=w1022, "speedmode Y"=w1021) -> (w1019:T36)
            n522 = Index Array(array=w1035) -> (element=w1040:cluster{dbl, "GUIdevice 8":string})  [unwired: 1 in]
            n523 = Index Array(array=w1036) -> (element=w1041:cluster{dbl, "GUIdevice 8":string})  [unwired: 1 in]
            n524 = Empty Array?(array=w1035) -> (empty?=w1043:bool)
            n525 = Unbundle(w1041) -> (w1049:dbl)  [unwired: 1 out]
            n526 = Unbundle(w1040) -> (w1045:dbl)  [unwired: 1 out]
            n527 = Unbundle By Name(w1019) -> ("Feedback global"=w1050:bool)
            n528 = Empty Array?(array=w1036) -> (empty?=w1047:bool)
            n529 = property on="autodetect" class="Bool (strict)"("Value"=FALSE ("autodetect")) -> ()  [unwired: 2 in, 2 out]
            n530 = Equal To 0?(x=w1049) -> (x = 0?=w1048:bool)
            n531 = Equal To 0?(x=w1045) -> (x = 0?=w1044:bool)
            n532 = Or(x=w1048, y=w1047) -> (x .or. y?=w1046:bool)
            n533 = Or(x=w1044, y=w1043) -> (x .or. y?=w1042:bool)
            n534 = case shown="True" w1050 {
              tunnel: w1046 -> [_ w1127]
              tunnel: w1036 -> [_ w1126]
              tunnel: w1042 -> [_ w1124]
              tunnel: w1035 -> [_ w1123]
              tunnel: w1038 -> [w1120 w1122]
              tunnel: [w1120 w1121] -> w1051
              frame False {
              }
              frame True {
                n535 = case shown="False" w1127 {
                  tunnel: w1126 -> [w1142 _]
                  tunnel: w1122 -> [w1138 w1143]
                  tunnel: [w1136 w1143] -> w1125
                  frame False {
                    n536 = Index Array(array=w1142) -> (element=w1141:cluster{dbl, "GUIdevice 8":string})  [unwired: 1 in]
                    n537 = Unbundle By Name(w1141) -> ("GUIdevice 8"=w1140:string)
                    n538 = call <vilib>:"Build State String with Arguments__jki_lib_state_machine.vi"("Arguments (\"\")"=w1140, "State"="Move X") -> ("State with Arguments"=w1137:string)  [unwired: 4 in]
                    n539 = call <vilib>:"Add State(s) to Queue__jki_lib_state_machine.vi"("State(s) in (\"\")"=w1138, "State(s) at Back (\"\")"=w1137) -> ("States Out"=w1136:string)  [unwired: 13 in]
                  }
                  frame True {
                  }
                }
                n540 = case shown="False" w1124 {
                  tunnel: w1123 -> [w1134 _]
                  tunnel: w1125 -> [w1130 w1135]
                  tunnel: [w1128 w1135] -> w1121
                  frame False {
                    n541 = Index Array(array=w1134) -> (element=w1133:cluster{dbl, "GUIdevice 8":string})  [unwired: 1 in]
                    n542 = Unbundle By Name(w1133) -> ("GUIdevice 8"=w1132:string)
                    n543 = call <vilib>:"Build State String with Arguments__jki_lib_state_machine.vi"("Arguments (\"\")"=w1132, "State"="Move Y") -> ("State with Arguments"=w1129:string)  [unwired: 4 in]
                    n544 = call <vilib>:"Add State(s) to Queue__jki_lib_state_machine.vi"("State(s) in (\"\")"=w1130, "State(s) at Back (\"\")"=w1129) -> ("States Out"=w1128:string)  [unwired: 13 in]
                  }
                  frame True {
                  }
                }
              }
            }
            n545 = call <vilib>:"Add State(s) to Queue__jki_lib_state_machine.vi"("State(s) in (\"\")"=w1038, "State(s) at Back (\"\")"=w1051) -> ("States Out"=w1053:string)  [unwired: 13 in]
          }
          frame "Move X" {
            # "Your code here.\n(You can make a copy of, or modify, this frame)"
            n546 = Unbundle By Name(w1163) -> ("Offset X"=w1162:dbl[][])
            n547 = call-poly <userlib>:"Filter 1D Array__ogtk.vi"("items to filter"=w1145, "array"=w1167) -> ("filtered item indices"=w1151:i32[])  [unwired: 4 in, 1 out]
            n548 = Unbundle By Name(w1163) -> ("active axis refs 2"=w1166:T11, "move properties"=w1150:T2[])
            n549 = for {
              tunnel: w1151 -> [w1172] mode=indexing
              tunnel: w1150 -> [w1176]
              shift-right: [w1171] -> w1148
              shift-left: i32[] [] ("filtered item indices") -> [w1174]
              n550 = Index Array(array=w1176, index=w1172) -> (element=w1175:T2)
              n551 = Unbundle By Name(w1175) -> ("enable feedback"=w1173:bool)
              n552 = case shown="True" w1173 {
                tunnel: w1174 -> [w1177 w1180]
                tunnel: w1172 -> [_ w1179]
                tunnel: [w1177 w1178] -> w1171
                frame False {
                }
                frame True {
                  n553 = Build Array (concatenate)(w1180, w1179) -> (w1178:i32[])
                }
              }
            }
            n554 = Index Array(array=w1148) -> (element=w1147:i32)  [unwired: 1 in]
            n555 = Index Array(array=w1162, index (row)=w1147) -> (element=w1161:dbl[])  [unwired: 1 in]
            n556 = Reverse 1D Array(array=w1161) -> (reversed array=w1160:dbl[])
            n557 = Index Array(array=w1166, index=w1147) -> (element=w1165:cluster{"Ref X":refnum<vi>, "Ref Y":refnum<vi>})
            n558 = Index Array(array=w1160) -> (element=w1158:dbl)  [unwired: 1 in]
            n559 = Index Array(array=w1150, index=w1147) -> (element=w1164:T2)
            n560 = Unbundle By Name(w1165) -> ("Ref X"=w1154:refnum<vi>, "Ref Y"=w1153:refnum<vi>)
            n561 = call <vilib>:"Build State String with Arguments__jki_lib_state_machine.vi"("Arguments (\"\")"=w1145, "State"="Wait" ("State(s) in Front (\"\")")) -> ("State with Arguments"=w1144:string)  [unwired: 4 in]
            n562 = Unbundle By Name(w1164) -> ("Invert Direction X"=w1155:bool, "Invert Axis"=w1159:bool, "Stepsize"=w1156:dbl, "enable feedback"=w1152:bool)
            n563 = Greater Or Equal To 0?(x=w1158) -> (x >= 0?=w1157:bool)
            n564 = call <vilib>:"Add State(s) to Queue__jki_lib_state_machine.vi"("State(s) in Front (\"\")"=w1144, "State(s) in (\"\")"=w1170) -> ("States Out"=w1169:string)  [unwired: 13 in]
            n565 = case shown="True" w1152 {
              tunnel: w1159 -> [_ w1186]
              tunnel: w1157 -> [_ w1185]
              tunnel: w1156 -> [_ w1184]
              tunnel: w1155 -> [_ w1183]
              tunnel: w1154 -> [_ w1182]
              tunnel: w1153 -> [_ w1181]
              frame False {
              }
              frame True {
                n566 = case shown="False" w1185 {
                  tunnel: w1183 -> [w1194 w1216]
                  tunnel: w1184 -> [w1192 w1214]
                  tunnel: w1186 -> [w1191 w1213]
                  tunnel: w1186 -> [w1190 w1212]
                  tunnel: w1182 -> [w1188 w1210]
                  tunnel: w1181 -> [w1187 w1209]
                  frame True {
                    n567 = case shown="False" w1191 {
                      tunnel: [w1205 w1207] -> w1193
                      tunnel: w1188 -> [w1206 _]
                      tunnel: w1187 -> [_ w1208]
                      frame False {
                        n568 = property class="DigNum (strict)"(reference=w1206) -> ("Value"=w1205:dbl)  [unwired: 1 in, 2 out]
                      }
                      frame True {
                        n569 = property class="DigNum (strict)"(reference=w1208) -> ("Value"=w1207:dbl)  [unwired: 1 in, 2 out]
                      }
                    }
                    n570 = case shown="False" w1194 {
                      tunnel: w1193 -> [w1201 w1204]
                      tunnel: w1192 -> [w1200 w1203]
                      tunnel: [w1199 w1202] -> w1189
                      frame False {
                        n571 = Add(x=w1201, y=w1200) -> (x+y=w1199:dbl)
                      }
                      frame True {
                        n572 = Subtract(x=w1204, y=w1203) -> (x-y=w1202:dbl)
                      }
                    }
                    n573 = case shown="False" w1190 {
                      tunnel: w1189 -> [w1195 w1197]
                      tunnel: w1188 -> [w1196 _]
                      tunnel: w1187 -> [_ w1198]
                      frame False {
                        n574 = property class="DigNum (strict)"(reference=w1196, "Val(Sgnl)"=w1195) -> ()  [unwired: 1 in, 2 out]
                      }
                      frame True {
                        n575 = property class="DigNum (strict)"(reference=w1198, "Val(Sgnl)"=w1197) -> ()  [unwired: 1 in, 2 out]
                      }
                    }
                  }
                  frame False {
                    n576 = case shown="False" w1213 {
                      tunnel: [w1227 w1229] -> w1215
                      tunnel: w1210 -> [w1228 _]
                      tunnel: w1209 -> [_ w1230]
                      frame False {
                        n577 = property class="DigNum (strict)"(reference=w1228) -> ("Value"=w1227:dbl)  [unwired: 1 in, 2 out]
                      }
                      frame True {
                        n578 = property class="DigNum (strict)"(reference=w1230) -> ("Value"=w1229:dbl)  [unwired: 1 in, 2 out]
                      }
                    }
                    n579 = case shown="False" w1216 {
                      tunnel: w1215 -> [w1223 w1226]
                      tunnel: w1214 -> [w1222 w1225]
                      tunnel: [w1221 w1224] -> w1211
                      frame False {
                        n580 = Subtract(x=w1223, y=w1222) -> (x-y=w1221:dbl)
                      }
                      frame True {
                        n581 = Add(x=w1226, y=w1225) -> (x+y=w1224:dbl)
                      }
                    }
                    n582 = case shown="False" w1212 {
                      tunnel: w1211 -> [w1217 w1219]
                      tunnel: w1210 -> [w1218 _]
                      tunnel: w1209 -> [_ w1220]
                      frame False {
                        n583 = property class="DigNum (strict)"(reference=w1218, "Val(Sgnl)"=w1217) -> ()  [unwired: 1 in, 2 out]
                      }
                      frame True {
                        n584 = property class="DigNum (strict)"(reference=w1220, "Val(Sgnl)"=w1219) -> ()  [unwired: 1 in, 2 out]
                      }
                    }
                  }
                }
              }
            }
            "Moving X" <- w1145
          }
          frame "ManMove X" {
            # "Your code here.\n(You can make a copy of, or modify, this frame)"
            n585 = Equal?(x=w1236, y="Right") -> (x = y?=w1237:bool)
            n586 = Unbundle By Name(w1246) -> ("move properties"=w1241:T2[], "active ccd"=w1234:i32, "active man refs"=w1239:cluster{"Ref X":refnum<vi>, "Ref Y":refnum<vi>}, "active cams"=w1235:string[])
            n587 = Index Array(array=w1235, index=w1234) -> (element=w1232:string)
            n588 = Index Array(array=w1241, index=w1234) -> (element=w1247:T2)
            n589 = Unbundle By Name(w1239) -> ("Ref X"=w1243:refnum<vi>, "Ref Y"=w1242:refnum<vi>)
            n590 = Unbundle By Name(w1247) -> ("Invert Direction X"=w1244:bool, "Invert Axis"=w1245:bool)
            n591 = call <vilib>:"Build State String with Arguments__jki_lib_state_machine.vi"("Arguments (\"\")"=w1232, "State"="Wait" ("State(s) in Front (\"\")")) -> ("State with Arguments"=w1231:string)  [unwired: 4 in]
            n592 = call <vilib>:"Add State(s) to Queue__jki_lib_state_machine.vi"("State(s) in Front (\"\")"=w1231, "State(s) in (\"\")"=w1250) -> ("States Out"=w1249:string)  [unwired: 13 in]
            n593 = case shown="False" w1237 {
              tunnel: w1244 -> [w1258 w1280]
              tunnel: "StepSize" -> [w1256 w1278]
              tunnel: w1245 -> [w1255 w1277]
              tunnel: w1245 -> [w1254 w1276]
              tunnel: w1243 -> [w1252 w1274]
              tunnel: w1242 -> [w1251 w1273]
              frame True {
                n594 = case shown="False" w1255 {
                  tunnel: [w1269 w1271] -> w1257
                  tunnel: w1252 -> [w1270 _]
                  tunnel: w1251 -> [_ w1272]
                  frame False {
                    n595 = property class="DigNum (strict)"(reference=w1270) -> ("Value"=w1269:dbl)  [unwired: 1 in, 2 out]
                  }
                  frame True {
                    n596 = property class="DigNum (strict)"(reference=w1272) -> ("Value"=w1271:dbl)  [unwired: 1 in, 2 out]
                  }
                }
                n597 = case shown="False" w1258 {
                  tunnel: w1257 -> [w1265 w1268]
                  tunnel: w1256 -> [w1264 w1267]
                  tunnel: [w1263 w1266] -> w1253
                  frame False {
                    n598 = Add(x=w1265, y=w1264) -> (x+y=w1263:dbl)
                  }
                  frame True {
                    n599 = Subtract(x=w1268, y=w1267) -> (x-y=w1266:dbl)
                  }
                }
                n600 = case shown="False" w1254 {
                  tunnel: w1253 -> [w1259 w1261]
                  tunnel: w1252 -> [w1260 _]
                  tunnel: w1251 -> [_ w1262]
                  frame False {
                    n601 = property class="DigNum (strict)"(reference=w1260, "Val(Sgnl)"=w1259) -> ()  [unwired: 1 in, 2 out]
                  }
                  frame True {
                    n602 = property class="DigNum (strict)"(reference=w1262, "Val(Sgnl)"=w1261) -> ()  [unwired: 1 in, 2 out]
                  }
                }
              }
              frame False {
                n603 = case shown="True" w1277 {
                  tunnel: [w1291 w1293] -> w1279
                  tunnel: w1274 -> [w1292 _]
                  tunnel: w1273 -> [_ w1294]
                  frame False {
                    n604 = property class="DigNum (strict)"(reference=w1292) -> ("Value"=w1291:dbl)  [unwired: 1 in, 2 out]
                  }
                  frame True {
                    n605 = property class="DigNum (strict)"(reference=w1294) -> ("Value"=w1293:dbl)  [unwired: 1 in, 2 out]
                  }
                }
                n606 = case shown="False" w1280 {
                  tunnel: w1279 -> [w1287 w1290]
                  tunnel: w1278 -> [w1286 w1289]
                  tunnel: [w1285 w1288] -> w1275
                  frame False {
                    n607 = Subtract(x=w1287, y=w1286) -> (x-y=w1285:dbl)
                  }
                  frame True {
                    n608 = Add(x=w1290, y=w1289) -> (x+y=w1288:dbl)
                  }
                }
                n609 = case shown="False" w1276 {
                  tunnel: w1275 -> [w1281 w1283]
                  tunnel: w1274 -> [w1282 _]
                  tunnel: w1273 -> [_ w1284]
                  frame False {
                    n610 = property class="DigNum (strict)"(reference=w1282, "Val(Sgnl)"=w1281) -> ()  [unwired: 1 in, 2 out]
                  }
                  frame True {
                    n611 = property class="DigNum (strict)"(reference=w1284, "Val(Sgnl)"=w1283) -> ()  [unwired: 1 in, 2 out]
                  }
                }
              }
            }
          }
          frame "ManMove Y" {
            # "Your code here.\n(You can make a copy of, or modify, this frame)"
            n612 = Equal?(x=w1300, y="Down") -> (x = y?=w1304:bool)
            n613 = Unbundle By Name(w1310) -> ("active cams"=w1299:string[], "move properties"=w1309:T2[], "active ccd"=w1298:i32, "active man refs"=w1308:cluster{"Ref X":refnum<vi>, "Ref Y":refnum<vi>})
            n614 = Index Array(array=w1299, index=w1298) -> (element=w1296:string)
            n615 = property on="StepSize" class="DigNum (strict)"() -> ("Value"=w1301:dbl)  [unwired: 2 in, 2 out]
            n616 = Index Array(array=w1309, index=w1298) -> (element=w1311:T2)
            n617 = Unbundle By Name(w1308) -> ("Ref Y"=w1303:refnum<vi>, "Ref X"=w1302:refnum<vi>)
            n618 = Unbundle By Name(w1311) -> ("Invert Direction Y"=w1306:bool, "Invert Axis"=w1305:bool)
            n619 = call <vilib>:"Build State String with Arguments__jki_lib_state_machine.vi"("Arguments (\"\")"=w1296, "State"="Wait" ("State(s) in Front (\"\")")) -> ("State with Arguments"=w1295:string)  [unwired: 4 in]
            n620 = call <vilib>:"Add State(s) to Queue__jki_lib_state_machine.vi"("State(s) in Front (\"\")"=w1295, "State(s) in (\"\")"=w1314) -> ("States Out"=w1313:string)  [unwired: 13 in]
            n621 = case shown="True" w1304 {
              tunnel: w1306 -> [w1322 w1344]
              tunnel: w1301 -> [w1320 w1342]
              tunnel: w1305 -> [w1319 w1341]
              tunnel: w1305 -> [w1318 w1340]
              tunnel: w1303 -> [w1316 w1338]
              tunnel: w1302 -> [w1315 w1337]
              frame True {
                n622 = case shown="False" w1319 {
                  tunnel: [w1333 w1335] -> w1321
                  tunnel: w1316 -> [w1334 _]
                  tunnel: w1315 -> [_ w1336]
                  frame False {
                    n623 = property class="DigNum (strict)"(reference=w1334) -> ("Value"=w1333:dbl)  [unwired: 1 in, 2 out]
                  }
                  frame True {
                    n624 = property class="DigNum (strict)"(reference=w1336) -> ("Value"=w1335:dbl)  [unwired: 1 in, 2 out]
                  }
                }
                n625 = case shown="False" w1322 {
                  tunnel: w1321 -> [w1329 w1332]
                  tunnel: w1320 -> [w1328 w1331]
                  tunnel: [w1327 w1330] -> w1317
                  frame False {
                    n626 = Add(x=w1329, y=w1328) -> (x+y=w1327:dbl)
                  }
                  frame True {
                    n627 = Subtract(x=w1332, y=w1331) -> (x-y=w1330:dbl)
                  }
                }
                n628 = case shown="False" w1318 {
                  tunnel: w1317 -> [w1323 w1325]
                  tunnel: w1316 -> [w1324 _]
                  tunnel: w1315 -> [_ w1326]
                  frame False {
                    n629 = property class="DigNum (strict)"(reference=w1324, "Val(Sgnl)"=w1323) -> ()  [unwired: 1 in, 2 out]
                  }
                  frame True {
                    n630 = property class="DigNum (strict)"(reference=w1326, "Val(Sgnl)"=w1325) -> ()  [unwired: 1 in, 2 out]
                  }
                }
              }
              frame False {
                n631 = case shown="False" w1341 {
                  tunnel: [w1355 w1357] -> w1343
                  tunnel: w1338 -> [w1356 _]
                  tunnel: w1337 -> [_ w1358]
                  frame False {
                    n632 = property class="DigNum (strict)"(reference=w1356) -> ("Value"=w1355:dbl)  [unwired: 1 in, 2 out]
                  }
                  frame True {
                    n633 = property class="DigNum (strict)"(reference=w1358) -> ("Value"=w1357:dbl)  [unwired: 1 in, 2 out]
                  }
                }
                n634 = case shown="False" w1344 {
                  tunnel: w1343 -> [w1351 w1354]
                  tunnel: w1342 -> [w1350 w1353]
                  tunnel: [w1349 w1352] -> w1339
                  frame False {
                    n635 = Subtract(x=w1351, y=w1350) -> (x-y=w1349:dbl)
                  }
                  frame True {
                    n636 = Add(x=w1354, y=w1353) -> (x+y=w1352:dbl)
                  }
                }
                n637 = case shown="False" w1340 {
                  tunnel: w1339 -> [w1345 w1347]
                  tunnel: w1338 -> [w1346 _]
                  tunnel: w1337 -> [_ w1348]
                  frame False {
                    n638 = property class="DigNum (strict)"(reference=w1346, "Val(Sgnl)"=w1345) -> ()  [unwired: 1 in, 2 out]
                  }
                  frame True {
                    n639 = property class="DigNum (strict)"(reference=w1348, "Val(Sgnl)"=w1347) -> ()  [unwired: 1 in, 2 out]
                  }
                }
              }
            }
          }
          frame "Move Y" {
            # "Your code here.\n(You can make a copy of, or modify, this frame)"
            n640 = Unbundle By Name(w1378) -> ("Offset Y"=w1377:dbl[][])
            n641 = call-poly <userlib>:"Filter 1D Array__ogtk.vi"("items to filter"=w1360, "array"=w1382) -> ("filtered item indices"=w1366:i32[])  [unwired: 4 in, 1 out]
            n642 = Unbundle By Name(w1378) -> ("active axis refs 2"=w1381:T11, "move properties"=w1364:T2[])
            n643 = for {
              tunnel: w1366 -> [w1387] mode=indexing
              tunnel: w1364 -> [w1391]
              shift-right: [w1386] -> w1365
              shift-left: i32[] [] ("filtered item indices") -> [w1389]
              n644 = Index Array(array=w1391, index=w1387) -> (element=w1390:T2)
              n645 = Unbundle By Name(w1390) -> ("enable feedback"=w1388:bool)
              n646 = case shown="True" w1388 {
                tunnel: w1389 -> [w1392 w1395]
                tunnel: w1387 -> [_ w1394]
                tunnel: [w1392 w1393] -> w1386
                frame False {
                }
                frame True {
                  n647 = Build Array (concatenate)(w1395, w1394) -> (w1393:i32[])
                }
              }
            }
            n648 = Index Array(array=w1365) -> (element=w1362:i32)  [unwired: 1 in]
            n649 = Index Array(array=w1377, index (row)=w1362) -> (element=w1376:dbl[])  [unwired: 1 in]
            n650 = Reverse 1D Array(array=w1376) -> (reversed array=w1375:dbl[])
            n651 = Index Array(array=w1381, index=w1362) -> (element=w1380:cluster{"Ref X":refnum<vi>, "Ref Y":refnum<vi>})
            n652 = Index Array(array=w1375) -> (element=w1373:dbl)  [unwired: 1 in]
            n653 = Index Array(array=w1364, index=w1362) -> (element=w1379:T2)
            n654 = Unbundle By Name(w1380) -> ("Ref Y"=w1369:refnum<vi>, "Ref X"=w1368:refnum<vi>)
            n655 = Unbundle By Name(w1379) -> ("Invert Direction Y"=w1370:bool, "Invert Axis"=w1374:bool, "Stepsize"=w1371:dbl, "enable feedback"=w1367:bool)
            n656 = Greater Or Equal To 0?(x=w1373) -> (x >= 0?=w1372:bool)
            n657 = call <vilib>:"Build State String with Arguments__jki_lib_state_machine.vi"("Arguments (\"\")"=w1360, "State"="Wait" ("State(s) in Front (\"\")")) -> ("State with Arguments"=w1359:string)  [unwired: 4 in]
            n658 = call <vilib>:"Add State(s) to Queue__jki_lib_state_machine.vi"("State(s) in Front (\"\")"=w1359, "State(s) in (\"\")"=w1385) -> ("States Out"=w1384:string)  [unwired: 13 in]
            n659 = case shown="True" w1367 {
              tunnel: w1374 -> [_ w1401]
              tunnel: w1372 -> [_ w1400]
              tunnel: w1371 -> [_ w1399]
              tunnel: w1370 -> [_ w1398]
              tunnel: w1369 -> [_ w1397]
              tunnel: w1368 -> [_ w1396]
              frame False {
              }
              frame True {
                n660 = case shown="True" w1400 {
                  tunnel: w1398 -> [w1409 w1431]
                  tunnel: w1399 -> [w1407 w1429]
                  tunnel: w1401 -> [w1406 w1428]
                  tunnel: w1401 -> [w1405 w1427]
                  tunnel: w1397 -> [w1403 w1425]
                  tunnel: w1396 -> [w1402 w1424]
                  frame True {
                    n661 = case shown="False" w1406 {
                      tunnel: [w1420 w1422] -> w1408
                      tunnel: w1403 -> [w1421 _]
                      tunnel: w1402 -> [_ w1423]
                      frame False {
                        n662 = property class="DigNum (strict)"(reference=w1421) -> ("Value"=w1420:dbl)  [unwired: 1 in, 2 out]
                      }
                      frame True {
                        n663 = property class="DigNum (strict)"(reference=w1423) -> ("Value"=w1422:dbl)  [unwired: 1 in, 2 out]
                      }
                    }
                    n664 = case shown="False" w1409 {
                      tunnel: w1408 -> [w1416 w1419]
                      tunnel: w1407 -> [w1415 w1418]
                      tunnel: [w1414 w1417] -> w1404
                      frame False {
                        n665 = Add(x=w1416, y=w1415) -> (x+y=w1414:dbl)
                      }
                      frame True {
                        n666 = Subtract(x=w1419, y=w1418) -> (x-y=w1417:dbl)
                      }
                    }
                    n667 = case shown="False" w1405 {
                      tunnel: w1404 -> [w1410 w1412]
                      tunnel: w1403 -> [w1411 _]
                      tunnel: w1402 -> [_ w1413]
                      frame False {
                        n668 = property class="DigNum (strict)"(reference=w1411, "Val(Sgnl)"=w1410) -> ()  [unwired: 1 in, 2 out]
                      }
                      frame True {
                        n669 = property class="DigNum (strict)"(reference=w1413, "Val(Sgnl)"=w1412) -> ()  [unwired: 1 in, 2 out]
                      }
                    }
                  }
                  frame False {
                    n670 = case shown="False" w1428 {
                      tunnel: [w1442 w1444] -> w1430
                      tunnel: w1425 -> [w1443 _]
                      tunnel: w1424 -> [_ w1445]
                      frame False {
                        n671 = property class="DigNum (strict)"(reference=w1443) -> ("Value"=w1442:dbl)  [unwired: 1 in, 2 out]
                      }
                      frame True {
                        n672 = property class="DigNum (strict)"(reference=w1445) -> ("Value"=w1444:dbl)  [unwired: 1 in, 2 out]
                      }
                    }
                    n673 = case shown="False" w1431 {
                      tunnel: w1430 -> [w1438 w1441]
                      tunnel: w1429 -> [w1437 w1440]
                      tunnel: [w1436 w1439] -> w1426
                      frame False {
                        n674 = Subtract(x=w1438, y=w1437) -> (x-y=w1436:dbl)
                      }
                      frame True {
                        n675 = Add(x=w1441, y=w1440) -> (x+y=w1439:dbl)
                      }
                    }
                    n676 = case shown="False" w1427 {
                      tunnel: w1426 -> [w1432 w1434]
                      tunnel: w1425 -> [w1433 _]
                      tunnel: w1424 -> [_ w1435]
                      frame False {
                        n677 = property class="DigNum (strict)"(reference=w1433, "Val(Sgnl)"=w1432) -> ()  [unwired: 1 in, 2 out]
                      }
                      frame True {
                        n678 = property class="DigNum (strict)"(reference=w1435, "Val(Sgnl)"=w1434) -> ()  [unwired: 1 in, 2 out]
                      }
                    }
                  }
                }
              }
            }
            "Moving Y" <- w1360
          }
          frame "Wait" {
            # "Your code here.\n(You can make a copy of, or modify, this frame)"
            n679 = flat-sequence {
              tunnel: T19."Disabled and Grayed Out" ("Disabled") -> [w1462]
              tunnel: w1452 -> [w1471]
              tunnel: w1451 -> [w1470]
              tunnel: [w1469] -> w1450
              tunnel: w1449 -> [w1468]
              tunnel: w1448 -> [w1467]
              tunnel: T19."Enabled" ("Disabled") -> [w1481]
              frame #0 {
                n680 = property on="Right" class="Bool (strict)"("DisabledEnum"=w1462) -> ()  [unwired: 2 in, 2 out]
                n681 = property on="Up" class="Bool (strict)"("DisabledEnum"=w1462) -> ()  [unwired: 2 in, 2 out]
                n682 = property on="Left" class="Bool (strict)"("DisabledEnum"=w1462) -> ()  [unwired: 2 in, 2 out]
                n683 = property on="Down" class="Bool (strict)"("DisabledEnum"=w1462) -> ()  [unwired: 2 in, 2 out]
                n684 = property on="StepSize" class="DigNum (strict)"("DisabledEnum"=w1462) -> ()  [unwired: 2 in, 2 out]
              }
              frame #1 {
                n685 = Wait (ms)(milliseconds to wait=u32 400) -> ()  [unwired: 1 out]
              }
              frame #2 {
                n686 = property on="Moving Y" class="Str"("Value"="") -> ()  [unwired: 2 in, 2 out]
                n687 = property on="Moving X" class="Str"("Value"="") -> ()  [unwired: 2 in, 2 out]
              }
              frame #3 {
                n688 = Equal?(x=w1467, y=w1468) -> (x = y?=w1466:bool)
                n689 = case shown="True" w1466 {
                  tunnel: w1471 -> [_ w1478]
                  tunnel: w1470 -> [w1472 w1475]
                  tunnel: [w1472 w1473] -> w1469
                  frame False {
                  }
                  frame True {
                    n690 = Unbundle By Name(w1478) -> ("Ref X"=w1477:refnum<vi>, "Ref Y"=w1476:refnum<vi>)
                    n691 = property class="DigNum (strict)"(reference=w1477, error in=w1475) -> (error out=w1474:errorcluster, "Value"=w1480:dbl)  [unwired: 1 out]
                    n692 = property class="DigNum (strict)"(reference=w1476, error in=w1474) -> (error out=w1473:errorcluster, "Value"=w1479:dbl)  [unwired: 1 out]
                    n693 = property on="Position 1" class="DigNum (strict)"("Value"=w1480) -> ()  [unwired: 2 in, 2 out]
                    n694 = property on="Position 2" class="DigNum (strict)"("Value"=w1479) -> ()  [unwired: 2 in, 2 out]
                  }
                }
              }
              frame #4 {
                n695 = property on="Right" class="Bool (strict)"("DisabledEnum"=w1481) -> ()  [unwired: 2 in, 2 out]
                n696 = property on="Up" class="Bool (strict)"("DisabledEnum"=w1481) -> ()  [unwired: 2 in, 2 out]
                n697 = property on="Left" class="Bool (strict)"("DisabledEnum"=w1481) -> ()  [unwired: 2 in, 2 out]
                n698 = property on="Down" class="Bool (strict)"("DisabledEnum"=w1481) -> ()  [unwired: 2 in, 2 out]
                n699 = property on="StepSize" class="DigNum (strict)"("DisabledEnum"=w1481) -> ()  [unwired: 2 in, 2 out]
              }
            }
            n700 = call-poly <userlib>:"Filter 1D Array__ogtk.vi"("items to filter"=w1455, "array"=w1456) -> ("filtered item indices"=w1454:i32[])  [unwired: 4 in, 1 out]
            n701 = Index Array(array=w1454) -> (element=w1449:i32)  [unwired: 1 in]
            n702 = Unbundle By Name(w1457) -> ("active axis refs 2"=w1453:T11, "active ccd"=w1448:i32)
            n703 = Index Array(array=w1453, index=w1449) -> (element=w1452:cluster{"Ref X":refnum<vi>, "Ref Y":refnum<vi>})
            n704 = call <vilib>:"Add State(s) to Queue__jki_lib_state_machine.vi"("State(s) in (\"\")"=w1461) -> ("States Out"=w1460:string)  [unwired: 14 in]
            n705 = local read "Mean Centroid X"() -> (w1458:dbl[][])
            n706 = Bundle By Name(cluster=w1457, "Mean Centroid X"=w1458, "Mean Centroid Y"=w1458) -> (w1459:T36)
          }
          frame "---------------Statistics--------------" {
            # "Template Separator\n(You can make a copy of, or modify, this frame)"
            n707 = call <vilib>:"Add State(s) to Queue__jki_lib_state_machine.vi"("State(s) in (\"\")"=w1485) -> ("States Out"=w1484:string)  [unwired: 14 in]
          }
          frame "Save Stats" {
            # "Your code here.\n(You can make a copy of, or modify, this frame)"
            n708 = property on="CCD 1" class="XYGraph (strict)"() -> ("Value"=w1495:cluster{timestamp[], dbl[]}[])  [unwired: 2 in, 2 out]
            n709 = property on="CCD 2" class="XYGraph (strict)"() -> ("Value"=w1494:cluster{timestamp[], dbl[]}[])  [unwired: 2 in, 2 out]
            n710 = property on="CCD 3" class="XYGraph (strict)"() -> ("Value"=w1493:cluster{timestamp[], dbl[]}[])  [unwired: 2 in, 2 out]
            n711 = property on="CCD 4" class="XYGraph (strict)"() -> ("Value"=w1492:cluster{timestamp[], dbl[]}[])  [unwired: 2 in, 2 out]
            n712 = property on="CCD 5" class="XYGraph (strict)"() -> ("Value"=w1491:cluster{timestamp[], dbl[]}[])  [unwired: 2 in, 2 out]
            n713 = property on="CCD 6" class="XYGraph (strict)"() -> ("Value"=w1490:cluster{timestamp[], dbl[]}[])  [unwired: 2 in, 2 out]
            n714 = property on="CCD 7" class="XYGraph (strict)"() -> ("Value"=w1489:cluster{timestamp[], dbl[]}[])  [unwired: 2 in, 2 out]
            n715 = property on="CCD 8" class="XYGraph (strict)"() -> ("Value"=w1488:cluster{timestamp[], dbl[]}[])  [unwired: 2 in, 2 out]
            n716 = Build Array(w1495, w1494, w1493, w1492, w1491, w1490, w1489, w1488) -> (w1487:cluster{timestamp[], dbl[]}[][])
            n717 = for {
              tunnel: w1487 -> [w1503] mode=indexing
              tunnel: w1486 -> [w1502] mode=indexing
              n718 = Empty String/Path?(string/path=w1502) -> (empty?=w1501:bool)
              n719 = case shown="False" w1501 {
                tunnel: w1503 -> [w1509 _]
                tunnel: w1502 -> [w1507 _]
                frame False {
                  n720 = Index Array(array=w1509, index #1=0 ("index"), index #2=1 ("index"), index #3=2 ("index"), index #4=3 ("index")) -> (element #1=w1544:cluster{timestamp[], dbl[]}, element #2=w1538:cluster{timestamp[], dbl[]}, element #3=w1537:cluster{timestamp[], dbl[]}, element #4=w1536:cluster{timestamp[], dbl[]})  [unwired: 1 in, 1 out]
                  n721 = Concatenate Strings(w1507, ".dat" ("string")) -> (w1505:string)
                  n722 = Unbundle(w1544) -> (w1543:timestamp[], w1521:dbl[])
                  n723 = Unbundle(w1538) -> (w1512:dbl[])  [unwired: 1 out]
                  n724 = Unbundle(w1537) -> (w1511:dbl[])  [unwired: 1 out]
                  n725 = Unbundle(w1536) -> (w1510:dbl[])  [unwired: 1 out]
                  n726 = Build Path(base path="save path", name or relative path=w1505) -> (appended path=w1504:path)
                  n727 = for {
                    tunnel: w1543 -> [w1546] mode=indexing
                    tunnel: [w1545] -> w1519 mode=indexing
                    n728 = Format Date/Time String(time format string (%c)="%Y%m%d%H%M%S", seconds (now)=w1546) -> (date/time string=w1545:string)  [unwired: 1 in]
                  }
                  n729 = Array Size(array=w1521) -> (size(s)=w1522:i32)
                  n730 = Number To Fractional String(number=w1521) -> (F-format string=w1518:string[])  [unwired: 3 in]
                  n731 = Number To Fractional String(number=w1512) -> (F-format string=w1515:string[])  [unwired: 3 in]
                  n732 = Number To Fractional String(number=w1511) -> (F-format string=w1514:string[])  [unwired: 3 in]
                  n733 = Number To Fractional String(number=w1510) -> (F-format string=w1513:string[])  [unwired: 3 in]
                  n734 = Initialize Array("", w1522, 5 ("dimension size")) -> (w1520:string[][])
                  n735 = Insert Into Array(array=w1520, index (col)=0 ("disabled index (col)"), new element=w1519) -> (w1530:string[][])  [unwired: 1 in]
                  n736 = Insert Into Array(array=w1530, index (col)=1 ("disabled index (col)"), new element=w1518) -> (w1529:string[][])  [unwired: 1 in]
                  n737 = Insert Into Array(array=w1529, index (col)=2 ("disabled index (col)"), new element=w1515) -> (w1533:string[][])  [unwired: 1 in]
                  n738 = Insert Into Array(array=w1533, index (col)=3 ("disabled index (col)"), new element=w1514) -> (w1534:string[][])  [unwired: 1 in]
                  n739 = Insert Into Array(array=w1534, index (col)=4 ("disabled index (col)"), new element=w1513) -> (w1535:string[][])  [unwired: 1 in]
                  n740 = Insert Into Array(array=w1535, index (row)=0, new element=string[] ["time", "Centroid X", "Centroid Y", "Motor Axis 1", "Motor Axis 2"] ("new element/subarray 2")) -> (w1517:string[][])  [unwired: 1 in]
                  n741 = call-poly <vilib>:"Write To Spreadsheet File.vi"("2D data"=w1517, "file path (dialog if empty)"=w1504) -> ()  [unwired: 6 in, 1 out]
                }
                frame True {
                }
              }
            }
            n742 = call <vilib>:"Add State(s) to Queue__jki_lib_state_machine.vi"("State(s) in (\"\")"=w1500) -> ("States Out"=w1499:string)  [unwired: 14 in]
            n743 = property on="Save Stats" class="Bool (strict)"("Value"=FALSE ("Save Stats")) -> ()  [unwired: 2 in, 2 out]
          }
          frame "tdms" {
            w1571 = 21600.0 ("new tdms")
            # "Your code here.\n(You can make a copy of, or modify, this frame)"
            n744 = Unbundle By Name(w1563) -> ("active cams"=w1564:string[], "Data Value Reference out"=w1581:refnum<k34>, "Offset X"=w1580:dbl[][], "Offset Y"=w1579:dbl[][], "active axis refs 2"=w1578:T11)
            n745 = for {
              tunnel: w1580 -> [w1626]
              tunnel: w1579 -> [w1625]
              tunnel: w1564 -> [w1589] mode=indexing
              tunnel: w1581 -> [w1590]
              tunnel: w1578 -> [w1611]
              tunnel: w1577 -> [w1595]
              tunnel: [w1593] -> w1576
              i -> [w1612]
              n746 = Index Array(array=w1626, index (row)=w1612) -> (element=w1624:dbl[])  [unwired: 1 in]
              n747 = Index Array(array=w1625, index (row)=w1612) -> (element=w1623:dbl[])  [unwired: 1 in]
              n748 = Index Array(array=w1611, index=w1612) -> (element=w1610:cluster{"Ref X":refnum<vi>, "Ref Y":refnum<vi>})
              n749 = Reverse 1D Array(array=w1623) -> (reversed array=w1621:dbl[])
              n750 = Reverse 1D Array(array=w1624) -> (reversed array=w1622:dbl[])
              n751 = Unbundle By Name(w1610) -> ("Ref X"=w1609:refnum<vi>, "Ref Y"=w1608:refnum<vi>)
              n752 = Index Array(array=w1622) -> (element=w1620:dbl)  [unwired: 1 in]
              n753 = Index Array(array=w1621) -> (element=w1619:dbl)  [unwired: 1 in]
              n754 = property class="DigNum (strict)"(reference=w1609, error in=w1595) -> (error out=w1594:errorcluster, "Value"=w1603:dbl)  [unwired: 1 out]
              n755 = Build Array(w1620) -> (w1592:dbl[])
              n756 = Build Array(w1619) -> (w1614:dbl[])
              n757 = Get Date/Time In Seconds() -> (seconds since 1Jan1904=w1591:timestamp)
              n758 = Build Array(w1591) -> (w1587:timestamp[])
              n759 = property class="DigNum (strict)"(reference=w1608, error in=w1594) -> (error out=w1585:errorcluster, "Value"=w1597:dbl)  [unwired: 1 out]
              n760 = Build Array(w1603) -> (w1602:dbl[])
              n761 = TDMS Write(0:w1590, 5:w1589, 7:"time", 9:w1587, 11:w1585) -> (4:w1586:refnum<k34>, 15:w1584:errorcluster)  [unwired: 1 in, 2 out]
              n762 = Build Array(w1597) -> (w1596:dbl[])
              n763 = TDMS Write(0:w1586, 5:w1589, 7:"centroid X", 9:w1592, 11:w1584) -> (4:w1617:refnum<k34>, 6:w1616:string, 15:w1615:errorcluster)  [unwired: 1 in, 1 out]
              n764 = TDMS Write(0:w1617, 5:w1616, 7:"centroid Y", 9:w1614, 11:w1615) -> (4:w1606:refnum<k34>, 6:w1605:string, 15:w1607:errorcluster)  [unwired: 1 in, 1 out]
              n765 = TDMS Write(0:w1606, 5:w1605, 7:"Motor Axis 1", 9:w1602, 11:w1607) -> (4:w1601:refnum<k34>, 6:w1600:string, 15:w1598:errorcluster)  [unwired: 1 in, 1 out]
              n766 = TDMS Write(0:w1601, 5:w1600, 7:"Motor Axis 2", 9:w1596, 11:w1598) -> (15:w1593:errorcluster)  [unwired: 1 in, 3 out]
            }
            n767 = property on="millisecond timer value" class="DigNum (strict)"() -> ("Value"=w1550:u32)  [unwired: 2 in, 2 out]
            n768 = Tick Count (ms)() -> (millisecond timer value=w1549:u32)
            n769 = Subtract(x=w1549, y=w1550) -> (x-y=w1554:u32)
            n770 = Divide(x=w1554, y=u32 1000) -> (x/y=w1552:dbl)
            n771 = Unbundle By Name(w1563) -> ("img to avg"=w1551:i32)
            n772 = Multiply(x=5.0 ("new tdms"), y=w1551) -> (x*y=w1557:dbl)
            n773 = Quotient & Remainder(x=w1552, y=w1557) -> (x-y*floor(x/y)=w1556:dbl)  [unwired: 1 out]
            "x-y*floor(x/y)" <- w1556
            n774 = Subtract(x=w1557, y=2.0) -> (x-y=w1559:dbl)
            n775 = Greater?(x=w1556, y=w1559) -> (0:w1560:bool)
            n776 = Select(t="Device Ini", s=w1560, f="") -> (s? t:f=w1548:string)
            n777 = Subtract(x=w1549, y=w1550) -> (x-y=w1566:u32)
            n778 = Divide(x=w1566, y=u32 1000) -> (x/y=w1568:dbl)
            n779 = Quotient & Remainder(x=w1568, y=w1571) -> (x-y*floor(x/y)=w1569:dbl)  [unwired: 1 out]
            n780 = Subtract(x=w1571, y=20.0) -> (x-y=w1573:dbl)
            n781 = Greater?(x=w1569, y=w1573) -> (0:w1570:bool)
            n782 = Select(t="newtdms", s=w1570, f="") -> (s? t:f=w1565:string)
            n783 = call <vilib>:"Add State(s) to Queue__jki_lib_state_machine.vi"("State(s) in Front (\"\")"=w1548, "State(s) in (\"\")"=w1583, "State(s) at Back (\"\")"=w1565) -> ("States Out"=w1582:string)  [unwired: 12 in]
          }
          frame "Reset History" {
            # "Your code here.\n(You can make a copy of, or modify, this frame)"
            n784 = for {
              N: 1 -> [_]
              shift-right: [w1636] -> w1628
              shift-left: timestamp[][] [] ("Time") -> [w1638]
              n785 = for {
                N: 12 -> [_]
                tunnel: w1638 -> [w1641] mode=indexing
                tunnel: [w1639] -> w1636 mode=indexing
                n786 = Get Date/Time In Seconds() -> (seconds since 1Jan1904=w1640:timestamp)
                n787 = Build Array (concatenate)(w1641, w1640) -> (w1639:timestamp[])
              }
            }
            n788 = local read "Offset X"() -> (w1627:dbl[][])
            n789 = Bundle By Name(cluster=w1632, "Offset X"=w1627, "Offset Y"=w1627, "Time"=w1628, "Motor X"=w1627) -> (w1631:T36)
            n790 = call <vilib>:"Add State(s) to Queue__jki_lib_state_machine.vi"("State(s) in (\"\")"=w1635) -> ("States Out"=w1634:string)  [unwired: 14 in]
          }
          frame "New Category: 2" {
            # "Your code here.\n(You can make a copy of, or modify, this frame)"
            n791 = call <vilib>:"Add State(s) to Queue__jki_lib_state_machine.vi"("State(s) in (\"\")"=w1645) -> ("States Out"=w1644:string)  [unwired: 14 in]
          }
          frame "stats" {
            # "Your code here.\n(You can make a copy of, or modify, this frame)"
            n792 = Unbundle By Name(w1653) -> ("Offset X"=w1651:dbl[][], "Offset Y"=w1650:dbl[][], "Time"=w1649:timestamp[][], "Motor X"=w1648:dbl[][], "Motor Y"=w1647:dbl[][])
            n793 = for {
              tunnel: w1652 -> [_] mode=indexing
              tunnel: w1651 -> [w1690]
              tunnel: w1650 -> [w1689]
              tunnel: w1649 -> [w1688]
              tunnel: w1648 -> [w1684]
              tunnel: w1647 -> [w1683]
              tunnel: [w1692] -> w1646 mode=indexing
              i -> [w1691]
              n794 = Index Array(array=w1689, index (row)=w1691) -> (element=w1685:dbl[])  [unwired: 1 in]
              n795 = Index Array(array=w1684, index (row)=w1691) -> (element=w1682:dbl[])  [unwired: 1 in]
              n796 = Index Array(array=w1683, index (row)=w1691) -> (element=w1681:dbl[])  [unwired: 1 in]
              n797 = Index Array(array=w1690, index (row)=w1691) -> (element=w1686:dbl[])  [unwired: 1 in]
              n798 = Index Array(array=w1688, index (row)=w1691) -> (element=w1687:timestamp[])  [unwired: 1 in]
              n799 = Bundle("Time"=w1687, "Motor X"=w1682) -> (w1695:cluster{"Time":timestamp[], "Motor X":dbl[]})  [unwired: 1 in]
              n800 = Bundle("Time"=w1687, "Motor Y"=w1681) -> (w1696:cluster{"Time":timestamp[], "Motor Y":dbl[]})  [unwired: 1 in]
              n801 = Bundle("Time"=w1687, "Offset X"=w1686) -> (w1694:cluster{"Time":timestamp[], "Offset X":dbl[]})  [unwired: 1 in]
              n802 = Bundle("Time"=w1687, "Offset Y"=w1685) -> (w1693:cluster{"Time":timestamp[], "Offset Y":dbl[]})  [unwired: 1 in]
              n803 = Build Array(w1693, w1694, w1695, w1696) -> (w1692:cluster{"Time":timestamp[], "Motor Y":dbl[]}[])
            }
            n804 = call <vilib>:"Add State(s) to Queue__jki_lib_state_machine.vi"("State(s) in (\"\")"=w1680) -> ("States Out"=w1679:string)  [unwired: 14 in]
            n805 = Index Array(array=w1646, index (row) #1=0 ("index (row)"), index (row) #2=1 ("index (row)"), index (row) #3=2 ("index (row)"), index (row) #4=3 ("index (row)"), index (row) #5=4 ("index (row)"), index (row) #6=5 ("index (row)"), index (row) #7=6 ("index (row)"), index (row) #8=7 ("index (row)"), index (row) #9=8 ("index (row)"), index (row) #10=9 ("index (row)"), index (row) #11=10 ("index (row)"), index (row) #12=11 ("index (row)")) -> (element #1=→"CCD 1":cluster{"Time":timestamp[], "Motor Y":dbl[]}[], element #2=→"CCD 2":cluster{"Time":timestamp[], "Motor Y":dbl[]}[], element #3=→"CCD 3":cluster{"Time":timestamp[], "Motor Y":dbl[]}[], element #4=→"CCD 4":cluster{"Time":timestamp[], "Motor Y":dbl[]}[], element #5=→"CCD 5":cluster{"Time":timestamp[], "Motor Y":dbl[]}[], element #6=→"CCD 6":cluster{"Time":timestamp[], "Motor Y":dbl[]}[], element #7=→"CCD 7":cluster{"Time":timestamp[], "Motor Y":dbl[]}[], element #8=→"CCD 8":cluster{"Time":timestamp[], "Motor Y":dbl[]}[], element #9=→"CCD 9":cluster{"Time":timestamp[], "Motor Y":dbl[]}[], element #10=→"CCD 10":cluster{"Time":timestamp[], "Motor Y":dbl[]}[], element #11=→"CCD 11":cluster{"Time":timestamp[], "Motor Y":dbl[]}[], element #12=→"CCD 12":cluster{"Time":timestamp[], "Motor Y":dbl[]}[])  [unwired: 12 in]
          }
          frame "newtdms" {
            # "Your code here.\n(You can make a copy of, or modify, this frame)"
            n806 = Unbundle By Name(w1707) -> ("Data Value Reference out"=w1708:refnum<k34>, "active cams"=w1700:string[])
            n807 = TDMS Close(8:w1701, 11:w1708) -> (0:w1698:errorcluster)  [unwired: 1 out]
            n808 = call <vilib>:"Clear Errors.vi"("error in (no error)"=w1698) -> ("error out"=w1697:errorcluster)  [unwired: 6 in]
            n809 = property on="new tdms" class="Bool (strict)"("Value"=FALSE ("new tdms")) -> ()  [unwired: 2 in, 2 out]
            n810 = Get Date/Time In Seconds() -> (seconds since 1Jan1904=w1718:timestamp)
            n811 = Format Date/Time String(time format string (%c)="%Y%m%d%H%M", seconds (now)=w1718) -> (date/time string=w1709:string)  [unwired: 1 in]
            n812 = Concatenate Strings(w1709, "Beampointing_TRA.tdms" ("string")) -> (w1715:string)
            n813 = String To Path(string=w1715) -> (path=w1716:path)
            n814 = Build Path(base path=path "c:/BP_DATA", name or relative path=w1716) -> (appended path=w1710:path)
            n815 = TDMS Open(6:FALSE ("disable buffering (T)"), 7:enum16{"1.0", "2.0"}."2.0" ("file format version (2.0)"), 8:w1697, 10:T16."create or replace" ("operation"), 11:w1710) -> (0:w1704:errorcluster, 3:w1703:refnum<k34>)  [unwired: 2 in]
            n816 = call <vilib>:"Add State(s) to Queue__jki_lib_state_machine.vi"("State(s) in (\"\")"=w1721) -> ("States Out"=w1720:string)  [unwired: 14 in]
            n817 = call "TDMSbuffersize.vi"("error in (no error)"=w1704, "group names"=w1700, "Data Value Reference in"=w1703) -> ("error out"=w1699:errorcluster, "Data Value Reference out"=w1702:refnum<k34>)  [unwired: 7 in]
            n818 = Bundle By Name(cluster=w1707, "Data Value Reference out"=w1702) -> (w1706:T36)
          }
          frame "Center" {
            # "Your code here.\n(You can make a copy of, or modify, this frame)"
            n819 = control-ref of="image::1"() -> (w1736:refnum<vi>)
            n820 = control-ref of="image::2"() -> (w1735:refnum<vi>)
            n821 = control-ref of="image::3"() -> (w1734:refnum<vi>)
            n822 = control-ref of="image::4"() -> (w1733:refnum<vi>)
            n823 = control-ref of="image::5"() -> (w1732:refnum<vi>)
            n824 = control-ref of="image::6"() -> (w1731:refnum<vi>)
            n825 = control-ref of="image::7"() -> (w1730:refnum<vi>)
            n826 = control-ref of="image::8"() -> (w1729:refnum<vi>)
            n827 = control-ref of="image::9"() -> (w1728:refnum<vi>)
            n828 = control-ref of="image::10"() -> (w1727:refnum<vi>)
            n829 = control-ref of="image::11"() -> (w1726:refnum<vi>)
            n830 = control-ref of="image::12"() -> (w1725:refnum<vi>)
            n831 = for {
              tunnel: [w1745] -> w1724 mode=indexing
              tunnel: w1723 -> [w1744] mode=indexing
              n832 = Unbundle By Name(w1744) -> ("Target.X::12"=w1743:refnum<vi>, "Target.Y::12"=w1742:refnum<vi>)
              n833 = property class="DigNum (strict)"(reference=w1743) -> ("Value"=w1746:dbl)  [unwired: 1 in, 2 out]
              n834 = property class="DigNum (strict)"(reference=w1742) -> ("Value"=w1747:dbl)  [unwired: 1 in, 2 out]
              n835 = Bundle("Value"=w1746, "Value"=w1747) -> (w1745:cluster{"Value":dbl, "Value":dbl})  [unwired: 1 in]
            }
            n836 = call <vilib>:"Add State(s) to Queue__jki_lib_state_machine.vi"("State(s) in (\"\")"=w1741) -> ("States Out"=w1740:string)  [unwired: 14 in]
            n837 = Build Array(w1736, w1735, w1734, w1733, w1732, w1731, w1730, w1729, w1728, w1727, w1726, w1725) -> (w1737:refnum<vi>[])
            n838 = for {
              tunnel: w1737 -> [w1749] mode=indexing
              tunnel: w1724 -> [w1748] mode=indexing
              n839 = property class="ImageControl"(reference=w1749, "Image Center Position"=w1748) -> ()  [unwired: 1 in, 2 out]
            }
            n840 = property on="Center" class="Bool (strict)"("Value"=FALSE ("Center")) -> ()  [unwired: 2 in, 2 out]
          }
          frame "ImgToAvg" {
            n841 = Decimal String To Number(string=w1756) -> (number=w1753:i32)  [unwired: 2 in, 1 out]
            n842 = Bundle By Name(cluster=w1755, "img to avg"=w1753) -> (w1754:T36)
            n843 = call <vilib>:"Add State(s) to Queue__jki_lib_state_machine.vi"("State(s) in (\"\")"=w1752) -> ("States Out"=w1751:string)  [unwired: 14 in]
          }
          frame "history" {
            # "Your code here.\n(You can make a copy of, or modify, this frame)"
            n844 = Unbundle By Name(w1766) -> ("Offset X"=w1772:dbl[][], "Offset Y"=w1771:dbl[][], "Mean Centroid X"=w1770:dbl[][], "Mean Centroid Y"=w1769:dbl[][], "Motor X"=w1768:dbl[][], "Motor Y"=w1767:dbl[][], "Time"=w1758:timestamp[][])
            n845 = for {
              tunnel: w1772 -> [w1790] mode=indexing
              tunnel: w1771 -> [w1788] mode=indexing
              tunnel: w1770 -> [w1787] mode=indexing
              tunnel: w1769 -> [w1786] mode=indexing
              tunnel: w1768 -> [w1785] mode=indexing
              tunnel: w1767 -> [w1784] mode=indexing
              tunnel: [w1789] -> w1764 mode=indexing
              tunnel: [w1783] -> w1763 mode=indexing
              tunnel: [w1779] -> w1762 mode=indexing
              tunnel: [w1782] -> w1761 mode=indexing
              tunnel: [w1781] -> w1760 mode=indexing
              tunnel: [w1780] -> w1759 mode=indexing
              tunnel: w1758 -> [w1778] mode=indexing
              tunnel: [w1776] -> w1757 mode=indexing
              w1777 = 0
              n846 = Delete From Array(array=w1785, index=w1777) -> (array with subset deleted=w1781:dbl[])  [unwired: 1 in, 1 out]
              n847 = Delete From Array(array=w1784, index=w1777) -> (array with subset deleted=w1780:dbl[])  [unwired: 1 in, 1 out]
              n848 = Delete From Array(array=w1778, index=w1777) -> (array with subset deleted=w1776:timestamp[])  [unwired: 1 in, 1 out]
              n849 = Delete From Array(array=w1787, index=w1777) -> (array with subset deleted=w1779:dbl[])  [unwired: 1 in, 1 out]
              n850 = Delete From Array(array=w1786, index=w1777) -> (array with subset deleted=w1782:dbl[])  [unwired: 1 in, 1 out]
              n851 = Delete From Array(array=w1788, index=w1777) -> (array with subset deleted=w1783:dbl[])  [unwired: 1 in, 1 out]
              n852 = Delete From Array(array=w1790, index=w1777) -> (array with subset deleted=w1789:dbl[])  [unwired: 1 in, 1 out]
            }
            n853 = call <vilib>:"Add State(s) to Queue__jki_lib_state_machine.vi"("State(s) in (\"\")"=w1775) -> ("States Out"=w1774:string)  [unwired: 14 in]
            n854 = Bundle By Name(cluster=w1766, "Offset X"=w1764, "Offset Y"=w1763, "Mean Centroid X"=w1762, "Mean Centroid Y"=w1761, "Motor X"=w1760, "Motor Y"=w1759, "Time"=w1757) -> (w1765:T36)
          }
        }
        n855 = property on="Box" class="Arr (strict)"() -> ("Value"=w135:T6)  [unwired: 2 in, 2 out]
        n856 = for {
          tunnel: w137 -> [w158]
          tunnel: w136 -> [w159]
          tunnel: w133 -> [w151] mode=indexing
          tunnel: w135 -> [w152] mode=indexing
          n857 = call-poly <userlib>:"Filter 1D Array__ogtk.vi"("items to filter"=w151, "array"=w159) -> ("filtered item indices"=w160:i32[])  [unwired: 4 in, 1 out]
          n858 = Index Array(array=w160) -> (element=w154:i32)  [unwired: 1 in]
          n859 = Index Array(array=w158, index=w154) -> (element=w157:T30)
          n860 = Unbundle By Name(w157) -> ("Target.X::12"=w162:refnum<vi>, "Target.Y::12"=w161:refnum<vi>)
          n861 = property class="DigNum (strict)"(reference=w162) -> ("Value"=w156:dbl)  [unwired: 1 in, 2 out]
          n862 = property class="DigNum (strict)"(reference=w161) -> ("Value"=w155:dbl)  [unwired: 1 in, 2 out]
          n863 = call "draw crosshair imaq.vi"("Color"=u32 16774656, "Target.Y"=w155, "size"=cluster{"xhair size":dbl, "xhair size 2":dbl} {"xhair size"=25.0, "xhair size 2"=25.0}, "Target.X"=w156, "Bounding Rectangle"=T14 {"Left"=0, "Top"=0, "Right"=0, "Bottom"=0}, "image in"=w151) -> ("image out"=w150:T9)  [unwired: 4 in, 1 out]
          n864 = call "draw box imaq.vi"("Color"=u32 1244928, "Rectangle"=w152, "image in"=w150) -> ()  [unwired: 8 in, 1 out]
        }
      }
      n865 = control-ref of="This Application"() -> (w123:refnum<vi>)
      n866 = control-ref of="This VI"() -> (w127:refnum<vi>)
      n867 = Current VI's Menubar() -> (w126:refnum<k9>)
      n868 = call "GUI_Master_subvi_reentrant_queues.vi"("This Application"=w123, "error in (no error)"=w124, "tcp data event"=w122, "Caller menu reference"=w126, "Caller VI ref"=w127) -> ("error out"=→"error IO 2":errorcluster)  [unwired: 6 in]
      n869 = Unbundle By Name(w66) -> ("Data Value Reference out"=w65:refnum<k34>)
      n870 = for {
        tunnel: w95 -> [w131] mode=indexing
        tunnel: w94 -> [w130]
        tunnel: [w129] -> w64
        n871 = call "IMAQ Dispose"("Image"=w131, "error in (no error)"=w130) -> ("error out"=w129:errorcluster)  [unwired: 4 in]
      }
      n872 = TDMS Close(8:w64, 11:w65) -> (0:→"error out 2":errorcluster)  [unwired: 1 out]
      "Names" <- w34
    }
  }
